vi "LabviewImageProcess - red_tweezers_interface_linegen - test_edited for seq order-10-10 - Copy.vi"() -> ()   [LabVIEW 2015]
doc: "This is the interface, the one VI which loads all the others. Run this one first.\n\n(the line below ensures settings are saved)\n[Red Tweezers Save Settings]"
uses:
  subvis/line_trapping.ctl
  subvis/spot.ctl
  <vilib>/userdefined/High Color/IMAQdx.ctl
  subvis/selection_element.ctl
  subvis/mouse_info.ctl
  <vilib>/Analysis/baseanly.llb/Real A x B.vi
  subvis/red_tweezers_globals_INTERNAL_VOLATILE.vi
  subvis/red_tweezers_globals.vi
  <vilib>/Analysis/NI_AALBase.lvlib
  <vilib>/vision/driver/NI_Vision_Acquisition_Software.lvlib
  <vilib>/vision/NI_Vision_Development_Module.lvlib
panel:
  out "Spot Storage":T1[](array[typedef]) {"Amplitude Correction" step=0.1; "Line Trapping"."Phase Gradient" step=0.05; "Line Trapping"."Vector"."x" step=1e-06 format="%#_6p"; "Line Trapping"."Vector"."y" step=1e-06 format="%#_6p"; "Line Trapping"."Vector"."z" step=1e-06 format="%#_6p"; "NA Position"."r" step=1e-06; "NA Position"."y" step=1e-06; "NA Position"."x" step=1e-06; "Position"."z" step=1e-06; "Position"."y" step=1e-06; "Position"."x" step=1e-06; "Phase" step=0.7753; "Intensity" step=0.1}
  out "# selected":i16
  out "Last Pattern":T1[](array[typedef]) {"Amplitude Correction" step=0.1; "Line Trapping"."Phase Gradient" step=0.05; "Line Trapping"."Vector"."x" step=1e-06 format="%#_6p"; "Line Trapping"."Vector"."y" step=1e-06 format="%#_6p"; "Line Trapping"."Vector"."z" step=1e-06 format="%#_6p"; "NA Position"."r" step=1e-06; "NA Position"."y" step=1e-06; "NA Position"."x" step=1e-06; "Position"."z" step=1e-06; "Position"."y" step=1e-06; "Position"."x" step=1e-06; "Phase" step=0.7753; "Intensity" step=0.1}
  out "Plugins":T3(array[cluster])=[{"Name"="ASI Stage", "Folder"=path "C:/Users/Richard Bowman/Dropbox/red_tweezers_1_4_rc4/plugins/ASI Stage.llb", "vi reference"=refnum, "Needs to be run"=TRUE, "Error"={"status"=FALSE, "code"=0, "source"=""}}, {"Name"="iTweezers", "Folder"=path "C:/Users/Richard Bowman/Dropbox/red_tweezers_1_4_rc4/plugins/iTweezers.llb", "vi reference"=refnum, "Needs to be run"=TRUE, "Error"={"status"=FALSE, "code"=0, "source"=""}}, {"Name"="MightexLED", "Folder"=path "C:/Users/Richard Bowman/Dropbox/red_tweezers_1_4_rc4/plugins/MightexLED.llb", "vi reference"=refnum, "Needs to be run"=TRUE, "Error"={"status"=FALSE, "code"=0, "source"=""}}]
  in  "Tab":T4(tab)
  out "Y":dbl
  out "X":dbl
  in  "O Button":bool
  in  "OK Button":bool
  in  "Bubble Size":dbl=50.0002
  out "Hit Indicator":bool
  in  "On":bool
  out "Induce check":bool
  out "Area+ Buffer":dbl
  in  "Area to check":dbl=0.00025
  out "Prev Current Spot":dbl
  out "spots selected 2":i32=4
  out "Spot # Check":dbl
  out "Orig Y SC":dbl
  out "Orig X SC":dbl
  out "ID num check":dbl
  out "Value Check":dbl
  out "ID":dbl[](array[numeric])
  out "Null array":dbl[](array[numeric])
  out "Potential Collisions":dbl
  out "What to Check":dbl[](array[numeric])
  out "String counter":dbl
  out "Counter for String":dbl
  out "Numeric 4":dbl
  out "LCounter":dbl
  out "Numeric 3":dbl
  out "Num":dbl
  out "Old Y":dbl
  out "Old X":dbl
  out "init":dbl
  out "Looper":bool
  in  "Output to SLM":bool
  out "Maximum":dbl
  out "Projected Distance":dbl
  out "Previous Distance":dbl
  out "Group ID #":dbl
  in  "Buffer Zone":dbl=7e-05
  out "# of Spots":dbl
  out "Distance":dbl
  out "Hit":bool
  out "Y Displacement":dbl
  out "X Displacement":dbl
  out "Current Spot #":dbl
  out "spots selected":i32=4
  in  "lock aspect ratio":bool=TRUE
  in  "Size":cluster{"x":dbl, "y":dbl, "z":dbl} {"z" step=1e-06 format="%#_4p"; "y" step=1e-06 format="%#_4p"; "x" step=1e-06 format="%#_4p"}
  in  "Position":cluster{"x":dbl, "y":dbl, "z":dbl}={"x"=1e-06, "y"=-6.3e-06, "z"=0.0} {"z" step=1e-06 format="%#_4p"; "y" step=1e-06 format="%#_4p"; "x" step=1e-06 format="%#_4p"}
  in  "phase":dbl step=0.7753
  in  "Vortex Charge":i8
  in  "Intensity":dbl=1.0 step=0.1
  in  "add to selection":bool
  in  "random position":bool
  in  "new spot":bool
  in  "delete":bool
  in  "rotate":bool
  in  "Rotation Axis":u16(ring)=2 items=["Z", "X", "Y", "Custom"]
  in  "Angle (degrees)":dbl=2.0
  in  "Custom Axis":cluster{dbl, dbl, dbl}
  in  "Spot Shape":enum32{"Normal", "Line", "NA", "Mixed"}(tab)=enum."Mixed"
  in  "Line Trapping":T2 {"Phase Gradient" step=0.05; "Vector"."x" step=1e-06 format="%#_4p"; "Vector"."y" step=1e-06 format="%#_4p"; "Vector"."z" step=1e-06 format="%#_4p"}
  in  "Scale back aperture":dbl=1.1 step=0.1
  in  "Scale BA":bool
  in  "Position on back aperture":cluster{"x":dbl, "y":dbl}={"x"=-5.84327907697451e-18, "y"=0.0} {"y" step=0.1 format="%#_4p"; "x" step=0.1 format="%#_4p"}
  in  "Radius on back aperture":dbl=1.1 step=0.1
  in  "Generate":bool
  in  "Pattern":T5(tab)
  in  "Spots across centre":i32=5
  in  "Reference Array?":bool
  in  "Fraction of SLM":dbl=1.0
  in  "Spots across centre":i32=5
  in  "N":cluster{i32, i32}
  in  "spacing/m":dbl=2.0
  in  "Iterations":i32=10
  out "non-uniformity":dbl(slide)=0.031119223416512406 scale=0.0..0.2
  out "efficiency":dbl(slide)=0.8985936267644501 scale=0.0..1.0
  in  "Optimise":bool
  in  "Reset Phase/Amplitude":bool
  in  "Fall-off/m":dbl=0.00025 min=0.0 step=1e-06 format="%#_4p"
  in  "Abort Plugin":bool
  in  "Plugin:":u16(ring)=1 items=["ASI Stage", "iTweezers", "MightexLED"]
  in  "Save Video":bool
  in  "Global ROI (requires restart)":i32[](array[numeric])=[0, 0, 1280, 512]
  in  "Zoom":bool
  in  "Draw ROI":bool
  in  "Zoom to Fit":bool
  out "Image Information":string="640x480 1.93X 8-bit image 255    (0,0)"
  in  "Camera":T6
  in  "Time per Frame (ms)":dbl
  in  "Edit Sequence Mode":bool
  in  "Manual Edit":bool
  in  "Bubble ID to Empty":dbl
  in  "Clearance Button":bool
  in  "Manual Sequence":bool
  in  "Play Sequence":bool
  in  "Reset":bool
  out "Sequence Instances":dbl
  out "Counter":dbl
  in  "Save State":bool
  out "Sequence On?":bool
  in  "Sequence Order":dbl
  out "Selection/Group":T7[](array[typedef])
  in  "Sequence Storer":T1[][](array[typedef]) {"Amplitude Correction" step=0.1; "Line Trapping"."Phase Gradient" step=0.05; "Line Trapping"."Vector"."x" step=1e-06 format="%#_6p"; "Line Trapping"."Vector"."y" step=1e-06 format="%#_6p"; "Line Trapping"."Vector"."z" step=1e-06 format="%#_6p"; "NA Position"."r" step=1e-06; "NA Position"."y" step=1e-06; "NA Position"."x" step=1e-06; "Position"."z" step=1e-06; "Position"."y" step=1e-06; "Position"."x" step=1e-06; "Phase" step=0.7753; "Intensity" step=0.1}
  in  "Rates":bool
  out "Rates":dbl
  out "LCS":dbl
  in  "Add Additional Frames":bool
  in  "Frame Location":dbl
  in  "Additional Frames Wanted":dbl
  in  "Initiate Creation":bool
  in  "Number of Planned Sequence Frames":dbl
  in  "Max Number of Bubbles":dbl
  in  "Tab Control":enum32{"Line", "Arc"}(tab)
  out "X Rate":dbl
  out "Y Rate":dbl
  out "Degree Rate":dbl
  out "Radians":dbl
  out "Center Y":dbl
  out "Center X":dbl
  in  "Radius X":dbl
  in  "Theta":dbl
  in  "Lock Current Spot":bool
  out "Locked Current Spot":dbl
  out "Numeric":dbl
  out "probe":dbl
  in  "Insert":bool
  in  "Start at Which Frame?":dbl
  out "Original Y":dbl
  out "Original X":dbl
  in  "Mark Original Position":bool
  in  "How Many Frames?":dbl
  out "New Y":dbl
  out "New X":dbl
  out "Spot Storage 2":T1[](array[typedef]) {"Amplitude Correction" step=0.1; "Line Trapping"."Phase Gradient" step=0.05; "Line Trapping"."Vector"."x" step=1e-06 format="%#_6p"; "Line Trapping"."Vector"."y" step=1e-06 format="%#_6p"; "Line Trapping"."Vector"."z" step=1e-06 format="%#_6p"; "NA Position"."r" step=1e-06; "NA Position"."y" step=1e-06; "NA Position"."x" step=1e-06; "Position"."z" step=1e-06; "Position"."y" step=1e-06; "Position"."x" step=1e-06; "Phase" step=0.7753; "Intensity" step=0.1}
  in  "Save":bool
  in  "Load":bool
  in  "Camera Capture":bool
  out "Bubble y":dbl
  out "Bubble x":dbl
  out "Number of Matches Returned":dbl
  out "bottomry":dbl
  out "toply":dbl
  out "bottomrx":dbl
  out "toplx":dbl
  in  "Send Data":bool
  out "Camera 2":T8(plugin-control)
  out "Circles":T9(array[cluster]) {"Position"."Y" format="%.2f"; "Position"."X" format="%.2f"}
  out "Video Frame Rate":dbl(knob)=50.00000000000003 scale=0.0..100.0 scale format="%.1f"
  out "Interface Frame Rate":dbl(knob)=97.23240312927678 scale=0.0..100.0 scale format="%.1f"
  in  "stop":bool=TRUE
  out "1 for original positon":dbl
  out "MOP pressed":bool
  out "MOP pressed After":bool
  out "X Pos every 10 sec":dbl
  out "Elapsed Time":dbl
  out "Sequence Frames To Check":string
  out "Position Indicator":string
  in  "Clear String":bool
  out "String 2":string
  out "Collision Detector":string
  out "Array":dbl[](array[numeric])
  out "Spot Checker":T1[](array[typedef]) {"Amplitude Correction" step=0.1; "Line Trapping"."Phase Gradient" step=0.05; "Line Trapping"."Vector"."x" step=1e-06 format="%#_6p"; "Line Trapping"."Vector"."y" step=1e-06 format="%#_6p"; "Line Trapping"."Vector"."z" step=1e-06 format="%#_6p"; "NA Position"."r" step=1e-06; "NA Position"."y" step=1e-06; "NA Position"."x" step=1e-06; "Position"."z" step=1e-06; "Position"."y" step=1e-06; "Position"."x" step=1e-06; "Phase" step=0.7753; "Intensity" step=0.1}
  out "Image":T8(plugin-control)
  # "Notes:\n\nIf you are doing non-sequence controls,\nthe delete function can be used as intended.\nHowever, do not use the delete function after\nrunning a sequence! Using it will prevent\nthe bubbles from appearing as the\nnumber of spots will change, which is\nessential for the sequence to work (it would\nbe displaying the maximum number of\nbubbles). \n\nIf you happen to delete a bubble, it can be \nrestored by inserting a new spot. Once enough\nspots have been restored, click on manual edit\nto correct the # of spots tracker. It should \nbe restored to where it originally was."
  # "The SLM can be used to shape spots; here you can restrict the NA of a spot (so it comes only from part of the back aperture), or create a line-trap"
  # "The traps do not have any spot-shaping applied (so they should just be diffraction-limited focal spots)."
  # "This shapes the amplitude (and phase) of the beam to create extended line traps.  The \"Phase Gradient\" control allows the Poynting vector to push things along the line.  Unfortunately, some work is needed on the scaling factors so the phase gradient control will need tweaking if the line trap has a nonzero z component."
  # "By default,each spot comes from the whole back aperture.  Here, you can limit a spot to come from a specific part of the back aperture."
  # "The control below allows you to scale the whole back aperture (i.e. the position and size of all the apertures).  It's a one-time operation, i.e. only changes things when you push \"ok\"."
  # "A Combination of line-trapping and NA restriction has been applied to these traps.  You can get at the line trap or NA parameters on the other tabs, switching to the NA tab does not delete the line-trap settings."
  # "This tab generates Shack-Hartmann type holograms, which are often useful when aligning the system, and arrays of spots."
  # "The controls above only work when using the \"IMAQdx with ROI Buttons\" case in the bottom loop.  You can save video regardless of camera code though."
  # "Manual Edit allows a user to\ngo to a specific sequence frame."
  # "To clear the sequence, you must\nclear the array. Right click on sequence\nstorer to do this."
  # "Use this to \"clear\" a \nspecific bubble. If\nworking on a sequence,\nuse this as your delete\nbutton! You can update\nthe view by using manual edit."
  # "Use the reset button\nto clear counter.\nIt becomes necessary\nwhen you clear the array,\nespecially in manual mode."
  # "Use the sequence creator tab to specify the\nnumber of bubbles you want along with\nthe number of frames.\n\nTo save at a specific interval, the sequence\norder can be used to place the state. If used\nto correct something, it will replace the\nentire sequence frame.\n\n\"Sequence On?\" is only used in auto mode."
  # "Frame Location must be\nwhere you want to add\nthe frames to (ie having \n4 as an input would have\nthe additional frames\nstart at array row 5."
  # "Multiple bubbles can  be done with the\nline function. One bubble at a time for the arc\nfunction."
  # "Using the Load/Save function:\n\nRed Tweezers itself is unable to save long \nsequences, but a separate program is able to\naccomplish this. To do this, follow these\nsteps:\n\n1. After creating your sequence, press the save\nbutton below.\n\n2. Then, go to the subvi folder and find\nSequenceSaver.vi.\n\n3. At the control \"Sequence Storer,\" right-click\nthe dimensions part of the array and go to\ndata operations.\n\n4. Press \"Make Current Values Default\" and save\nthe sequence.\n\n5. The next time you load the program, simply\npress load to re-acquire the sequence. You\nwill need to insert the bubbles again, but after\nthe first frame can be recovered by using\nSequenceControl.vi."
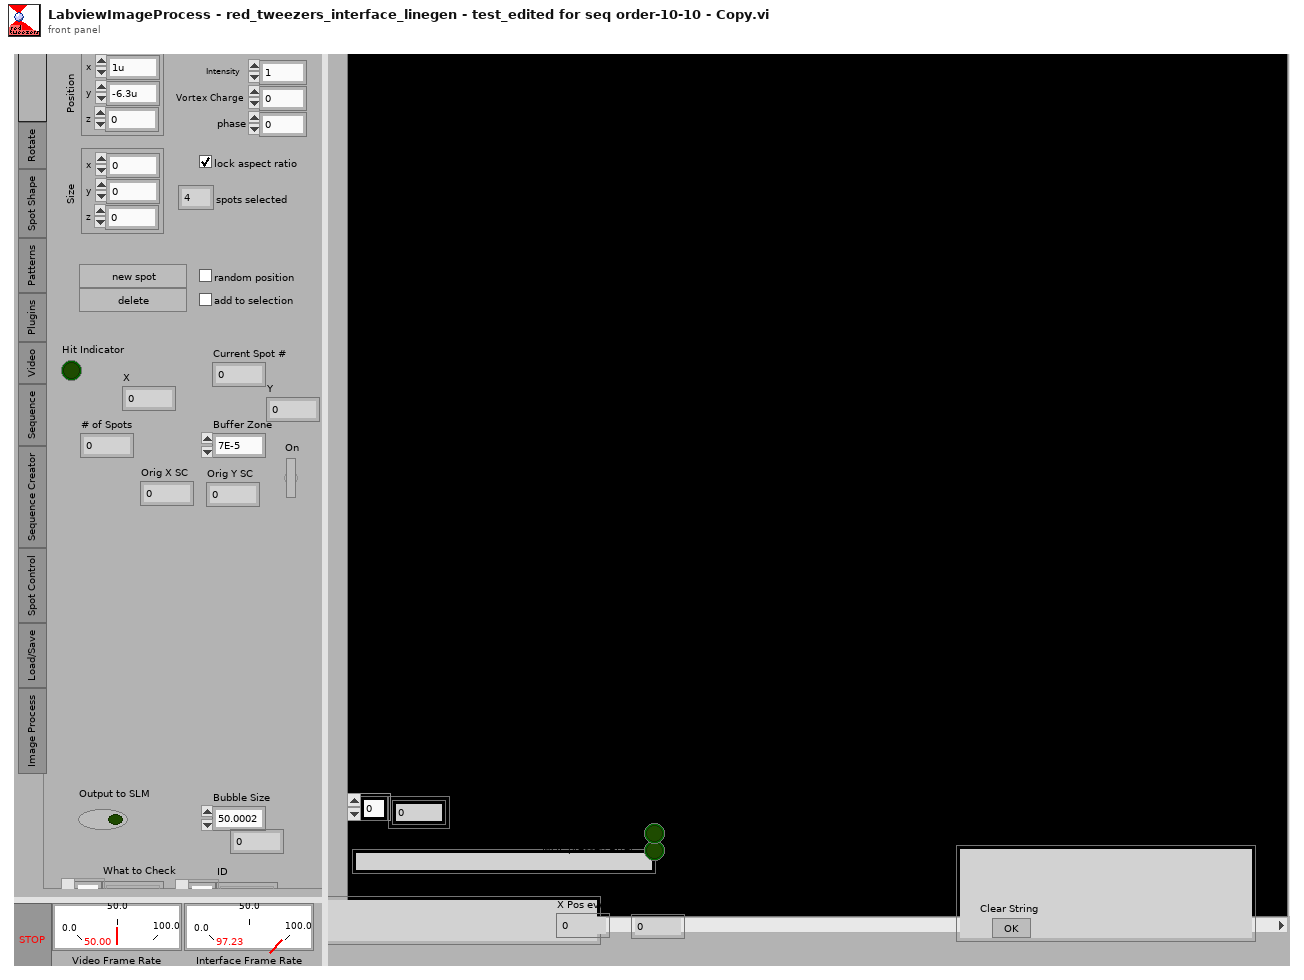
[diagram p1: front panel]
types:
  T1 = typedef "spot.ctl" = cluster{"Position":cluster{"x":dbl, "y":dbl, "z":dbl}, "Intensity":dbl, "Vortex Charge":i8, "Phase":dbl, "NA Position":cluster{"x":dbl, "y":dbl, "r":dbl}, "Line Trapping":T2, "Amplitude Correction":dbl}
  T2 = typedef "line_trapping.ctl" = cluster{"Vector":cluster{"x":dbl, "y":dbl, "z":dbl}, "Phase Gradient":dbl}
  T3 = cluster{"Name":string, "Folder":path, "vi reference":refnum<vi>, "Needs to be run":bool, "Error":errorcluster}[]
  T4 = enum32{"Current Spot", "Rotate", "Spot Shape", "Patterns", "Plugins", "Video", "Sequence", "Sequence Creator", "Spot Control", "Load/Save", "Image Process"}
  T5 = enum32{"HCP Shack-Hartmann", "Square Shack-Hartmann", "Rectangular Grid"}
  T6 = typedef "IMAQdx.ctl" = refnum<k21>
  T7 = typedef "selection_element.ctl" = cluster{"Group ID":i32, "Selected":bool}
  T8 = typedef "IMAQ Image.ctl" = refnum<image>
  T9 = cluster{"Position":cluster{"X":sgl, "Y":sgl}, "Radius":dbl, "Score":dbl}[]
  T10 = typedef "mouse_info.ctl" = cluster{"Button Down":bool, "Dragging":bool, "Position (Image Pixels)":cluster{"X":dbl, "Y":dbl}, "Previous Position (Image Pixels)":cluster{"X":dbl, "Y":dbl}, "Button":u16, "Mods":cluster{"Double Click":bool, "Menu Key":bool}, "PlatMods":cluster{"Shift":bool, "Ctrl":bool, "Alt":bool, "Cmd":bool, "Opt":bool}}
  T11 = cluster{"Position":cluster{"x":dbl, "y":dbl, "z":dbl}, "Intensity":dbl, "Vortex Charge":i8, "Phase":dbl, "NA Position":cluster{"x":dbl, "y":dbl, "r":dbl}, "Line Trapping":T2, "Amplitude Correction":dbl}
  T12 = enum16{"Set guide visibility", "Set grid visibility", "Show front panel", "Render on image"}
  T13 = enum32{"Current Spot", "Rotate", "Spot Shape", "Patterns", "Plugins", "Video"}
  T14 = enum16{"Left Button", "Center Button", "Right Button", "Window Close"}
  T15 = typedef "Image Type" = u32
  T16 = cluster{"number: 0 to 1":dbl, "number: 0 to 1":dbl}
  T17 = typedef "NI_Matrix.lvlib/RealMatrix.ctl" = dbl[][]
  T18 = typedef "overlay_element.ctl" = cluster{"Tool":enum16{"Lines", "Oval", "Rectangle", "Text"}, "Points":cluster{"X":dbl, "Y":dbl}[], "Drawing Mode":u32, "Color":u32, "String":string}
  T19 = enum32{"Current Spot", "Rotate", "Spot Shape", "Patterns", "Plugins", "Video", "Particle Tracking", "Clamping", "Blank"}[]
  T20 = typedef "LVMenuShortCut.ctl" = cluster{"include Shift key?":bool, "include Ctrl key?":bool, "shortcut key":string}
  T21 = typedef "LVPoint32TypeDef.ctl" = cluster{"Horizontal":i32, "Vertical":i32}
  T22 = cluster{"Shift":bool, "Ctrl":bool, "Alt":bool, "Cmd":bool, "Opt":bool}
  T23 = cluster{"Button Down":bool, "Dragging":bool, "Mouse Coords (image pixels)":cluster{dbl, dbl}, "Mouse Coords (image pixels)":cluster{dbl, dbl}, "Button":u16, "Mods":cluster{"Double Click":bool, "Menu Key":bool}, "PlatMods":cluster{"Shift":bool, "Ctrl":bool, "Alt":bool, "Cmd":bool, "Opt":bool}}
  T24 = cluster{"Position":cluster{"X":sgl, "Y":sgl}, "Radius":dbl, "Score":dbl}
  T25 = cluster{"[0]":dbl, "[1]":dbl, "[2]":dbl, "[3]":dbl}
  T26 = cluster{"Average Frame Time":dbl, "millisecond timer value":u32}
  T27 = cluster{"Position":cluster{"x":dbl, "y":dbl, "z":dbl}, "Intensity":dbl, "Vortex Charge":i8, "Phase":dbl, "NA Position":cluster{"x":dbl, "y":dbl, "r":dbl}, "Line Trapping":T2, "Amplitude Correction":dbl}[]
  T28 = enum32{"Bad", "Idle", "Run top level", "Running"}
  T29 = typedef "AviRefnum.ctl" = refnum<k1>
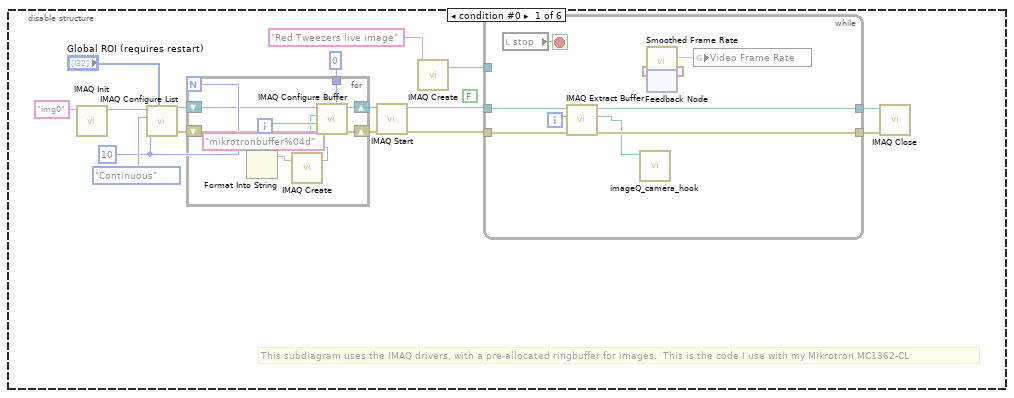
[diagram p3: hidden frame]
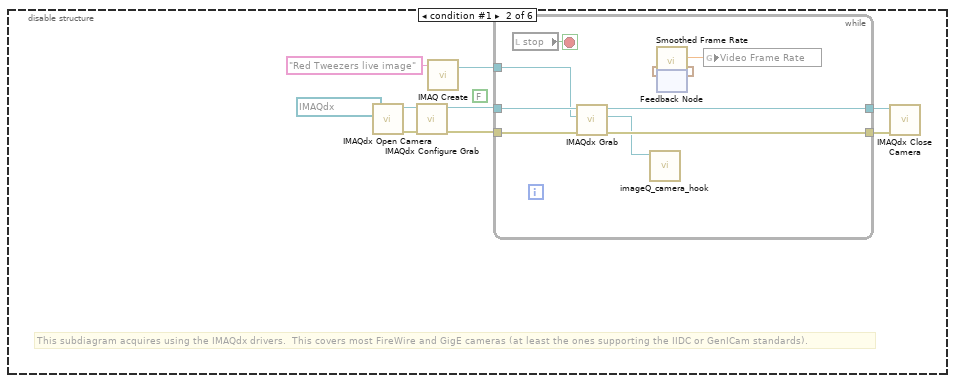
[diagram p4: hidden frame]
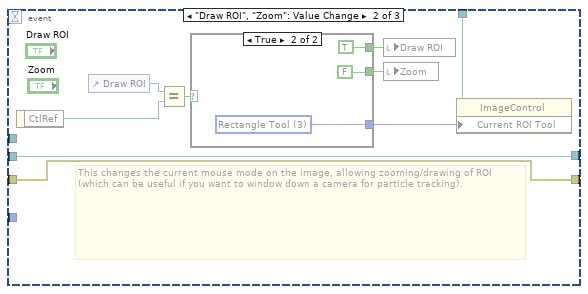
[diagram p5: hidden frame]
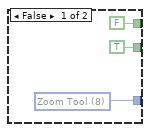
[diagram p6: hidden frame]
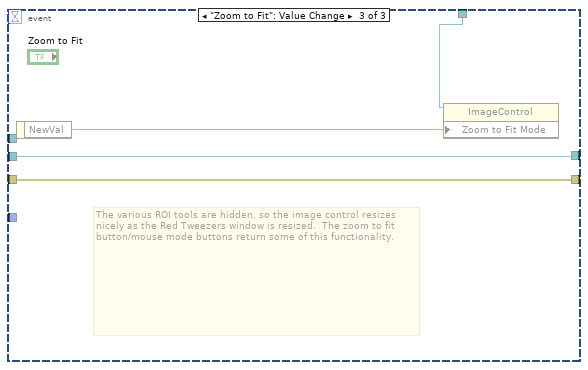
[diagram p7: hidden frame]
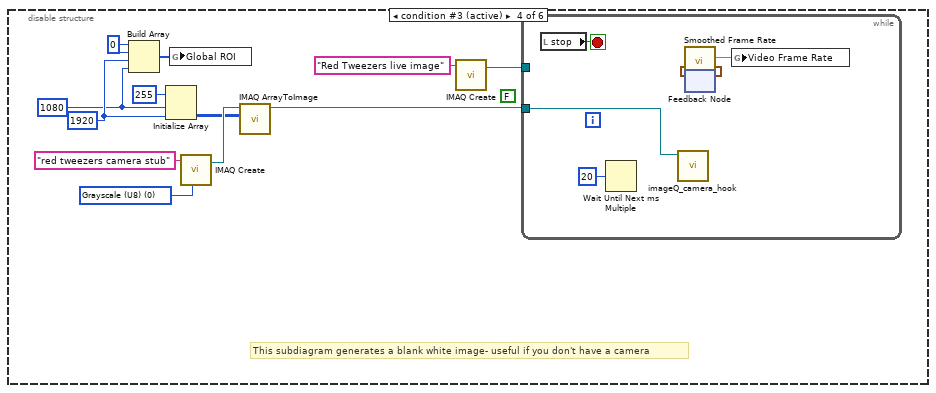
[diagram p8: hidden frame]
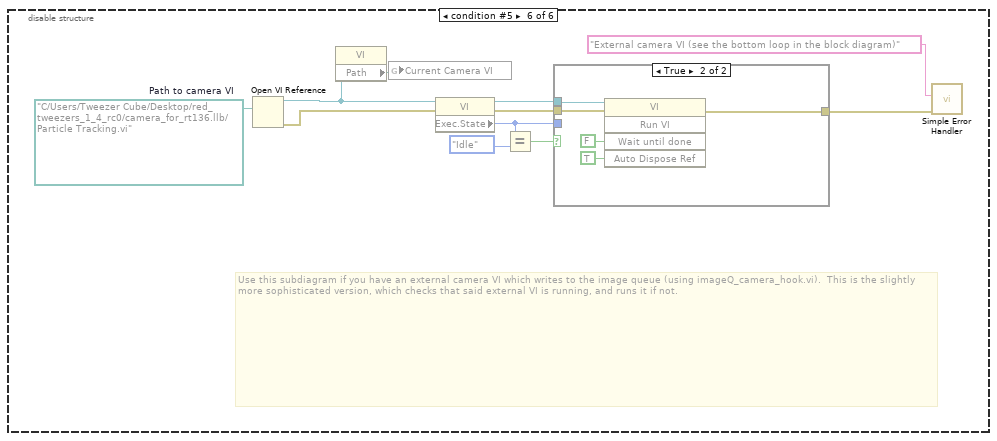
[diagram p10: hidden frame]
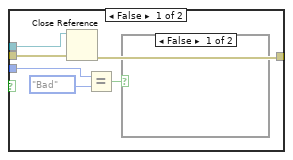
[diagram p11: hidden frame]
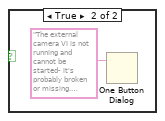
[diagram p12: hidden frame]
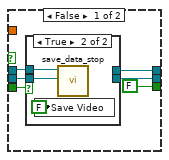
[diagram p13: hidden frame]
diagram:
  w11 = "red_tweezers_display_imageQ" ("Queue Name")
  w23 = T10 {"Button Down"=FALSE, "Dragging"=FALSE, "Position (Image Pixels)"={"X"=0.0, "Y"=0.0}, "Previous Position (Image Pixels)"={"X"=0.0, "Y"=0.0}, "Button"=0, "Mods"={"Double Click"=FALSE, "Menu Key"=FALSE}, "PlatMods"={"Shift"=FALSE, "Ctrl"=FALSE, "Alt"=FALSE, "Cmd"=FALSE, "Opt"=FALSE}}  # Mouse Information
  w24 = refnum<vi> refnum  # Image
  # "The funny looking feedback-node structure is deliberate (if odd).  We want to reload settings from the last used file (stored in the registry) only if this program has not been run since it was last loaded from file/recompiled.  That's why I use an uninitialised shift register: every time the program runs, it increments.  So, if it is zero, this is our first run (or we've been recently recompiled)."
  # "This loop handles the video that is displayed on-screen and saved to file."
  # "Initially, we only register to be told when the user clicks the image"
  # "This is the actual image control"
  # "This is a generic reference.\nIt is just a placeholder, so we can register for events later."
  # "This version of red tweezers uses two coordinate systems: \n1. Real Coordinates - corresponding to physical distances in 3D in microns\n2. Image Coordinates - position on the camera image, relative to the top left of the CURRENT ROI, measured in pixels. If the ROI changes, the relationship between \"real units\" and \"image pixels\" may change, so all values should be stored and presented to the user in REAL units unless there is a good reason to do otherwise."
  n1 = control-ref of="Plugin Pnl"() -> (w20:refnum<vi>)
  n2 = flat-sequence {
    tunnel: [w27] -> w6
    tunnel: w4 -> [_]
    frame #0 {
      n3 = vi-ref "red_tweezers_globals_INTERNAL.vi"() -> (w28:refnum<vi>)
      n4 = property class="VI"(reference=w28) -> ("Path"=w27:path)  [unwired: 1 in, 2 out]
      n5 = global write "red_tweezers_globals_INTERNAL_VOLATILE.vi" "Current Camera VI"(w27) -> ()
    }
  }
  n6 = control-ref of="Plugin:"() -> (w21:refnum<vi>)
  n7 = feedback #1() -> (w14:dbl)  [unwired: 1 in]
  n8 = Equal To 0?(x=w14) -> (x = 0?=w13:bool)
  n9 = Increment(x=w14) -> (x+1=w12:dbl)
  n10 = feedback-in #1(w12) -> ()
  n11 = call "plugins_load.vi"("Sub Panel"=w20, "Plugin Chooser"=w21) -> ("error out"=w15:errorcluster, "Plugins"=w17:T3)  [unwired: 2 in, 2 out]
  "Plugins" <- w17
  n12 = control-ref of="Image"() -> (w5:refnum<vi>)
  n13 = case shown="True" w13 {
    tunnel: w15 -> [_ w29]
    tunnel: [_ w29] -> w4
    frame False {
    }
    frame True {
      n14 = call "settings_load_default_file.vi"("error out"=w29) -> ()
    }
  }
  n15 = flat-sequence {
    tunnel: w4 -> [_]
    tunnel: w2 -> [w31]
    frame #0 {
      # "ensure we don't accidentally start saving video, and run UDP Sender to set up the hologram window."
      n16 = local write "Save Video"(FALSE ("background subtraction")) -> ()
      n17 = call "UDP Sender generic_2.vi"("Spots"=w31) -> ()  [unwired: 2 in, 1 out]
    }
  }
  n18 = global read "red_tweezers_globals.vi" "Selection/Group"() -> (w22:T7[])
  n19 = register-events(w5, w24, w24, w24) -> (reference out=w25:refnum<event-registration>)  [unwired: 2 in, 1 out]
  n20 = global read "red_tweezers_globals.vi" "Spots"() -> (w2:T1[])
  n21 = local write "stop"(FALSE ("STOP")) -> ()
  n22 = call "ensure_selection_matches_spots.vi"("Selection and Groups in"=w22, "Spots"=w2) -> ("Selection and Groups out"=w26:T7[], "Spots (duplicate)"=w1:T1[])  [unwired: 4 in]
  n23 = call "IMAQ Create"("Image Name"=w11) -> ("New Image"=w9:T8)  [unwired: 4 in, 1 out]
  n24 = call "imageQ_create_return_queue.vi"("Queue Name"=w11) -> ("queue out"=w10:refnum<queue>)
  n25 = while {
    shift-right: [w118] -> _
    shift-left: w1 -> [w138]
    shift-right: [w137] -> _
    shift-left: w26 -> [w136]
    shift-right: [w140] -> _
    shift-left: _ -> [w131]
    shift-right: [w139] -> _
    shift-left: _ -> [w130]
    tunnel: w5 -> [w135]
    shift-right: [w129] -> _
    shift-left: w23 -> [w128]
    shift-right: [w132] -> _
    shift-left: w25 -> [w133]
    border: errorcluster {"status"=FALSE, "code"=0, "source"=""} ("error out") -> [_]
    tunnel: [errorcluster {"status"=FALSE, "code"=0, "source"=""} ("error in (no error)")] -> w18
    border: w17 -> [_]
    tunnel: w1 -> [w119]
    stop <- w120 stop-if-true
    w34 = 1
    w42 = 7 items=["Red", "Green", "Blue", "Hue", "Saturation", "Luminance", "Value", "Intensity"] ("Color Plane")
    w46 = T15 0 items=["Grayscale (U8)", "Grayscale (I16)", "Grayscale (SGL)", "Complex (CSG)", "RGB (U32)", "HSL (U32)", "RGB (U64)", "Grayscale (U16)"] ("Image Type")
    # "Don't Need. For Matlab Part."
    # "The function inserts the newly generated sequence for the automatic sequence generator. It also contains the code\nthe code necessary to check whether the bubbles will intersect with each other in the sequence."
    # "This calculates the size of the area including the buffer zone length.\nThe bubble diameter will also be included in the near future."
    # "The statement to the right controls the area that are being chcecked and checks\nwhich bubbles need to be checked.  There are two instances where this activates\nin this case:\n\nWhen a new bubble is selected\nWhen a bubble is deselected, reverting to the last current spot #\n\nThe other case, when the bubble moves out of the area specified, is located\ninside the while loop controlling the bubble movement with a mouse."
    # "Timer function example"
    # "These functions help with the calculations for the sequence generator."
    # "This loads the sequence from the \"saver\" VI. The save function below \"saves\" the sequence into the saver VI."
    # "The VI above is SequenceSaver.vi which contains the\ncode necessary to create a sequence."
    # "This case structure is the Save State structure. This stores\nthe current state of the bubbles (ie position)."
    # "Reset sets the counter back to zero. This is particularly useful \nwhen using the manual sequence."
    # "This case structure helps to continue the sequence.\nThis takes the true case of the Sequence On? function\nor the true case for the Manual Sequence function\nin order to go to the next sequence frame."
    # "This case structure allows for the playing of the sequence.\nThe amount of time it takes to go through the sequence\ncan be edited on the current spot menu."
    # "We only write to the image overlay when we are in one of the tabs, to prevent it disappearing when we are (for example) using the mouse."
    # "These wires control saving undo info. See the VI below's tip strips for details."
    # "Setting these wires to false means:\n(1) dragging moves the selection\n(2) clicking spots changes selection\nset them to true to stop the default mouse behaviour, don't wire them straight through!"
    n26 = event shown="[6] <Image>: Mouse Move" {
      selector: w133 -> [w550 w1222 w1227 w1449 w1477 w1494 w1591 _]
      dyn-events: [w550 w1221 w1227 w1447 w1474 w1495 w1591 _] -> w132
      timeout: 0 -> [_ _ _ _ _ _ _ _]
      tunnel: [w558 _ w1229 w1444 w1479 w1486 w1578 _] -> w140
      tunnel: [w557 _ w1228 w1443 w1478 w1485 w1582 _] -> w139
      tunnel: [w556 _ _ _ _ _ _ _] -> w91
      tunnel: w138 -> [w555 w1217 w1234 w1439 w1472 w1491 w1586 w1909]
      tunnel: [w554 w1217 w1232 w1439 w1472 w1482 w1584 w1909] -> w126
      tunnel: [w553 w1216 w1231 w1428 w1471 w1492 w1574 w1908] -> w125
      tunnel: w136 -> [w552 w1216 w1233 w1428 w1471 w1490 w1585 w1908]
      tunnel: w135 -> [w551 w1218 w1224 w1438 w1475 w1493 w1587 _]
      tunnel: [w549 _ w1226 w1448 T10 {"Button Down"=FALSE, "Dragging"=FALSE, "Position (Image Pixels)"={"X"=0.0, "Y"=0.0}, "Previous Position (Image Pixels)"={"X"=0.0, "Y"=0.0}, "Button"=0, "Mods"={"Double Click"=FALSE, "Menu Key"=FALSE}, "PlatMods"={"Shift"=FALSE, "Ctrl"=FALSE, "Alt"=FALSE, "Cmd"=FALSE, "Opt"=FALSE}} T10 {"Button Down"=FALSE, "Dragging"=FALSE, "Position (Image Pixels)"={"X"=0.0, "Y"=0.0}, "Previous Position (Image Pixels)"={"X"=0.0, "Y"=0.0}, "Button"=0, "Mods"={"Double Click"=FALSE, "Menu Key"=FALSE}, "PlatMods"={"Shift"=FALSE, "Ctrl"=FALSE, "Alt"=FALSE, "Cmd"=FALSE, "Opt"=FALSE}} w1590 _] -> w129
      tunnel: w128 -> [w549 _ w1226 _ _ w1489 w1581 _]
      tunnel: w131 -> [_ _ w1229 w1444 w1479 w1486 w1578 _]
      tunnel: w130 -> [_ _ w1228 w1443 w1478 w1485 w1582 _]
      tunnel: [w548 _ _ _ _ _ _ _] -> w127
      tunnel: [_ _ w1225 _ _ _ TRUE _] -> w124
      tunnel: [_ _ _ TRUE TRUE TRUE FALSE _] -> w123
      tunnel: [TRUE _ _ _ _ _ _ _] -> w121
      tunnel: [_ _ _ _ _ _ _ "stop"] -> w120
      tunnel: w119 -> [_ _ _ _ _ _ w1575 _]
      event Timeout {
        n27 = event-data() -> ()  [unwired: 1 in, 1 out]
        n28 = case shown="\"Current Spot\", Default" "Tab" {
          tunnel: [w574 w842 w989 w1091 w1172 w1210] -> w554
          tunnel: w555 -> [w571 w844 w990 w1093 w1172 w1210]
          tunnel: w552 -> [w560 w843 w987 w1092 w1171 w1209]
          tunnel: [w573 w841 w988 w1090 w1171 w1209] -> w553
          tunnel: [w561 _ TRUE _ _ _] -> w558
          tunnel: [w561 _ _ _ _ _] -> w557
          tunnel: [_ _ _ FALSE _ _] -> w556
          tunnel: w551 -> [_ _ _ _ _ w1206]
          tunnel: w549 -> [_ _ w969 _ _ _]
          tunnel: [_ _ w971 _ _ _] -> w548
          frame "Current Spot", Default {
            w561 = FALSE
            # "The function below contains the code necessary to use the automatic sequence generator to create specific movements. It also helps translate cases where the point is entered in not dragged.\nThis prevents bubbles from intersecting if the bubble is told not to intersect."
            # "If it's out of date, update front panel"
            n29 = call "find_centroid.vi"("Selection and Groups"=w560, "Spots"=w571) -> ("Mean Values"=w569:T1, "size"=w563:cluster{"x":dbl, "y":dbl, "z":dbl}, "centroid"=w564:cluster{"x":dbl, "y":dbl, "z":dbl}, "# selected"=w562:i16)  [unwired: 2 in, 1 out]
            n30 = stacked-sequence {
              tunnel: w562 -> [_ w576]
              frame #0 {
                n31 = local read "spots selected"() -> (→"spots selected 2":i32)
              }
              frame #1 {
                "spots selected" <- w576
              }
            }
            n32 = feedback-in #2(w569) -> ()
            n33 = feedback #2() -> (w570:T1)  [unwired: 1 in]
            n34 = feedback #3() -> (w568:cluster{"x":dbl, "y":dbl, "z":dbl})  [unwired: 1 in]
            n35 = feedback-in #3(w563) -> ()
            n36 = Not Equal?(x=w570, y=w569) -> (x != y?=w567:bool)
            n37 = Not Equal?(x=w568, y=w563) -> (x != y?=w566:bool)
            n38 = Or(x=w567, y=w566) -> (x .or. y?=w565:bool)
            n39 = case shown="True" w565 {
              tunnel: w569 -> [_ w582]
              tunnel: w563 -> [_ w578]
              frame False {
              }
              frame True {
                n40 = Unbundle By Name(w582) -> ("Position"=w577:cluster{"x":dbl, "y":dbl, "z":dbl}, "Intensity"=w580:dbl, "Vortex Charge"=w579:i8, "Phase"=w581:dbl)
                n41 = local write "Size"(w578) -> ()
                n42 = local write "Vortex Charge"(w579) -> ()
                n43 = local write "Intensity"(w580) -> ()
                n44 = local write "Position"(w577) -> ()
                n45 = local write "phase"(w581) -> ()
                n46 = Unbundle By Name(w577) -> ()  [unwired: 2 out]
              }
            }
            n47 = local write "Selection/Group"(w560) -> ()
            n48 = event shown="[3] \"Position\": Value Change" {
              selector: _ -> [_ _ _ _ _ _ _ _]
              dyn-events: _ -> [_ _ _ _ _ _ _ _]
              timeout: 10 -> [_ _ _ _ _ _ _ _]
              tunnel: w571 -> [w584 w588 w602 w625 w729 w774 w800 w823]
              tunnel: w560 -> [w583 w587 w605 w632 w716 w771 w797 w821]
              tunnel: [w584 w586 w603 w624 w717 w772 w798 w822] -> w574
              tunnel: [w583 w585 w604 w632 w716 w771 w797 w821] -> w573
              tunnel: w564 -> [_ _ _ _ w728 _ _ _]
              event Timeout {
                n49 = event-data() -> ()  [unwired: 3 out]
              }
              event "delete": Value Change {
                n50 = event-data() -> ()  [unwired: 7 out]
                n51 = call "delete_selected_spots.vi"("Selection/Group 3"=w587, "Spots 3"=w588) -> ("Selection/Group 2"=w585:T7[], "Spots 2"=w586:T1[])  [unwired: 4 in]
              }
              event "new spot": Value Change {
                # "If we're not adding it to the selection, de-select all the other spots"
                n52 = event-data() -> ()  [unwired: 7 out]
                n53 = call "coords_ROI_currentimage.vi"() -> ("Mono ROI"=w589:i32[])
                n54 = case shown="False" "add to selection" {
                  tunnel: w605 -> [w618 w623]
                  tunnel: [w617 w623] -> w600
                  frame False {
                    n55 = for {
                      tunnel: w618 -> [w621] mode=indexing
                      tunnel: [w622] -> w617 mode=indexing
                      n56 = Unbundle(w621) -> ("Group ID"=w620:i32)  [unwired: 1 out]
                      n57 = Bundle(cluster=w621, "Group ID"=w620, "Selected"=FALSE ("Label.Visible")) -> (w622:T7)
                    }
                  }
                  frame True {
                  }
                }
                n58 = Index Array(array=w589) -> (element #1=w595:i32, element #2=w596:i32, element #3=w594:i32, element #4=w593:i32)  [unwired: 4 in]
                n59 = Bundle("Numeric"=w595, "Numeric"=w596) -> (w590:cluster{"Numeric":i32, "Numeric":i32})  [unwired: 1 in]
                n60 = Bundle("Numeric"=w594, "Numeric"=w593) -> (w592:cluster{"Numeric":i32, "Numeric":i32})  [unwired: 1 in]
                n61 = Subtract(x=w592, y=w590) -> (x-y=w591:cluster{"Numeric":i32, "Numeric":i32})
                n62 = case shown="True" "random position" {
                  tunnel: [w607 w613] -> w598
                  tunnel: w591 -> [_ w609]
                  tunnel: w590 -> [_ w608]
                  frame False {
                    n63 = call "replace_position.vi"("Position"=cluster{"x":dbl, "y":dbl, "z":dbl} {"x"=0.0, "y"=0.0, "z"=0.0}) -> ("Spot"=w607:T1)  [unwired: 1 in, 2 out]
                  }
                  frame True {
                    n64 = Random Number (0-1)() -> (number: 0 to 1=w615:dbl)
                    n65 = Random Number (0-1)() -> (number: 0 to 1=w616:dbl)
                    n66 = Bundle("number: 0 to 1"=w616, "number: 0 to 1"=w615) -> (w614:T16)  [unwired: 1 out]
                    n67 = Multiply(x=w614, y=w609) -> (x*y=w611:cluster{dbl, dbl})
                    n68 = Add(x=w611, y=w608) -> (x+y=w610:cluster{dbl, dbl})
                    n69 = call "coords_image_to_real_currentimage.vi"("Position (pixels on image)"=w610) -> ("Position (real coords)"=w612:cluster{dbl, dbl, "Z":dbl})  [unwired: 9 in]
                    n70 = call "replace_position.vi"("Position"=w612) -> ("Spot"=w613:T1)  [unwired: 1 in, 2 out]
                  }
                }
                n71 = Build Array (concatenate)(w602, w598) -> (w603:T1[])
                n72 = Build Array (concatenate)(w600, cluster{i32, "Label.Visible":bool} {0, "Label.Visible"=TRUE}) -> (w604:T7[])
              }
              event "Position": Value Change {
                # "If the position has changed, translate the spots"
                n73 = event-data() -> ("OldVal"=w630:cluster{"x":dbl, "y":dbl, "z":dbl}, "NewVal"=w631:cluster{"x":dbl, "y":dbl, "z":dbl})  [unwired: 5 out]
                n74 = flat-sequence {
                  tunnel: w632 -> [w636]
                  tunnel: w629 -> [w635]
                  tunnel: w625 -> [w634]
                  tunnel: [w633] -> w626
                  frame #0 {
                    n75 = for {
                      tunnel: w634 -> [w641] mode=indexing
                      tunnel: w636 -> [w638] mode=indexing
                      tunnel: [w640] -> w633 mode=indexing
                      tunnel: w635 -> [w639]
                      n76 = Unbundle(w638) -> ("Selected"=w637:bool)  [unwired: 1 out]
                      n77 = case shown="True" w637 {
                        tunnel: w641 -> [w642 w647]
                        tunnel: [w642 w646] -> w640
                        tunnel: w639 -> [_ w643]
                        frame False {
                        }
                        frame True {
                          n78 = call "extract_position.vi"("Spot"=w647) -> ("Position"=w644:cluster{"x":dbl, "y":dbl, "z":dbl})
                          n79 = Add(x=w644, y=w643) -> (x+y=w645:cluster{"x":dbl, "y":dbl, "z":dbl})
                          n80 = call "replace_position.vi"("Position"=w645, "Spot in"=w647) -> ("Spot"=w646:T1)  [unwired: 2 out]
                        }
                      }
                    }
                  }
                }
                n81 = Subtract(x=w631, y=w630) -> (x-y=w629:cluster{"x":dbl, "y":dbl, "z":dbl})
                n82 = local read "# of Spots"() -> (w628:dbl)
                n83 = stacked-sequence {
                  tunnel: w625 -> [_ w652 _]
                  tunnel: w626 -> [_ w651 _]
                  tunnel: w628 -> [_ w650 _]
                  tunnel: [_ _ w699] -> w627
                  tunnel: w626 -> [_ _ w698]
                  tunnel: w625 -> [_ _ w697]
                  tunnel: [_ _ w696] -> w624
                  frame #0 {
                    n84 = local write "Looper"(FALSE) -> ()
                    "init" <- 0
                  }
                  frame #1 {
                    n85 = for {
                      N: w650 -> [_]
                      tunnel: w652 -> [w657]
                      tunnel: w651 -> [w662]
                      stop <- w663 stop-if-true
                      n86 = local read "init"() -> (w656:dbl)
                      n87 = Index Array(array=w662, index=w656) -> (element=w661:T1)
                      n88 = Index Array(array=w657, index=w656) -> (element=w655:T1)
                      n89 = Unbundle By Name(w661) -> ("Position.x"=w660:dbl, "Position.y"=w659:dbl)
                      n90 = local read "# of Spots"() -> (w658:dbl)
                      n91 = Unbundle By Name(w655) -> ("Position.x"=→"Old X":dbl, "Position.y"=→"Old Y":dbl)
                      n92 = local write "New X"(w660) -> ()
                      n93 = local write "New Y"(w659) -> ()
                      n94 = stacked-sequence {
                        tunnel: w657 -> [w668 _]
                        tunnel: w660 -> [w667 _]
                        tunnel: w659 -> [w666 _]
                        tunnel: w658 -> [w665 _]
                        tunnel: w656 -> [w664 _]
                        frame #0 {
                          n95 = for {
                            N: w665 -> [_]
                            tunnel: w668 -> [w690]
                            tunnel: w667 -> [w689]
                            tunnel: w666 -> [w687]
                            tunnel: w664 -> [w672]
                            i -> [w674]
                            stop <- w673 stop-if-true
                            n96 = Index Array(array=w690, index=w674) -> (element=w691:T1)
                            n97 = Unbundle By Name(w691) -> ("Position.x"=w688:dbl, "Position.y"=w686:dbl)
                            n98 = Subtract(x=w689, y=w688) -> (x-y=w685:dbl)
                            n99 = Subtract(x=w687, y=w686) -> (x-y=w684:dbl)
                            n100 = Square(x=w685) -> (x^2=w683:dbl)
                            n101 = Square(x=w684) -> (x^2=w682:dbl)
                            n102 = local read "# of Spots"() -> (w676:dbl)
                            n103 = Add(x=w683, y=w682) -> (x+y=w681:dbl)
                            n104 = local read "Buffer Zone"() -> (w671:dbl)
                            n105 = Square Root(x=w681) -> (sqrt(x)=w680:dbl)
                            n106 = Multiply(x=2, y=w671) -> (x*y=w669:dbl)
                            n107 = Less?(x=w680, y=w669) -> (x < y?=w678:bool)
                            n108 = Not Equal?(x=w672, y=w674) -> (x != y?=w677:bool)
                            n109 = Equal?(x=w676, y=w674) -> (x = y?=w679:bool)
                            n110 = And(x=w677, y=w678) -> (x .and. y?=w675:bool)
                            "Looper" <- w675
                            n111 = Or(x=w675, y=w679) -> (x .or. y?=w673:bool)
                          }
                        }
                        frame #1 {
                          n112 = local read "Looper"() -> (w692:bool)
                          n113 = case shown="False" w692 {
                            frame False {
                              n114 = local read "init"() -> (w693:dbl)
                              n115 = Add(x=w693, y=1) -> (x+y=w695:dbl)
                              n116 = local write "init"(w695) -> ()
                            }
                            frame True {
                            }
                          }
                        }
                      }
                      n117 = local read "Looper"() -> (w663:bool)
                    }
                  }
                  frame #2 {
                    n118 = local read "Looper"() -> (w700:bool)
                    n119 = case shown="False" w700 {
                      tunnel: w698 -> [w704 _]
                      tunnel: w697 -> [_ w712]
                      tunnel: ["This is an acceptable entry." "ERROR: A bubble will intersect the buffer zone."] -> w699
                      tunnel: [w704 w712] -> w696
                      frame False {
                        n120 = local write "Looper"(FALSE) -> ()
                        n121 = local read "Current Spot #"() -> (w705:dbl)
                        n122 = Index Array(array=w704, index=w705) -> (element=w703:T1)
                        n123 = Unbundle By Name(w703) -> ("Position.x"=w702:dbl, "Position.y"=w701:dbl)
                        n124 = local write "New Y"(w701) -> ()
                        n125 = local write "New X"(w702) -> ()
                      }
                      frame True {
                        # "Restore original position"
                        n126 = local write "Looper"(FALSE) -> ()
                        n127 = local read "Old Y"() -> (w709:dbl)
                        n128 = local read "Old X"() -> (w710:dbl)
                        n129 = local read "Position"() -> (w708:cluster{"x":dbl, "y":dbl, "z":dbl})
                        n130 = Bundle By Name(cluster=w708, "x"=w710, "y"=w709) -> (w711:cluster{"x":dbl, "y":dbl, "z":dbl})
                        n131 = local write "Position"(w711) -> ()
                      }
                    }
                  }
                }
                "Position Indicator" <- w627
              }
              event "Size": Value Change {
                # "If we were constraining the aspect ratio, or preventing a divide by zero, the size control on the FP may be incorrect.  We refresh it in here to stop it displaying a wrong value."
                # "If the size has changed, scale the spots"
                n132 = event-data() -> ("OldVal"=w721:cluster{"x":dbl, "y":dbl, "z":dbl}, "NewVal"=w727:cluster{"x":dbl, "y":dbl, "z":dbl})  [unwired: 5 out]
                n133 = Not Equal?(x=w721, y=w727) -> (x != y?=w720:cluster{"x":bool, "y":bool, "z":bool})
                n134 = Divide(x=w727, y=w721) -> (x/y=w726:cluster{"x":dbl, "y":dbl, "z":dbl})
                n135 = Not Equal To 0?(x=w721) -> (x != 0?=w719:cluster{"x":bool, "y":bool, "z":bool})
                n136 = And(x=w720, y=w719) -> (x .and. y?=w718:cluster{"x":bool, "y":bool, "z":bool})
                n137 = Cluster To Array(cluster=w718) -> (array=w725:bool[])
                n138 = Cluster To Array(cluster=w726) -> (array=w724:dbl[])
                n139 = case shown="True" "lock aspect ratio" {
                  tunnel: w725 -> [w733 w750]
                  tunnel: w724 -> [w732 w748]
                  tunnel: [w730 w740] -> w723
                  frame False {
                    # "We are not constraining the aspect ratio here, so just check we're not introducing NAs"
                    n140 = for {
                      tunnel: w733 -> [w739] mode=indexing
                      tunnel: w732 -> [w735] mode=indexing
                      tunnel: [w737] -> w731 mode=indexing
                      n141 = Not A Number/Path/Refnum?(number/path/refnum=w735) -> (NaN/Path/Refnum?=w736:bool)
                      n142 = Compound Arithmetic op=AND(w739, invert w736) -> (w738:bool)
                      n143 = Select(t=w735, s=w738, f=1.0) -> (s? t:f=w737:dbl)
                    }
                    n144 = Array To Cluster(array=w731) -> (cluster=w730:cluster{"[0]":dbl, "[1]":dbl, "[2]":dbl})
                  }
                  frame True {
                    # "Pick the first element that changed and use it.  Also need to make sure (1) an element did change and (2) everything's valid (no divide by zeros)"
                    n145 = Search 1D Array(1D array=w750, element=TRUE) -> (index of element=w747:i32)  [unwired: 1 in]
                    n146 = Index Array(array=w748, index=w747) -> (element=w743:dbl)
                    n147 = Not A Number/Path/Refnum?(number/path/refnum=w743) -> (NaN/Path/Refnum?=w746:bool)
                    n148 = Less Than 0?(x=w747) -> (x < 0?=w745:bool)
                    n149 = Or(x=w746, y=w745) -> (x .or. y?=w744:bool)
                    n150 = Select(t=1.0, s=w744, f=w743) -> (s? t:f=w741:dbl)
                    n151 = Bundle("x"=w741, "x"=w741, "x"=w741) -> (w740:cluster{"x":dbl, "x":dbl, "x":dbl})  [unwired: 1 in]
                  }
                }
                n152 = for {
                  tunnel: w729 -> [w756] mode=indexing
                  tunnel: w716 -> [w753] mode=indexing
                  tunnel: [w755] -> w717 mode=indexing
                  tunnel: w723 -> [w754]
                  tunnel: w728 -> [w751]
                  n153 = Unbundle(w753) -> ("Selected"=w752:bool)  [unwired: 1 out]
                  n154 = case shown="True" w752 {
                    tunnel: w756 -> [w757 w765]
                    tunnel: [w757 w764] -> w755
                    tunnel: w754 -> [_ w763]
                    tunnel: w751 -> [_ w759]
                    frame False {
                    }
                    frame True {
                      n155 = call "extract_position.vi"("Spot"=w765) -> ("Position"=w761:cluster{"x":dbl, "y":dbl, "z":dbl})
                      n156 = Subtract(x=w761, y=w759) -> (x-y=w762:cluster{"x":dbl, "y":dbl, "z":dbl})
                      n157 = Multiply(x=w762, y=w763) -> (x*y=w760:cluster{"x":dbl, dbl, dbl})
                      n158 = Add(x=w759, y=w760) -> (x+y=w758:cluster{"x":dbl, dbl, dbl})
                      n159 = call "replace_position.vi"("Position"=w758, "Spot in"=w765) -> ("Spot"=w764:T1)  [unwired: 2 out]
                    }
                  }
                }
                n160 = call "find_centroid.vi"("Selection and Groups"=w716, "Spots"=w717) -> ("size"=w715:cluster{"x":dbl, "y":dbl, "z":dbl})  [unwired: 2 in, 4 out]
                n161 = local write "Size"(w715) -> ()
              }
              event "Intensity": Value Change {
                # "When  the user changes intensity, scale all the spots selected so the new mean is correct but keep the ratio between the selected spots.\n\nThe exception to this is when the mean intensity is zero, in which case multiplying makes no sense- in that case we just replace with the new value."
                n162 = event-data() -> ("NewVal"=w766:dbl, "OldVal"=w773:dbl)  [unwired: 5 out]
                n163 = Equal To 0?(x=w773) -> (x = 0?=w769:bool)
                n164 = Not A Number/Path/Refnum?(number/path/refnum=w773) -> (NaN/Path/Refnum?=w768:bool)
                n165 = Or(x=w769, y=w768) -> (x .or. y?=w767:bool)
                n166 = Divide(x=w766, y=w773) -> (x/y=w770:dbl)
                n167 = for {
                  tunnel: w774 -> [w779] mode=indexing
                  tunnel: w771 -> [w781] mode=indexing
                  tunnel: [w778] -> w772 mode=indexing
                  tunnel: w770 -> [w777]
                  tunnel: w767 -> [w776]
                  tunnel: w766 -> [w775]
                  n168 = Unbundle(w781) -> ("Selected"=w780:bool)  [unwired: 1 out]
                  n169 = case shown="True" w780 {
                    tunnel: w779 -> [w782 w789]
                    tunnel: [w782 w786] -> w778
                    tunnel: w777 -> [_ w785]
                    tunnel: w776 -> [_ w784]
                    tunnel: w775 -> [_ w783]
                    frame False {
                    }
                    frame True {
                      n170 = Unbundle By Name(w789) -> ("Intensity"=w787:dbl)
                      n171 = case shown="True" w784 {
                        tunnel: [w792 w793] -> w788
                        tunnel: w787 -> [w791 _]
                        tunnel: w785 -> [w790 _]
                        tunnel: w783 -> [_ w793]
                        frame False {
                          n172 = Multiply(x=w791, y=w790) -> (x*y=w792:dbl)
                        }
                        frame True {
                        }
                      }
                      n173 = Bundle By Name(cluster=w789, "Intensity"=w788) -> (w786:T1)
                    }
                  }
                }
              }
              event "phase": Value Change {
                # "When  the user changes phase, translate the phase of all spots selectedd"
                n174 = event-data() -> ("NewVal"=w795:dbl, "OldVal"=w799:dbl)  [unwired: 5 out]
                n175 = Not A Number/Path/Refnum?(number/path/refnum=w799) -> (NaN/Path/Refnum?=w794:bool)
                n176 = Subtract(x=w795, y=w799) -> (x-y=w796:dbl)
                n177 = for {
                  tunnel: w800 -> [w805] mode=indexing
                  tunnel: w797 -> [w807] mode=indexing
                  tunnel: [w804] -> w798 mode=indexing
                  tunnel: w796 -> [w803]
                  tunnel: w794 -> [w802]
                  tunnel: w795 -> [w801]
                  n178 = Unbundle(w807) -> ("Selected"=w806:bool)  [unwired: 1 out]
                  n179 = case shown="False" w806 {
                    tunnel: w805 -> [w808 w815]
                    tunnel: [w808 w812] -> w804
                    tunnel: w803 -> [_ w811]
                    tunnel: w802 -> [_ w810]
                    tunnel: w801 -> [_ w809]
                    frame False {
                    }
                    frame True {
                      n180 = Unbundle By Name(w815) -> ("Phase"=w813:dbl)
                      n181 = case shown="False" w810 {
                        tunnel: [w818 w819] -> w814
                        tunnel: w813 -> [w817 _]
                        tunnel: w811 -> [w816 _]
                        tunnel: w809 -> [_ w819]
                        frame False {
                          n182 = Add(x=w817, y=w816) -> (x+y=w818:dbl)
                        }
                        frame True {
                        }
                      }
                      n183 = Bundle By Name(cluster=w815, "Phase"=w814) -> (w812:T1)
                    }
                  }
                }
              }
              event "Vortex Charge": Value Change {
                # "When  the user changes l, just set all selected spots to have that value of l."
                n184 = event-data() -> ("NewVal"=w820:i8)  [unwired: 6 out]
                n185 = for {
                  tunnel: w823 -> [w826] mode=indexing
                  tunnel: w821 -> [w828] mode=indexing
                  tunnel: [w825] -> w822 mode=indexing
                  tunnel: w820 -> [w824]
                  n186 = Unbundle(w828) -> ("Selected"=w827:bool)  [unwired: 1 out]
                  n187 = case shown="True" w827 {
                    tunnel: w826 -> [w829 w832]
                    tunnel: [w829 w831] -> w825
                    tunnel: w824 -> [_ w830]
                    frame False {
                    }
                    frame True {
                      n188 = Bundle By Name(cluster=w832, "Vortex Charge"=w830) -> (w831:T1)
                    }
                  }
                }
              }
            }
          }
          frame "Spot Shape" {
            # "We update the spot shape tab only when spots have changed OUTSIDE this tab.  This avoids unnecessary jumping about of the tab control."
            n189 = call "find_centroid.vi"("Selection and Groups"=w843, "Spots"=w844) -> ("Mean Values"=w839:T1)  [unwired: 2 in, 4 out]
            n190 = Wait (ms)(milliseconds to wait=u32 10) -> ()  [unwired: 1 out]
            n191 = call "spots_shape.vi"("Selection and Groups"=w843, "Spots"=w844) -> ("Spot Shape"=w846:enum32{"Normal", "Line", "NA", "Mixed"})  [unwired: 7 in]
            n192 = feedback-in #4(w839) -> ()
            n193 = feedback #4() -> (w840:T1)  [unwired: 1 in]
            n194 = Not Equal?(x=w840, y=w839) -> (x != y?=w845:bool)
            n195 = feedback #5() -> (w835:enum32{"Normal", "Line", "NA", "Mixed"})  [unwired: 1 in]
            n196 = feedback #6() -> (w837:T1)  [unwired: 1 in]
            n197 = Not Equal?(x=w837, y=w839) -> (x != y?=w836:bool)
            n198 = case shown="False" w836 {
              tunnel: w846 -> [_ w965]
              tunnel: ["Spot Shape" w965] -> w834
              frame False {
              }
              frame True {
                n199 = local write "Spot Shape"(w965) -> ()
              }
            }
            n200 = feedback-in #5(w834) -> ()
            n201 = Not Equal?(x=w834, y=w835) -> (x != y?=w833:bool)
            n202 = case shown="\"Normal\", Default" w834 {
              tunnel: w844 -> [w850 w867 w893 w963]
              tunnel: w843 -> [w849 w866 w892 w962]
              tunnel: [w849 w865 w890 w962] -> w841
              tunnel: [w848 w864 w891 w963] -> w842
              tunnel: w839 -> [_ w863 w889 _]
              tunnel: w845 -> [_ w862 w888 _]
              tunnel: w833 -> [_ w860 w886 _]
              frame "Normal", Default {
                # "If \"normal\" is selected, don't allow any NA or line-trapping stuff"
                n203 = for {
                  tunnel: w850 -> [w853] mode=indexing
                  tunnel: w849 -> [w852] mode=indexing
                  tunnel: [w854] -> w848 mode=indexing
                  n204 = Unbundle(w852) -> ("Selected"=w851:bool)  [unwired: 1 out]
                  n205 = case shown="True" w851 {
                    tunnel: [w855 w859] -> w854
                    tunnel: w853 -> [w855 w858]
                    frame False {
                    }
                    frame True {
                      n206 = Bundle By Name(cluster=w858, "NA Position"=cluster{"x":dbl, "y":dbl, "r":dbl} {"x"=0.0, "y"=0.0, "r"=1.0} ("x"), "Line Trapping"=T2 {"Vector"={"x"=0.0, "y"=0.0, "z"=0.0}, "Phase Gradient"=0.0}) -> (w859:T1)
                    }
                  }
                }
              }
              frame "Line" {
                # "If it's out of date, update front panel"
                n207 = Or(x=w862, y=w860) -> (x .or. y?=w861:bool)
                n208 = case shown="True" w861 {
                  tunnel: w863 -> [_ w870]
                  frame False {
                  }
                  frame True {
                    n209 = Unbundle By Name(w870) -> ("Line Trapping"=w869:T2)
                    n210 = local write "Line Trapping"(w869) -> ()
                  }
                }
                n211 = event shown="[1] \"Line Trapping\": Value Change" {
                  selector: _ -> [_ _]
                  dyn-events: _ -> [_ _]
                  timeout: 10 -> [_ _]
                  tunnel: w867 -> [w872 w876]
                  tunnel: w866 -> [w871 w874]
                  tunnel: [w872 w875] -> w864
                  tunnel: [w871 w874] -> w865
                  event Timeout {
                    n212 = event-data() -> ()  [unwired: 3 out]
                  }
                  event Value Change {
                    # "If the line vector has changed, update it"
                    n213 = event-data() -> ("NewVal"=w873:T2)  [unwired: 6 out]
                    n214 = for {
                      tunnel: w876 -> [w881] mode=indexing
                      tunnel: w874 -> [w878] mode=indexing
                      tunnel: [w880] -> w875 mode=indexing
                      tunnel: w873 -> [w879]
                      n215 = Unbundle(w878) -> ("Selected"=w877:bool)  [unwired: 1 out]
                      n216 = case shown="True" w877 {
                        tunnel: w881 -> [w882 w884]
                        tunnel: [w882 w885] -> w880
                        tunnel: w879 -> [_ w883]
                        frame False {
                        }
                        frame True {
                          n217 = Bundle By Name(cluster=w884, "Line Trapping"=w883) -> (w885:T1)
                        }
                      }
                    }
                  }
                }
              }
              frame "NA" {
                n218 = Or(x=w886, y=w888) -> (x .or. y?=w887:bool)
                n219 = case shown="True" w887 {
                  tunnel: w889 -> [_ w898]
                  frame False {
                  }
                  frame True {
                    n220 = Unbundle By Name(w898) -> ("NA Position"=w897:cluster{"x":dbl, "y":dbl, "r":dbl})
                    n221 = call "xyz_to_xy.vi"("Position"=w897) -> ("Position (2D)"=w896:cluster{"x":dbl, "y":dbl}, "z"=w895:dbl)  [unwired: 6 out]
                    n222 = local write "Position on back aperture"(w896) -> ()
                    n223 = local write "Radius on back aperture"(w895) -> ()
                  }
                }
                n224 = event shown="[3] \"Scale BA\": Value Change" {
                  selector: _ -> [_ _ _ _]
                  dyn-events: _ -> [_ _ _ _]
                  timeout: 10 -> [_ _ _ _]
                  tunnel: w893 -> [w900 w906 w927 w949]
                  tunnel: w892 -> [w899 w904 w924 w950]
                  tunnel: [w900 w905 w925 w947] -> w891
                  tunnel: [w899 w904 w924 w950] -> w890
                  event Timeout {
                    n225 = event-data() -> ()  [unwired: 3 out]
                  }
                  event "Position on back aperture": Value Change {
                    # "If the position has changed, translate the spots"
                    n226 = event-data() -> ("OldVal"=w902:cluster{"x":dbl, "y":dbl}, "NewVal"=w903:cluster{"x":dbl, "y":dbl})  [unwired: 5 out]
                    n227 = Subtract(x=w903, y=w902) -> (x-y=w901:cluster{"x":dbl, "y":dbl})
                    n228 = for {
                      tunnel: w906 -> [w911] mode=indexing
                      tunnel: w904 -> [w908] mode=indexing
                      tunnel: [w910] -> w905 mode=indexing
                      tunnel: w901 -> [w909]
                      n229 = Unbundle(w908) -> ("Selected"=w907:bool)  [unwired: 1 out]
                      n230 = case shown="True" w907 {
                        tunnel: w911 -> [w912 w914]
                        tunnel: [w912 w915] -> w910
                        tunnel: w909 -> [_ w916]
                        frame False {
                        }
                        frame True {
                          n231 = Unbundle By Name(w914) -> ("NA Position"=w918:cluster{"x":dbl, "y":dbl, "r":dbl})
                          n232 = call "xy_to_xyz.vi"("Position (2D)"=w916) -> ("Position (3D)"=w917:cluster{dbl, dbl, dbl})  [unwired: 1 in, 2 out]
                          n233 = Add(x=w918, y=w917) -> (x+y=w913:cluster{dbl, dbl, dbl})
                          n234 = Bundle By Name(cluster=w914, "NA Position"=w913) -> (w915:T1)
                        }
                      }
                    }
                  }
                  event "Radius on back aperture": Value Change {
                    # "When  the user changes intensity, scale all the spots selected so the new mean is correct but keep the ratio between the selected spots.\n\nThe exception to this is when the mean intensity is zero, in which case multiplying makes no sense- in that case we just replace with the new value."
                    n235 = event-data() -> ("NewVal"=w919:dbl, "OldVal"=w926:dbl)  [unwired: 5 out]
                    n236 = Equal To 0?(x=w926) -> (x = 0?=w922:bool)
                    n237 = Not A Number/Path/Refnum?(number/path/refnum=w926) -> (NaN/Path/Refnum?=w921:bool)
                    n238 = Or(x=w922, y=w921) -> (x .or. y?=w920:bool)
                    n239 = Divide(x=w919, y=w926) -> (x/y=w923:dbl)
                    n240 = for {
                      tunnel: w927 -> [w932] mode=indexing
                      tunnel: w924 -> [w934] mode=indexing
                      tunnel: [w931] -> w925 mode=indexing
                      tunnel: w923 -> [w930]
                      tunnel: w920 -> [w929]
                      tunnel: w919 -> [w928]
                      n241 = Unbundle(w934) -> ("Selected"=w933:bool)  [unwired: 1 out]
                      n242 = case shown="True" w933 {
                        tunnel: w932 -> [w935 w942]
                        tunnel: [w935 w939] -> w931
                        tunnel: w930 -> [_ w938]
                        tunnel: w929 -> [_ w937]
                        tunnel: w928 -> [_ w936]
                        frame False {
                        }
                        frame True {
                          n243 = Unbundle By Name(w942) -> ("NA Position.r"=w940:dbl)
                          n244 = case shown="False" w937 {
                            tunnel: [w945 w946] -> w941
                            tunnel: w940 -> [w944 _]
                            tunnel: w938 -> [w943 _]
                            tunnel: w936 -> [_ w946]
                            frame False {
                              n245 = Multiply(x=w944, y=w943) -> (x*y=w945:dbl)
                            }
                            frame True {
                            }
                          }
                          n246 = Bundle By Name(cluster=w942, "NA Position.r"=w941) -> (w939:T1)
                        }
                      }
                    }
                  }
                  event "Scale BA": Value Change {
                    n247 = event-data() -> ()  [unwired: 7 out]
                    n248 = for {
                      tunnel: w950 -> [w955] mode=indexing
                      tunnel: w949 -> [w953] mode=indexing
                      tunnel: "Scale back aperture" -> [w952]
                      tunnel: [w951] -> w947 mode=indexing
                      n249 = Unbundle(w955) -> ("Selected"=w954:bool)  [unwired: 1 out]
                      n250 = case shown="True" w954 {
                        tunnel: w953 -> [w956 w957]
                        tunnel: w952 -> [_ w960]
                        tunnel: [w956 w958] -> w951
                        frame False {
                        }
                        frame True {
                          n251 = Unbundle By Name(w957) -> ("NA Position"=w961:cluster{"x":dbl, "y":dbl, "r":dbl})
                          n252 = Multiply(x=w960, y=w961) -> (x*y=w959:cluster{"x":dbl, "y":dbl, "r":dbl})
                          n253 = Bundle By Name(cluster=w957, "NA Position"=w959) -> (w958:T1)
                        }
                      }
                    }
                  }
                }
              }
              frame "Mixed" {
              }
            }
            n254 = call "find_centroid.vi"("Selection and Groups"=w841, "Spots"=w842) -> ("Mean Values"=w838:T1)  [unwired: 2 in, 4 out]
            n255 = feedback-in #6(w838) -> ()
          }
          frame "Rotate" {
            w976 = u32 0 items=["Frame", "Fill", "Highlight"] ("Drawing Mode")
            w975 = u32 0 ("Color")
            w972 = i16 100 ("radius")
            # "It's necessary to check this has changed to stop us unintentionally \"spinning\" the spots..."
            # "Draw the centroid as a spot, then a large circle+cross"
            # "It's important that this loop doesn't go too fast- it hogs the CPU.  However, each tab can have a different loop speed."
            n256 = Unbundle By Name(w969) -> ("Position (Image Pixels)"=w985:cluster{"X":dbl, "Y":dbl}, "Previous Position (Image Pixels)"=w984:cluster{"X":dbl, "Y":dbl}, "Dragging"=w986:bool)
            n257 = feedback-in #7(w969) -> ()
            n258 = feedback #7() -> (w970:T10)  [unwired: 1 in]
            n259 = call "find_centroid.vi"("Selection and Groups"=w987, "Spots"=w990) -> ("centroid"=w983:cluster{"x":dbl, "y":dbl, "z":dbl})  [unwired: 2 in, 4 out]
            n260 = Not Equal?(x=w969, y=w970) -> (x != y?=w967:bool)
            n261 = Wait (ms)(milliseconds to wait=u32 10) -> ()  [unwired: 1 out]
            n262 = And(x=w967, y=w986) -> (x .and. y?=w968:bool)
            n263 = call "coords_real_to_image_currentview.vi"("Position (real coords)"=w983) -> ("Position (pixels, relative to the top left of the image)"=w966:cluster{dbl, dbl})  [unwired: 7 in, 1 out]
            n264 = case shown="True" w968 {
              tunnel: w990 -> [w999 w1043]
              tunnel: [w1001 w1042] -> w989
              tunnel: w987 -> [w1000 w1044]
              tunnel: [w1000 w1044] -> w988
              tunnel: w983 -> [w998 w1035]
              tunnel: w985 -> [_ w1034]
              tunnel: w984 -> [_ w1033]
              tunnel: w966 -> [_ w1032]
              frame False {
                n265 = event shown="[1] Timeout" {
                  selector: _ -> [_ _]
                  dyn-events: _ -> [_ _]
                  timeout: 10 -> [_ _]
                  tunnel: [w1014 w1031] -> w1001
                  tunnel: w1000 -> [w1013 _]
                  tunnel: w999 -> [w1012 w1031]
                  tunnel: w998 -> [w1008 _]
                  event "rotate": Value Change {
                    n266 = event-data() -> ()  [unwired: 6 out]
                    n267 = case shown="3" "Rotation Axis" {
                      tunnel: [cluster{dbl, dbl, dbl} {0.0, 0.0, 1.0} ("Custom Axis") cluster{dbl, dbl, dbl} {1.0, 0.0, 0.0} ("Custom Axis") cluster{dbl, dbl, dbl} {0.0, 1.0, 0.0} ("Custom Axis") "Custom Axis"] -> w1009
                      frame 0, Default {
                        # "Z"
                      }
                      frame 1 {
                        # "X"
                      }
                      frame 2 {
                        # "Y"
                      }
                      frame 3 {
                      }
                    }
                    n268 = call "normalise_3d_vector.vi"("Vector"=w1009) -> ("Unit Vector"=w1011:cluster{dbl, dbl, dbl})  [unwired: 3 out]
                    n269 = Divide(x=6.283185307179586, y=360.0) -> (x/y=w1006:dbl)
                    n270 = Multiply(x="Angle (degrees)", y=w1006) -> (x*y=w1003:dbl)
                    n271 = call "arb_rotation_matrix.vi"("Unit Vector"=w1011, "theta"=w1003) -> ("Real Matrix"=w1015:T17)
                    n272 = for {
                      tunnel: w1013 -> [w1025] mode=indexing
                      tunnel: w1012 -> [w1020] mode=indexing
                      tunnel: [w1021] -> w1014 mode=indexing
                      tunnel: w1008 -> [w1023]
                      tunnel: w1015 -> [w1022]
                      n273 = Unbundle(w1025) -> ("Selected"=w1024:bool)  [unwired: 1 out]
                      n274 = case shown="True" w1024 {
                        tunnel: w1023 -> [_ w1030]
                        tunnel: [w1026 w1029] -> w1021
                        tunnel: w1020 -> [w1026 w1028]
                        tunnel: w1022 -> [_ w1027]
                        frame False {
                        }
                        frame True {
                          n275 = call "apply_matrix_transformation_to_spots.vi"("Transform centre (i.e. transform about this point)"=w1030, "Transformation Matrix (3x3)"=w1027, "Spot In"=w1028) -> ("Spot Out"=w1029:T1)  [unwired: 5 out]
                        }
                      }
                    }
                  }
                  event Timeout {
                    n276 = event-data() -> ()  [unwired: 4 out]
                  }
                }
              }
              frame True {
                # "if the mouse has not moved, stuff will be NaN, so let's make like a leopard and not change our spots"
                # "the magnitude of the change in our direction vector gives the rotation angle in radians"
                # "If it's within 100px of the centroid, pretend the mouse is on the surface of a sphere, and synthesize Z accordingly (z^2=100^2-x^2-y^2).  This allows rotation in 3d :)  The output should always be a unit vector."
                n277 = Build Array(w1034, w1033) -> (w1049:cluster{"X":dbl, "Y":dbl}[])
                n278 = for {
                  tunnel: w1032 -> [w1082]
                  tunnel: w1049 -> [w1078] mode=indexing
                  tunnel: [w1068] -> w1048 mode=indexing
                  n279 = Subtract(x=w1078, y=w1082) -> (x-y=w1073:cluster{dbl, dbl})
                  n280 = Divide(x=w1073, y=100.0 ("x")) -> (x/y=w1074:cluster{dbl, dbl})
                  n281 = Square(x=w1074) -> (x^2=w1081:cluster{dbl, dbl})
                  n282 = Unbundle(w1081) -> (w1079:dbl, w1080:dbl)
                  n283 = Add(x=w1079, y=w1080) -> (x+y=w1070:dbl)
                  n284 = Subtract(x=1.0, y=w1070) -> (x-y=w1076:dbl)
                  n285 = Square Root(x=w1070) -> (sqrt(x)=w1071:dbl)
                  n286 = Greater Than 0?(x=w1076) -> (x > 0?=w1077:bool)
                  n287 = case shown="False" w1077 {
                    tunnel: w1076 -> [_ w1089]
                    tunnel: [0.0 w1088] -> w1067
                    tunnel: w1074 -> [w1086 w1087]
                    tunnel: w1071 -> [w1085 _]
                    tunnel: [w1084 w1087] -> w1069
                    frame False {
                      n288 = Divide(x=w1086, y=w1085) -> (x/y=w1084:cluster{dbl, dbl})
                    }
                    frame True {
                      n289 = Square Root(x=w1089) -> (sqrt(x)=w1088:dbl)
                    }
                  }
                  n290 = call "xy_to_xyz.vi"("z"=w1067, "Position (2D)"=w1069) -> ("Position (3D)"=w1068:cluster{dbl, dbl, dbl})  [unwired: 2 out]
                }
                n291 = Index Array(array=w1048) -> (element #1=w1047:cluster{dbl, dbl, dbl}, element #2=w1038:cluster{dbl, dbl, dbl})  [unwired: 2 in]
                n292 = Add(x=w1047, y=w1038) -> (x+y=w1037:cluster{dbl, dbl, dbl})
                n293 = Subtract(x=w1047, y=w1038) -> (x-y=w1036:cluster{dbl, dbl, dbl})
                n294 = call "cross_product.vi"("b"=w1037, "a"=w1036) -> ("a cross b"=w1046:cluster{dbl, dbl, dbl})
                n295 = call "normalise_3d_vector.vi"("Vector"=w1046) -> ("Unit Vector"=w1045:cluster{dbl, dbl, dbl})  [unwired: 3 out]
                n296 = call "normalise_3d_vector.vi"("Vector"=w1036) -> ("magnitude"=w1040:dbl)  [unwired: 3 out]
                n297 = Not Equal To 0?(x=w1040) -> (x != 0?=w1039:bool)
                n298 = call "arb_rotation_matrix.vi"("Unit Vector"=w1045, "theta"=w1040) -> ("Real Matrix"=w1041:T17)
                n299 = case shown="True" w1039 {
                  tunnel: w1044 -> [_ w1055]
                  tunnel: w1043 -> [w1050 w1054]
                  tunnel: [w1050 w1053] -> w1042
                  tunnel: w1041 -> [_ w1052]
                  tunnel: w1035 -> [_ w1051]
                  frame False {
                  }
                  frame True {
                    n300 = for {
                      tunnel: w1055 -> [w1061] mode=indexing
                      tunnel: w1054 -> [w1058] mode=indexing
                      tunnel: [w1057] -> w1053 mode=indexing
                      tunnel: w1052 -> [w1059]
                      tunnel: w1051 -> [w1056]
                      n301 = Unbundle(w1061) -> ("Selected"=w1060:bool)  [unwired: 1 out]
                      n302 = case shown="True" w1060 {
                        tunnel: [w1062 w1065] -> w1057
                        tunnel: w1058 -> [w1062 w1066]
                        tunnel: w1059 -> [_ w1063]
                        tunnel: w1056 -> [_ w1064]
                        frame False {
                        }
                        frame True {
                          n303 = call "apply_matrix_transformation_to_spots.vi"("Transform centre (i.e. transform about this point)"=w1064, "Transformation Matrix (3x3)"=w1063, "Spot In"=w1066) -> ("Spot Out"=w1065:T1)  [unwired: 5 out]
                        }
                      }
                    }
                  }
                }
              }
            }
            n304 = call "coords_real_to_image_currentview.vi"("Position (real coords)"=w983) -> ("Position (pixels, relative to the top left of the image)"=w978:cluster{dbl, dbl}, "z (real coords)"=w982:dbl)  [unwired: 7 in]
            n305 = expression code="z*1e7+20"(w982) -> (w994:dbl)
            n306 = In Range and Coerce(upper limit=100.0, x=w994, lower limit=2.0) -> (coerced(x)=w981:dbl)  [unwired: 1 out]
            n307 = Bundle("upper limit"=w981, "upper limit"=w981) -> (w974:cluster{"upper limit":dbl, "upper limit":dbl})  [unwired: 1 in]
            n308 = call "myoverlay_oval.vi"("Color"=w975, "Drawing Mode"=w976, "Size"=w974, "Centre Position (pixels on image)"=w978) -> ("Overlay Elements Out"=w980:T18[])  [unwired: 5 in]
            n309 = Bundle("radius"=w972, "radius"=w972) -> (w973:cluster{"radius":i16, "radius":i16})  [unwired: 1 in]
            n310 = call "myoverlay_oval.vi"("Color"=w975, "Drawing Mode"=w976, "Size"=w973, "Centre Position (pixels on image)"=w978, "Overlay Elements In"=w980) -> ("Overlay Elements Out"=w979:T18[])  [unwired: 4 in]
            n311 = Multiply(x=w972, y=cluster{dbl, dbl}[] [{0.0, 0.0}, {1.0, 0.0}, {0.0, 0.0}, {0.0, 1.0}, {0.0, 0.0}, {-1.0, 0.0}, {0.0, 0.0}, {0.0, -1.0}, {0.0, 0.0}]) -> (x*y=w991:cluster{dbl, dbl}[])
            n312 = Add(x=w978, y=w991) -> (x+y=w977:cluster{dbl, dbl}[])
            n313 = call "myoverlay_lines.vi"("Color"=w975, "Drawing Mode"=w976, "Line Endpoints"=w977, "Overlay Elements In"=w979) -> ("Overlay Elements Out"=w971:T18[])  [unwired: 5 in]
          }
          frame "Patterns" {
            n314 = event shown="[3] \"Optimise\": Value Change" {
              selector: _ -> [_ _ _ _ _]
              dyn-events: _ -> [_ _ _ _ _]
              timeout: u32 10 ("milliseconds to wait") -> [_ _ _ _ _]
              tunnel: [w1108 w1138 w1142 w1145 w1156] -> w1091
              tunnel: [w1107 w1139 w1141 w1148 w1157] -> w1090
              tunnel: w1093 -> [w1106 w1138 w1142 w1146 w1155]
              tunnel: w1092 -> [w1105 w1139 w1141 w1148 w1157]
              event "Generate": Value Change {
                # "If there were previous spots, centre the pattern on the spots"
                n315 = event-data() -> ()  [unwired: 1 in, 1 out]
                n316 = call "find_centroid.vi"("Selection and Groups"=w1105, "Spots"=w1106) -> ("size"=w1101:cluster{"x":dbl, "y":dbl, "z":dbl}, "centroid"=w1097:cluster{"x":dbl, "y":dbl, "z":dbl}, "# selected"=w1103:i16)  [unwired: 2 in, 2 out]
                n317 = Greater?(x=w1103, y=i16 1) -> (0:w1098:bool)
                n318 = case shown="False" w1098 {
                  tunnel: w1101 -> [_ w1124]
                  tunnel: [cluster{"x":dbl, "y":dbl, "z":dbl} {"x"=2e-05, "y"=2e-05, "z"=2e-05} ("size") w1124] -> w1100
                  frame False {
                  }
                  frame True {
                  }
                }
                n319 = case shown="\"HCP Shack-Hartmann\"" "Pattern" {
                  tunnel: [w1126 w1129 w1135] -> w1099
                  tunnel: w1100 -> [_ w1128 _]
                  frame "Square Shack-Hartmann" {
                    n320 = call "patterns_square_shack_hartmann.vi"("N"="Spots across centre") -> ("Spots"=w1126:T1[])
                  }
                  frame "HCP Shack-Hartmann" {
                    n321 = Unbundle By Name(w1128) -> ("x"=w1127:dbl)
                    n322 = call "pattern_hcp_shack_hartmann.vi"("Width"=w1127, "Reference Array?"="Reference Array?", "Fraction of SLM"="Fraction of SLM", "N"="Spots across centre") -> ("Shack-Hartmann Spots"=w1129:T1[])  [unwired: 7 in]
                  }
                  frame "Rectangular Grid" {
                    n323 = call "patterns_rectangular_grid.vi"("spacing/m"="spacing/m", "N"="N") -> ("Spots"=w1135:T1[])
                  }
                }
                n324 = local write "Generate"(FALSE ("Generate")) -> ()
                n325 = case shown="True" w1098 {
                  tunnel: w1099 -> [w1111 w1115]
                  tunnel: w1097 -> [_ w1117]
                  tunnel: [w1111 w1113] -> w1109
                  frame False {
                  }
                  frame True {
                    n326 = call "find_centroid.vi"("Spots"=w1115) -> ("centroid"=w1116:cluster{"x":dbl, "y":dbl, "z":dbl}, "# selected"=→"# selected":i16)  [unwired: 3 in, 3 out]
                    n327 = Subtract(x=w1117, y=w1116) -> (x-y=w1114:cluster{"x":dbl, "y":dbl, "z":dbl})
                    n328 = for {
                      tunnel: w1115 -> [w1120] mode=indexing
                      tunnel: w1114 -> [w1119]
                      tunnel: [w1118] -> w1113 mode=indexing
                      n329 = call "extract_position.vi"("Spot"=w1120) -> ("Position"=w1121:cluster{"x":dbl, "y":dbl, "z":dbl})
                      n330 = Add(x=w1121, y=w1119) -> (x+y=w1122:cluster{"x":dbl, "y":dbl, "z":dbl})
                      n331 = call "replace_position.vi"("Position"=w1122, "Spot in"=w1120) -> ("Spot"=w1118:T1)  [unwired: 2 out]
                    }
                  }
                }
                "Last Pattern" <- w1109
                n332 = call "ensure_selection_matches_spots.vi"("Select All (default: no)"=TRUE ("Select All (default: true)"), "Spots"=w1109) -> ("Selection and Groups out"=w1107:T7[], "Spots (duplicate)"=w1108:T1[])  [unwired: 4 in]
              }
              event "Spots across centre", "Fraction of SLM", "Reference Array?", "N", "spacing/m", "Spots across centre": Value Change {
                n333 = event-data() -> ()  [unwired: 1 in, 1 out]
                n334 = local read "Last Pattern"() -> (w1137:T1[])
                n335 = Equal?(x=w1138, y=w1137) -> (x = y?=w1136:bool)
                n336 = case shown="True" w1136 {
                  selector: w1136 -> [_ w1140]
                  frame False {
                  }
                  frame True {
                    n337 = property on="Generate" class="Bool (strict)"("Val(Sgnl)"=w1140) -> ()  [unwired: 2 in, 2 out]
                  }
                }
              }
              event Timeout {
                n338 = event-data() -> ()  [unwired: 1 in, 1 out]
              }
              event "Optimise": Value Change {
                n339 = event-data() -> ()  [unwired: 1 in, 1 out]
                n340 = for {
                  N: "Iterations" -> [_]
                  tunnel: 203 ("Optimisation Resolution") -> [w1152]
                  shift-right: [w1153] -> w1145
                  shift-left: w1146 -> [w1154]
                  tunnel: "Fall-off/m" -> [w1149]
                  n341 = call "do_gsw_step.vi"("Optimisation Resolution"=w1152, "Sinc Zero"=w1149, "Spots In"=w1154) -> ("non-uniformity"=→"non-uniformity":dbl, "efficiency"=→"efficiency":dbl, "Spots Out"=w1153:T1[])  [unwired: 6 in]
                }
              }
              event "Reset Phase/Amplitude": Value Change {
                n342 = event-data() -> ()  [unwired: 1 in, 1 out]
                n343 = for {
                  tunnel: [w1160] -> w1156 mode=indexing
                  tunnel: w1155 -> [w1161] mode=indexing
                  n344 = Bundle By Name(cluster=w1161, "Phase"=0.0, "Amplitude Correction"=0.0) -> (w1160:T1)
                }
              }
            }
          }
          frame "Plugins" {
            # "The local variable ensures the references are  correct when they make it through to the \"close plugins\" block."
            # "This is the error from loading/unloading VIs on the front panel"
            n345 = control-ref of="Plugin Pnl"() -> (w1165:refnum<vi>)
            n346 = Wait (ms)(milliseconds to wait=u32 10) -> ()  [unwired: 1 out]
            n347 = feedback #8() -> (w1164:T3)
            n348 = feedback #9() -> (w1166:errorcluster)
            n349 = event shown="[1] \"Plugin:\": Value Change" {
              selector: _ -> [_ _ _]
              dyn-events: _ -> [_ _ _]
              timeout: 10 -> [_ _ _]
              tunnel: "Abort Plugin" -> [w1173 _ _]
              tunnel: "Plugin:" -> [w1178 _ w1194]
              tunnel: w1166 -> [w1177 w1192 w1196]
              tunnel: [w1176 w1187 w1195] -> w1167
              tunnel: [w1175 w1188 w1198] -> w1163
              tunnel: w1164 -> [w1179 w1189 w1197]
              tunnel: w1165 -> [_ w1190 _]
              event Timeout {
                n350 = event-data() -> ()  [unwired: 1 in, 2 out]
                n351 = Not(x=w1173) -> (.not. x?=w1174:bool)
                n352 = case shown="True" w1174 {
                  tunnel: w1179 -> [w1181 w1186]
                  tunnel: w1178 -> [_ w1185]
                  tunnel: w1177 -> [w1180 w1184]
                  tunnel: [w1180 w1183] -> w1176
                  tunnel: [w1181 w1182] -> w1175
                  frame False {
                  }
                  frame True {
                    n353 = call "plugins_run.vi"("Error In"=w1184, "Plugin Index"=w1185, "Plugins In"=w1186) -> ("Error Out"=w1183:errorcluster, "Plugins"=w1182:T3)  [unwired: 7 in]
                  }
                }
              }
              event "Plugin:": Value Change {
                n354 = event-data() -> ("NewVal"=w1191:u16)  [unwired: 1 in]
                n355 = call "plugins_switch.vi"("error in"=w1192, "Plugin Pnl"=w1190, "Plugin Index"=w1191, "Plugins In"=w1189) -> ("error out"=w1187:errorcluster, "Plugins Out"=w1188:T3)  [unwired: 4 in]
              }
              event "Abort Plugin": Value Change {
                n356 = event-data() -> ("NewVal"=w1193:bool)  [unwired: 1 in]
                n357 = case shown="True" w1193 {
                  tunnel: [w1200 w1205] -> w1198
                  tunnel: w1197 -> [w1200 w1204]
                  tunnel: w1196 -> [w1199 w1203]
                  tunnel: [w1199 w1202] -> w1195
                  tunnel: w1194 -> [_ w1201]
                  frame False {
                  }
                  frame True {
                    n358 = call "plugins_abort.vi"("Error In"=w1203, "Plugin Index"=w1201, "Plugins In"=w1204) -> ("Error Out"=w1202:errorcluster, "Plugins Out"=w1205:T3)  [unwired: 7 in]
                  }
                }
              }
            }
            n359 = feedback-in #8(w1163) -> ()
            n360 = feedback-in #9(w1167) -> ()
            n361 = local write "Plugins"(w1163) -> ()
          }
          frame "Video" {
            # "All the controls on this tab are in the bottom (camera) loop."
            n362 = Wait (ms)(milliseconds to wait=u32 10) -> ()  [unwired: 1 out]
            n363 = property on="Property Node" class="ImageControl"(reference=w1206) -> ("Image Information String"=→"Image Information":string)  [unwired: 1 in, 2 out]
          }
        }
        n364 = case shown="True" "Clear String" {
          frame False {
          }
          frame True {
            w559 = ""
            n365 = local write "Sequence Frames To Check"(w559) -> ()
            n366 = local write "String 2"(w559) -> ()
          }
        }
      }
      event "Tab": Value Change {
        w1214 = T19 [enum."Video", enum."Particle Tracking"] items=["Current Spot", "Rotate", "Spot Shape", "Patterns", "Plugins", "Video", "Particle Tracking", "Clamping", "Blank"]
        w1219 = refnum<vi> refnum  # Image
        # "This allows us to disable custom mouse-handling for certain tabs.  It can also be done from within the \"mouse down\" event case."
        n367 = event-data() -> ("NewVal"=w1215:T4)  [unwired: 1 in, 3 out]
        n368 = Equal?(x=w1214, y=w1215) -> (x = y?=w1213:bool[])
        n369 = Or Array Elements(Boolean array=w1213) -> (logical OR=w1212:bool)
        n370 = Not(x=w1212) -> (.not. x?=w1211:bool)
        n371 = Select(t=w1218, s=w1211, f=w1219) -> (s? t:f=w1220:refnum<vi>)
        n372 = register-events(reference=w1222, w1220, w1219, w1219, w1219) -> (reference out=w1221:refnum<event-registration>)  [unwired: 1 in, 1 out]
      }
      event Menu Selection (User) {
        n373 = event-data() -> ("ItemTag"=w1230:string, "MenuRef"=w1223:refnum<k9>)  [unwired: 1 in]
        n374 = case shown="\"ToggleSavingData\"" w1230 {
          tunnel: w1234 -> [w1238 w1248 w1257 w1271 w1290 w1294 w1297 w1304 w1311 w1313 w1316 w1345 w1371 w1392 w1403 w1414 w1417 w1419 w1424 w1427]
          tunnel: w1233 -> [w1237 w1247 w1256 w1280 w1289 w1293 w1295 w1302 w1310 w1312 w1315 w1344 w1370 w1391 w1402 w1413 w1416 w1420 w1425 w1426]
          tunnel: [w1238 w1248 w1257 w1271 w1288 w1291 w1297 w1304 w1311 w1313 w1316 w1345 w1371 w1392 w1403 w1414 w1417 w1419 w1424 w1427] -> w1232
          tunnel: [w1237 w1247 w1256 w1280 w1287 w1292 w1296 w1303 w1309 w1314 w1317 w1344 w1370 w1391 w1402 w1413 w1416 w1420 w1425 w1426] -> w1231
          tunnel: [_ _ _ _ TRUE _ _ _ _ _ _ _ _ _ _ _ _ _ _ _] -> w1225
          tunnel: w1224 -> [_ _ _ _ _ _ _ _ _ _ _ w1343 w1369 w1383 _ _ _ _ _ _]
          tunnel: w1223 -> [_ _ _ _ _ _ _ _ _ _ _ w1334 w1363 w1386 w1397 w1408 _ _ _ _]
          frame "ToggleSavingData" {
            # "Data is saved from the middle loop: look there for an explanation."
            n375 = local read "Save Video"() -> (w1236:bool)
            n376 = Not(x=w1236) -> (.not. x?=w1235:bool)
            n377 = local write "Save Video"(w1235) -> ()
          }
          frame "SaveStateToFile" {
            # "Save the current settings (i.e. the values of all the controls in VIs that have [Red Tweezers Save Settings] in their documentation string) to a file."
            n378 = call "File Dialog"("prompt"="Please select a location to save the settings", "button label"="Save", "default name"="red_tweezers_settings.xml", "pattern (all files)"="*.xml" ("pattern label"), "pattern label"="XML Settings Files") -> ("selected path"=w1246:path, "cancelled"=w1239:bool)  [unwired: 7 in, 2 out]
            n379 = Not(x=w1239) -> (.not. x?=w1240:bool)
            n380 = case shown="True" w1240 {
              tunnel: w1246 -> [_ w1250]
              frame False {
              }
              frame True {
                n381 = Path To String(path=w1250) -> (string=w1249:string)
                n382 = call "settings_save_to_file.vi"("XML File Path"=w1250) -> ()  [unwired: 11 in]
                n383 = call "settings_filename_to_registry.vi"("Last Used Settings File"=w1249) -> ()  [unwired: 11 in]
              }
            }
          }
          frame "SaveStateToCurrentFile" {
            # "As SaveStateToFile, but using the current file (i.e. Save not Save As...)."
            n384 = global read "red_tweezers_globals_INTERNAL_VOLATILE.vi" "Current Settings File"() -> (w1255:path)
            n385 = call <vilib>:"Check if File or Folder Exists.vi"("path"=w1255) -> ("file or folder exists?"=w1254:bool, "dup path"=w1253:path)  [unwired: 8 in, 1 out]
            n386 = case shown="True" w1254 {
              selector: w1254 -> [_ w1268]
              tunnel: w1253 -> [_ w1269]
              tunnel: [w1260 w1269] -> w1252
              tunnel: [w1261 w1268] -> w1251
              frame False {
                n387 = call "File Dialog3"("prompt"="Please select a location to save the settings", "button label"="Save", "default name"="red_tweezers_settings.xml", "pattern (all files)"="*.xml" ("pattern label"), "pattern label"="XML Settings Files") -> ("selected path"=w1260:path, "cancelled"=w1267:bool)  [unwired: 7 in, 2 out]
                n388 = Not(x=w1267) -> (.not. x?=w1261:bool)
              }
              frame True {
              }
            }
            n389 = case shown="True" w1251 {
              tunnel: w1252 -> [_ w1259]
              frame False {
              }
              frame True {
                n390 = Path To String(path=w1259) -> (string=w1258:string)
                n391 = call "settings_save_to_file.vi"("XML File Path"=w1259) -> ()  [unwired: 11 in]
                n392 = call "settings_filename_to_registry.vi"("Last Used Settings File"=w1258) -> ()  [unwired: 11 in]
              }
            }
          }
          frame "LoadStateFromFile" {
            # "Load a file, and use it to reset the values of all the front panel controls."
            # "We need to re-run the initialisation stuff in UDP sender after changing settings\n(for example, this synchronises the settings like camera pixel size with the\nrelevant global variable)"
            n393 = call "File Dialog2"("prompt"="Please select a settings file", "button label"="Open", "default name"="red_tweezers_settings.xml", "pattern (all files)"="*.xml" ("pattern label"), "pattern label"="XML Settings Files") -> ("selected path"=w1272:path, "cancelled"=w1279:bool)  [unwired: 7 in, 2 out]
            n394 = Not(x=w1279) -> (.not. x?=w1278:bool)
            n395 = case shown="False" w1278 {
              selector: w1278 -> [w1281 w1282]
              tunnel: w1272 -> [_ w1283]
              tunnel: [w1281 w1282] -> w1270
              frame False {
              }
              frame True {
                n396 = call "settings_load_from_file.vi"("XML File Path"=w1283) -> ()  [unwired: 9 in, 2 out]
                n397 = Path To String(path=w1283) -> (string=w1284:string)
                n398 = call "settings_filename_to_registry.vi"("Last Used Settings File"=w1284) -> ()  [unwired: 11 in]
              }
            }
            n399 = call "UDP Sender generic_2.vi"("re-initialise"=w1270, "Spots"=w1271) -> ()  [unwired: 1 in, 1 out]
          }
          frame "Undo" {
            # "This should get the last undo vector and replace the spots with it :)"
            n400 = call "red_tweezers_UNDO.vi"("Selection/Group"=w1289, "Undo/Store (store, False)"=TRUE, "Spots"=w1290) -> ("Selection/Group Out (Undo only)"=w1287:T7[], "Spots Out (Undo only)"=w1288:T1[])  [unwired: 7 in]
          }
          frame "Delete" {
            n401 = call "delete_selected_spots.vi"("Selection/Group 3"=w1293, "Spots 3"=w1294) -> ("Selection/Group 2"=w1292:T7[], "Spots 2"=w1291:T1[])  [unwired: 4 in]
          }
          frame "SelectAllSpots" {
            n402 = for {
              tunnel: w1295 -> [w1300] mode=indexing
              tunnel: [w1301] -> w1296 mode=indexing
              n403 = Unbundle(w1300) -> ("Group ID"=w1299:i32)  [unwired: 1 out]
              n404 = Bundle(cluster=w1300, "Group ID"=w1299, "Selected"=TRUE ("Label.Visible")) -> (w1301:T7)
            }
          }
          frame "SelectNoSpots" {
            n405 = for {
              tunnel: w1302 -> [w1307] mode=indexing
              tunnel: [w1308] -> w1303 mode=indexing
              n406 = Unbundle(w1307) -> ("Group ID"=w1306:i32)  [unwired: 1 out]
              n407 = Bundle(cluster=w1307, "Group ID"=w1306, "Selected"=FALSE ("Label.Visible")) -> (w1308:T7)
            }
          }
          frame "SelectSpecificSpots" {
            n408 = call "select_by_id.vi"("Selection/Group"=w1310, "Spots"=w1311) -> ("Selection/Group Out"=w1309:T7[])  [unwired: 9 in]
          }
          frame "Group" {
            # "Group the currently selected spots"
            n409 = call "group_selected_spots.vi"("Selection/Group 2"=w1312) -> ("Array"=w1314:T7[])
          }
          frame "Ungroup" {
            # "Ungroup the currently selected spots"
            n410 = for {
              tunnel: [w1321] -> w1317 mode=indexing
              tunnel: w1315 -> [w1320] mode=indexing
              tunnel: 0 -> [w1319]
              n411 = Unbundle(w1320) -> ("Selected"=w1322:bool)  [unwired: 1 out]
              n412 = case shown="False" w1322 {
                tunnel: [w1323 w1326] -> w1321
                tunnel: w1320 -> [w1323 w1325]
                tunnel: w1319 -> [_ w1324]
                frame False {
                }
                frame True {
                  n413 = Unbundle(w1325) -> ("Selected"=w1327:bool)  [unwired: 1 out]
                  n414 = Bundle(cluster=w1325, "Group ID"=w1324, "Selected"=w1327) -> (w1326:T7)
                }
              }
            }
          }
          frame "ZoomIn" {
            w1328 = "ZoomToFit" ("item tag")
            # "turn off \"zoom to fit\""
            n415 = property class="ImageControl"(reference=w1343) -> (reference out=w1337:refnum<vi>, "ZoomSingle"=w1342:cluster{"X":sgl, "Y":sgl}, "Image Center Position"=w1335:cluster{"X":u32, "Y":u32})  [unwired: 1 in, 1 out]
            n416 = Unbundle(w1342) -> ("X"=w1340:sgl)  [unwired: 1 out]
            n417 = Round To Nearest(number=w1340) -> (nearest integer value=w1336:sgl)
            n418 = Greater Than 0?(x=w1336) -> (x > 0?=w1341:bool)
            n419 = case shown="True" w1341 {
              tunnel: w1340 -> [w1350 w1353]
              tunnel: [w1349 w1351] -> w1339
              frame False {
                n420 = Reciprocal(x=w1350) -> (1/x=w1347:sgl)
                n421 = Round Toward +Infinity(x=w1347) -> (ceil(x): smallest int >= x=w1348:sgl)
                n422 = Decrement(x=w1348) -> (x-1=w1346:sgl)
                n423 = Reciprocal(x=w1346) -> (1/x=w1349:sgl)
              }
              frame True {
                n424 = Round Toward -Infinity(1:w1353) -> (0:w1352:sgl)
                n425 = Increment(x=w1352) -> (x+1=w1351:sgl)
              }
            }
            n426 = Bundle(w1339, w1339) -> (w1338:cluster{sgl, sgl})  [unwired: 1 in]
            n427 = property class="ImageControl"(reference=w1337, "ZoomSingle"=w1338, "Image Center Position"=w1335) -> ()  [unwired: 1 in, 2 out]
            n428 = Get Menu Item Info(7:w1328, 11:w1334) -> (1:w1331:bool, 2:w1332:string, 3:w1333:refnum<k9>, 6:w1330:T20)  [unwired: 1 in, 3 out]
            n429 = Set Menu Item Info(4:w1330, 6:FALSE ("checked"), 7:w1328, 9:w1331, 10:w1332, 11:w1333) -> ()  [unwired: 1 in, 2 out]
          }
          frame "ZoomOut" {
            w1357 = "ZoomToFit" ("item tag")
            # "turn off \"zoom to fit\""
            n430 = property class="ImageControl"(reference=w1369) -> (reference out=w1365:refnum<vi>, "ZoomSingle"=w1368:cluster{"X":sgl, "Y":sgl}, "Image Center Position"=w1364:cluster{"X":u32, "Y":u32})  [unwired: 1 in, 1 out]
            n431 = Unbundle(w1368) -> ("X"=w1354:sgl)  [unwired: 1 out]
            n432 = Greater?(x=w1354, y=1.0) -> (0:w1356:bool)
            n433 = case shown="False" w1356 {
              tunnel: w1354 -> [w1378 w1381]
              tunnel: [w1377 w1379] -> w1367
              frame False {
                n434 = Reciprocal(x=w1378) -> (1/x=w1375:sgl)
                n435 = Add(x=w1375, y=sgl 0.01 ("x")) -> (x+y=w1373:sgl)
                n436 = Round Toward -Infinity(1:w1373) -> (0:w1376:sgl)
                n437 = Increment(x=w1376) -> (x+1=w1374:sgl)
                n438 = Reciprocal(x=w1374) -> (1/x=w1377:sgl)
              }
              frame True {
                n439 = Round Toward +Infinity(x=w1381) -> (ceil(x): smallest int >= x=w1380:sgl)
                n440 = Decrement(x=w1380) -> (x-1=w1379:sgl)
              }
            }
            n441 = Bundle(w1367, w1367) -> (w1366:cluster{sgl, sgl})  [unwired: 1 in]
            n442 = property class="ImageControl"(reference=w1365, "ZoomSingle"=w1366, "Image Center Position"=w1364) -> ()  [unwired: 1 in, 2 out]
            n443 = Get Menu Item Info(7:w1357, 11:w1363) -> (1:w1360:bool, 2:w1361:string, 3:w1362:refnum<k9>, 6:w1359:T20)  [unwired: 1 in, 3 out]
            n444 = Set Menu Item Info(4:w1359, 6:FALSE ("checked"), 7:w1357, 9:w1360, 10:w1361, 11:w1362) -> ()  [unwired: 1 in, 2 out]
          }
          frame "ZoomToFit" {
            w1387 = "ZoomToFit" ("item tag")
            # "and make sure the image obeys the result"
            # "Toggle menu checkmark"
            n445 = Get Menu Item Info(7:w1387, 11:w1386) -> (1:w1385:bool, 2:w1389:string, 3:w1390:refnum<k9>, 4:w1384:bool, 6:w1388:T20)  [unwired: 1 in, 2 out]
            n446 = Not(x=w1384) -> (.not. x?=w1382:bool)
            n447 = Set Menu Item Info(4:w1388, 6:w1382, 7:w1387, 9:w1385, 10:w1389, 11:w1390) -> ()  [unwired: 1 in, 2 out]
            n448 = property class="ImageControl"(reference=w1383, "Zoom to Fit Mode"=w1382) -> ()  [unwired: 1 in, 2 out]
          }
          frame "ShowGrid" {
            w1398 = "ShowGrid" ("item tag")
            # "Toggle menu checkmark"
            n449 = Get Menu Item Info(7:w1398, 11:w1397) -> (1:w1396:bool, 2:w1400:string, 3:w1401:refnum<k9>, 4:w1395:bool, 6:w1399:T20)  [unwired: 1 in, 2 out]
            n450 = Not(x=w1395) -> (.not. x?=w1394:bool)
            n451 = Set Menu Item Info(4:w1399, 6:w1394, 7:w1398, 9:w1396, 10:w1400, 11:w1401) -> ()  [unwired: 1 in, 2 out]
            n452 = call "grid_and_guides.vi"("Boolean"=w1394, "Operation"=T12."Set grid visibility") -> ()  [unwired: 9 in, 1 out]
          }
          frame "ShowGuides" {
            w1409 = "ShowGuides" ("item tag")
            # "Toggle menu checkmark"
            n453 = Get Menu Item Info(7:w1409, 11:w1408) -> (1:w1407:bool, 2:w1411:string, 3:w1412:refnum<k9>, 4:w1406:bool, 6:w1410:T20)  [unwired: 1 in, 2 out]
            n454 = Not(x=w1406) -> (.not. x?=w1405:bool)
            n455 = Set Menu Item Info(4:w1410, 6:w1405, 7:w1409, 9:w1407, 10:w1411, 11:w1412) -> ()  [unwired: 1 in, 2 out]
            n456 = call "grid_and_guides.vi"("Boolean"=w1405, "Operation"=T12."Set guide visibility") -> ()  [unwired: 9 in, 1 out]
          }
          frame "ConfigureGridAndGuides" {
            n457 = call "grid_and_guides.vi"("Operation"=T12."Show front panel") -> ()  [unwired: 10 in, 1 out]
          }
          frame "ShowSettings" {
            n458 = call "UDP Sender generic_2.vi"("Show panel"=TRUE, "Spots"=w1419) -> ()  [unwired: 1 in, 1 out]
          }
          frame "CameraSettings" {
            n459 = global read "red_tweezers_globals_INTERNAL_VOLATILE.vi" "Current Camera VI"() -> (w1422:path)
            n460 = Open VI Reference(vi path=w1422) -> (vi reference=w1421:refnum<vi>)  [unwired: 5 in, 1 out]
            n461 = property class="VI"(reference=w1421, "Front Panel.Open"=TRUE ("Front Panel Window:Open")) -> ()  [unwired: 1 in, 2 out]
          }
          frame Default {
          }
        }
      }
      event Mouse Down? {
        # "We don't process clicks when the user is on the video tab, so that we can set ROIs."
        # "When the mouse button goes down over the image, we save where it went down, etc. and wait to see what happens next.  We also register to be told when the mouse leaves the control, goes up, or moves.  \"click\" or \"drag\" are only detected once the mouse moves or goes up."
        n462 = event-data() -> ("Coords"=w1442:T21, "Button"=w1437:u16, "Mods"=w1446:cluster{"Double Click":bool, "Menu Key":bool}, "PlatMods"=w1445:T22)  [unwired: 1 in]
        n463 = call "mouse_to_image_coords.vi"("Mouse Coords (screen/pane units)"=w1442, "Image Control"=w1438) -> ("Cursor is on Display Area"=w1436:bool, "Mouse Coords (image pixels)"=w1441:cluster{dbl, dbl})  [unwired: 4 in]
        n464 = disable-structure shown="Enabled" {
          disable-tunnel: w1437 -> [w1454 _]
          disable-tunnel: w1436 -> [w1452 w1455]
          disable-tunnel: [w1451 w1455] -> w1432
          frame Enabled {
            n465 = Equal?(x=u16 1, y=w1454) -> (x = y?=w1453:bool)
            n466 = And(x=w1452, y=w1453) -> (x .and. y?=w1451:bool)
          }
          frame Disabled {
            # "use other pane to allow right-clicking on image"
          }
        }
        n467 = local read "Tab"() -> (w1433:T4)
        n468 = Not Equal?(x=w1433, y=T13."Video" ("Tab")) -> (x != y?=w1431:bool)
        n469 = And(x=w1432, y=w1431) -> (x .and. y?=w1430:bool)
        n470 = case shown="False" w1430 {
          tunnel: w1449 -> [w1458 w1469]
          tunnel: [T10 {"Button Down"=FALSE, "Dragging"=FALSE, "Position (Image Pixels)"={"X"=0.0, "Y"=0.0}, "Previous Position (Image Pixels)"={"X"=0.0, "Y"=0.0}, "Button"=0, "Mods"={"Double Click"=FALSE, "Menu Key"=FALSE}, "PlatMods"={"Shift"=FALSE, "Ctrl"=FALSE, "Alt"=FALSE, "Cmd"=FALSE, "Opt"=FALSE}} w1468] -> w1448
          tunnel: [w1458 w1465] -> w1447
          tunnel: w1437 -> [_ w1464]
          tunnel: w1446 -> [_ w1463]
          tunnel: w1445 -> [_ w1462]
          tunnel: w1441 -> [_ w1461]
          tunnel: [FALSE TRUE] -> w1440
          tunnel: w1438 -> [_ w1459]
          frame False {
            # "If the user clicked on a scrollbar, ignore it and let LabVIEW handle it. (this keeps the scrollbars working)"
          }
          frame True {
            w1467 = FALSE  # Dragging
            w1466 = TRUE  # Button Down
            n471 = register-events(reference=w1469, w1459, w1459, w1459, w1459) -> (reference out=w1465:refnum<event-registration>)  [unwired: 1 in, 1 out]
            n472 = Bundle("Button Down"=w1466, "Dragging"=w1467, "Mouse Coords (image pixels)"=w1461, "Mouse Coords (image pixels)"=w1461, "Button"=w1464, "Mods"=w1463, "PlatMods"=w1462) -> (w1468:T23)  [unwired: 1 in]
          }
        }
        n473 = Array Size(array=w1428) -> (size(s)=w1429:i32)
        n474 = local write "# of Spots"(w1429) -> ()
        n475 = local write "Selection/Group"(w1428) -> ()
        n476 = event-data("Discard?"=w1440) -> ()  [unwired: 4 in, 1 out]
      }
      event Mouse Leave {
        w1476 = refnum<vi> refnum  # Dummy
        # "When the mouse leaves, we reset things."
        n477 = event-data() -> ()  [unwired: 1 in, 2 out]
        n478 = register-events(reference=w1477, w1475, w1476, w1476, w1476) -> (reference out=w1474:refnum<event-registration>)  [unwired: 1 in, 1 out]
      }
      event Mouse Up {
        w1496 = refnum<vi> refnum  # Dummy
        # "Double clicking adds a spot at the mouse position."
        # "deregister"
        # "If we get here the mouse has gone down and up again.  If we've not moved in between, we have a Click.\nEither way we're no longer interested in mouse leave/move/up events."
        n479 = event-data() -> ("Mods"=w1483:cluster{"Double Click":bool, "Menu Key":bool})  [unwired: 1 in, 5 out]
        n480 = Unbundle By Name(w1489) -> ("Dragging"=w1498:bool)
        n481 = Unbundle By Name(w1483) -> ("Double Click"=w1480:bool)
        n482 = Not(x=w1498) -> (.not. x?=w1497:bool)
        n483 = Not(x=w1485) -> (.not. x?=w1487:bool)
        n484 = And(x=w1497, y=w1487) -> (x .and. y?=w1481:bool)
        n485 = case shown="True" w1481 {
          tunnel: w1489 -> [_ w1504]
          tunnel: w1491 -> [w1499 w1503]
          tunnel: w1490 -> [w1500 w1506]
          tunnel: [w1500 w1505] -> w1492
          tunnel: w1480 -> [_ w1501]
          tunnel: [w1499 w1502] -> w1482
          frame False {
          }
          frame True {
            n486 = case shown="False" w1501 {
              tunnel: w1506 -> [w1513 w1563]
              tunnel: [w1511 w1569] -> w1505
              tunnel: w1503 -> [w1507 w1570]
              tunnel: w1504 -> [w1510 w1565]
              tunnel: [w1507 w1561] -> w1502
              frame False {
                w1517 = 400.0  # 20^2 px
                # "If the user clicked, determine which spots should be selected: if we've clicked a spot/group then select it.  Shift-clicking toggles selection for that spot, and leaves the rest of the selection unchanged."
                # "check we're close enough"
                # "find closest"
                n487 = Unbundle By Name(w1510) -> ("Position (Image Pixels)"=w1509:cluster{"X":dbl, "Y":dbl}, "PlatMods.Shift"=w1508:bool)
                n488 = for {
                  tunnel: [w1553] -> w1515 mode=indexing
                  tunnel: w1509 -> [w1552]
                  tunnel: w1507 -> [w1551] mode=indexing
                  # "calculate distances between mouse position and spot positions"
                  n489 = call "extract_position.vi"("Spot"=w1551) -> ("Position"=w1550:cluster{"x":dbl, "y":dbl, "z":dbl})
                  n490 = call "coords_real_to_image_currentview.vi"("Position (real coords)"=w1550) -> ("Position (pixels, relative to the top left of the image)"=w1549:cluster{dbl, dbl})  [unwired: 7 in, 1 out]
                  n491 = Subtract(x=w1549, y=w1552) -> (x-y=w1556:cluster{dbl, dbl})
                  n492 = Multiply(x=w1556, y=w1556) -> (x*y=w1555:cluster{dbl, dbl})
                  n493 = Cluster To Array(cluster=w1555) -> (array=w1554:dbl[])
                  n494 = Add Array Elements(numeric array=w1554) -> (sum=w1553:dbl)
                }
                n495 = Array Max & Min(array=w1515) -> (min value=w1516:dbl, min index (indices)=w1512:i32)  [unwired: 2 out]
                n496 = Less Or Equal?(x=w1516, y=w1517) -> (x <= y?=w1514:bool)
                n497 = case shown="True" w1514 {
                  tunnel: w1513 -> [w1518 w1525]
                  tunnel: w1512 -> [_ w1519]
                  tunnel: w1508 -> [_ w1521]
                  tunnel: [w1518 w1520] -> w1511
                  frame False {
                    # "If we didn't click a spot, do nothing."
                  }
                  frame True {
                    # "If the spot is in a group, act on all spots in that group, not just the spot we clicked."
                    # "This case statement toggles the selection of the spot/group we clicked, and leaves other spots unchanged if we're holding shift.  Otherwise, we select the spot/group that was clicked and deselect everything else."
                    n498 = stacked-sequence {
                      tunnel: w1519 -> [_ w1527]
                      frame #0 {
                        n499 = local read "Current Spot #"() -> (→"Prev Current Spot":dbl)
                      }
                      frame #1 {
                        "Current Spot #" <- w1527
                      }
                    }
                    n500 = Index Array(array=w1525, index=w1519) -> (element=w1524:T7)
                    n501 = Unbundle(w1524) -> ("Group ID"=w1522:i32)  [unwired: 1 out]
                    n502 = Greater Than 0?(x=w1522) -> (x > 0?=w1523:bool)
                    n503 = for {
                      tunnel: w1525 -> [w1538] mode=indexing
                      tunnel: w1523 -> [w1535]
                      tunnel: w1522 -> [w1534]
                      tunnel: w1519 -> [w1533]
                      tunnel: w1521 -> [w1531]
                      tunnel: [w1529] -> w1520 mode=indexing
                      i -> [w1532]
                      n504 = Unbundle(w1538) -> ("Group ID"=w1528:i32, "Selected"=w1536:bool)
                      n505 = case shown="True" w1535 {
                        tunnel: w1528 -> [_ w1542]
                        tunnel: [w1540 w1544] -> w1530
                        tunnel: w1534 -> [_ w1543]
                        tunnel: w1533 -> [w1541 _]
                        tunnel: w1532 -> [w1539 _]
                        frame False {
                          n506 = Equal?(x=w1539, y=w1541) -> (x = y?=w1540:bool)
                        }
                        frame True {
                          n507 = Equal?(x=w1542, y=w1543) -> (x = y?=w1544:bool)
                        }
                      }
                      n508 = case shown="True" w1531 {
                        tunnel: [w1545 w1546] -> w1537
                        tunnel: w1536 -> [_ w1547]
                        tunnel: w1530 -> [w1545 w1548]
                        frame False {
                        }
                        frame True {
                          n509 = Exclusive Or(1:w1548, 2:w1547) -> (0:w1546:bool)
                        }
                      }
                      n510 = Bundle("Group ID"=w1528, w1537) -> (w1529:cluster{"Group ID":i32, bool})  [unwired: 1 out]
                    }
                  }
                }
              }
              frame True {
                # "convert mouse position to real coords, and add a spot there."
                # "Double-click detected"
                n511 = Unbundle By Name(w1565) -> ("Position (Image Pixels)"=w1564:cluster{"X":dbl, "Y":dbl})
                n512 = for {
                  tunnel: w1563 -> [w1573] mode=indexing
                  tunnel: [w1572] -> w1562 mode=indexing
                  n513 = Bundle(cluster=w1573, "Selected"=FALSE) -> (w1572:T7)  [unwired: 1 in]
                }
                n514 = call "coords_image_to_real_currentimage.vi"("Position (pixels on image)"=w1564) -> ("Position (real coords)"=w1566:cluster{dbl, dbl, "Z":dbl})  [unwired: 9 in]
                n515 = call "replace_position.vi"("Position"=w1566) -> ("Spot"=w1568:T1)  [unwired: 3 in]
                n516 = Build Array (concatenate)(w1570, w1568) -> (w1561:T1[])
                n517 = Build Array (concatenate)(w1562, T7 {"Group ID"=0, "Selected"=TRUE} ("selection_element")) -> (w1569:T7[])
                n518 = Array Size(array=w1561) -> (size(s)=w1560:i32)
                n519 = local write "Induce check"(TRUE) -> ()
                n520 = Subtract(x=w1560, y=1) -> (x-y=w1559:i32)
                n521 = local write "Current Spot #"(w1559) -> ()
              }
            }
          }
        }
        n522 = register-events(reference=w1494, w1493, w1496, w1496, w1496) -> (reference out=w1495:refnum<event-registration>)  [unwired: 1 in, 1 out]
      }
      event Mouse Move {
        n523 = event-data() -> ("Coords"=w1588:T21)  [unwired: 1 in, 2 out]
        n524 = call "mouse_to_image_coords.vi"("Mouse Coords (screen/pane units)"=w1588, "Image Control"=w1587) -> ("Mouse Coords (image pixels)"=w1579:cluster{dbl, dbl})  [unwired: 4 in, 1 out]
        n525 = Not(x=w1578) -> (.not. x?=w1583:bool)
        n526 = case shown="True" w1583 {
          tunnel: w1581 -> [_ w1601]
          tunnel: w1586 -> [w1593 w1603]
          tunnel: w1585 -> [w1592 w1602]
          tunnel: [w1592 w1602] -> w1574
          tunnel: [w1593 w1604] -> w1584
          tunnel: w1579 -> [_ w1595]
          tunnel: w1575 -> [_ w1594]
          frame False {
          }
          frame True {
            # "this is the displacement of the mouse, since the last iteration, in \"real\" coordinates (NB the conversions go before subtracting, as it may involve adding a constant as well as multiplying, which would confuse things as we're only interested in displacements here."
            # "The \"position\" local variable is there just in case we're on the \"current spot\" tab, so that the position updates nicely"
            # "If the user is dragging, translate the spots.\nHolding down shift causes the mouse's motion to be transformed into scaling about the centroid of the spots and rotation about the same point"
            n527 = Unbundle By Name(w1601) -> ("Position (Image Pixels)"=w1596:cluster{"X":dbl, "Y":dbl})
            n528 = call "find_centroid.vi"("Selection and Groups"=w1602, "Spots"=w1603) -> ("centroid"=w1597:cluster{"x":dbl, "y":dbl, "z":dbl})  [unwired: 2 in, 4 out]
            n529 = Unbundle By Name(w1601) -> ("PlatMods.Shift"=w1600:bool)
            n530 = disable-structure shown="Disabled" {
              disable-tunnel: w1597 -> [w1605 _]
              frame Disabled {
                n531 = local write "Position"(w1605) -> ()
              }
              frame Enabled {
              }
            }
            n532 = call "coords_image_to_real_currentimage.vi"("Position (pixels on image)"=w1595) -> ("Position (real coords)"=w1598:cluster{dbl, dbl, "Z":dbl})  [unwired: 9 in]
            n533 = call "coords_image_to_real_currentimage.vi"("Position (pixels on image)"=w1596) -> ("Position (real coords)"=w1599:cluster{dbl, dbl, "Z":dbl})  [unwired: 9 in]
            n534 = case shown="False" w1600 {
              tunnel: [w1610 w1884] -> w1604
              tunnel: w1603 -> [w1616 w1885]
              tunnel: w1602 -> [w1615 w1883]
              tunnel: w1599 -> [w1614 w1870]
              tunnel: w1597 -> [_ w1880]
              tunnel: w1598 -> [w1611 w1871]
              tunnel: w1594 -> [_ _]
              frame False {
                # "Spot Checker passes on information for the bubble collision,system so proper calculations can be made."
                n535 = while {
                  tunnel: w1614 -> [w1655]
                  tunnel: [w1645] -> w1612
                  tunnel: w1611 -> [w1644]
                  i -> [w1638]
                  stop <- w1640 stop-if-true
                  w1630 = 0
                  # "This while loop statement makes sure\nthat every spot gets checked before \nallowing any spot to move."
                  # "Buffer zone controls the amount of space between the\ncenter of a spot compared to the center of another spot.\nThis is used to prevent bubbles from colliding with each other."
                  # "Projected distance calculates the distance between two spots- this is used for when a \"hit\" occurs. If the projected distance becomes larger than the previous distance, the program will assume that the spot is being pulled from the buffer zone and as a result will allow the bubble to exit."
                  # "This subVI leads to the distance function, which outputs the distance between a spot being checked compared to the current spot number."
                  n536 = control-ref of="Value Check"() -> (w1635:refnum<vi>)
                  n537 = control-ref of="ID num check"() -> (w1634:refnum<vi>)
                  n538 = control-ref of="Spot Checker"() -> (w1651:refnum<vi>)
                  n539 = Subtract(x=w1644, y=w1655) -> (x-y=w1645:cluster{dbl, dbl, "Z":dbl})
                  n540 = call "DistanceFunction.vi"("Condition Driver"=FALSE, "Position (real coords)"=w1655, "Current Spot Number"=w1634, "Spot Checker"=w1651, "Spot Number Being Checked"=w1635) -> ("Distance"=w1619:dbl)  [unwired: 6 in]
                  n541 = stacked-sequence {
                    tunnel: w1619 -> [_ w1660]
                    frame #0 {
                      n542 = local read "Distance"() -> (→"Previous Distance":dbl)
                    }
                    frame #1 {
                      "Distance" <- w1660
                    }
                  }
                  n543 = Unbundle(w1645) -> (→"X Displacement":dbl, →"Y Displacement":dbl)  [unwired: 1 out]
                  n544 = control-ref of="ID num check"() -> (w1636:refnum<vi>)
                  n545 = control-ref of="Spot Checker"() -> (w1649:refnum<vi>)
                  n546 = control-ref of="Y Displacement"() -> (w1647:refnum<vi>)
                  n547 = control-ref of="Value Check"() -> (w1637:refnum<vi>)
                  n548 = control-ref of="X Displacement"() -> (w1648:refnum<vi>)
                  n549 = call "ProjectedDistance.vi"("X Displacement"=w1648, "Spot Number Check"=w1637, "Current Spot #"=w1636, "Spot Checker"=w1649, "Y Displacement"=w1647) -> ("Numeric"=→"Projected Distance":dbl)  [unwired: 6 in]
                  n550 = Multiply(x="Buffer Zone", y=2) -> (x*y=w1654:dbl)
                  n551 = local read "ID num check"() -> (w1631:dbl)
                  n552 = local read "Value Check"() -> (w1632:dbl)
                  n553 = local read "Projected Distance"() -> (w1623:dbl)
                  n554 = Equal?(x=w1619, y=0) -> (x = y?=w1620:bool)
                  n555 = case shown="False" w1620 {
                    frame False {
                      n556 = local read "Hit"() -> (w1657:bool)
                      n557 = local write "Hit Indicator"(w1657) -> ()
                    }
                    frame True {
                      "Hit Indicator" <- FALSE
                    }
                  }
                  n558 = Not Equal?(x=w1623, y=0) -> (x != y?=w1621:bool)
                  n559 = Less Or Equal?(x=w1619, y=w1654) -> (x <= y?=w1624:bool)
                  n560 = Equal?(x=w1631, y=w1630) -> (x = y?=w1629:bool)
                  n561 = And(x=w1624, y=w1621) -> (x .and. y?=w1617:bool)
                  "Hit" <- w1617
                  n562 = Equal?(x=w1630, y=w1632) -> (x = y?=w1628:bool)
                  n563 = Not(x=w1617) -> ()  [unwired: 1 out]
                  n564 = And(x=w1629, y=w1628) -> (x .and. y?=w1627:bool)
                  n565 = Or(x=w1617, y=w1627) -> (x .or. y?=w1633:bool)
                  n566 = case shown="True" w1633 {
                    frame False {
                      n567 = stacked-sequence {
                        frame #0 {
                          n568 = local read "Potential Collisions"() -> (w1663:dbl)
                          n569 = local read "Spot # Check"() -> (w1665:dbl)
                          n570 = Subtract(x=w1663, y=1) -> (x-y=w1661:dbl)
                          n571 = Less Or Equal?(x=w1665, y=w1661) -> (x <= y?=w1664:bool)
                          n572 = case shown="True" w1664 {
                            frame False {
                              # "Spot # Check resets if the the number of potential collisons is more than Spot # Check."
                              n573 = local write "Spot # Check"(0) -> ()
                            }
                            frame True {
                              n574 = stacked-sequence {
                                frame #0 {
                                # "Spot # Check increments by 1 every time it is greater than the # of potential collisions."
                                n575 = local read "Spot # Check"() -> (w1669:dbl)
                                n576 = Add(x=w1669, y=1) -> (x+y=→"Spot # Check":dbl)
                                }
                                frame #1 {
                                # "Spot # Check resets if the Spot # Check is eqaul to the # of potential collisions."
                                n577 = local read "Potential Collisions"() -> (w1670:dbl)
                                n578 = local read "Spot # Check"() -> (w1671:dbl)
                                n579 = Equal?(x=w1671, y=w1670) -> (x = y?=w1672:bool)
                                n580 = case shown="True" w1672 {
                                frame False {
                                }
                                frame True {
                                n581 = local write "Spot # Check"(0) -> ()
                                }
                                }
                                }
                                frame #2 {
                                n582 = local read "Spot Checker"() -> (w1687:T1[])
                                n583 = local read "Current Spot #"() -> (w1688:dbl)
                                n584 = local read "Area to check"() -> (w1674:dbl)
                                n585 = Index Array(array=w1687, index=w1688) -> (element=w1686:T1)
                                n586 = local read "Orig Y SC"() -> (w1683:dbl)
                                n587 = Unbundle By Name(w1686) -> ("Position.x"=w1684:dbl, "Position.y"=w1682:dbl)
                                n588 = local read "Orig X SC"() -> (w1685:dbl)
                                n589 = Subtract(x=w1682, y=w1683) -> (x-y=w1675:dbl)
                                n590 = Absolute Value(x=w1675) -> (abs(x)=w1676:dbl)
                                n591 = Subtract(x=w1684, y=w1685) -> (x-y=w1678:dbl)
                                n592 = Greater?(x=w1676, y=w1674) -> (0:w1680:bool)
                                n593 = Absolute Value(x=w1678) -> (abs(x)=w1677:dbl)
                                n594 = Greater?(x=w1677, y=w1674) -> (0:w1679:bool)
                                n595 = Or(x=w1679, y=w1680) -> (x .or. y?=w1681:bool)
                                n596 = case shown="True" w1681 {
                                frame False {
                                }
                                frame True {
                                n597 = stacked-sequence {
                                frame #0 {
                                n598 = local read "Null array"() -> (w1693:dbl[])
                                n599 = local write "What to Check"(w1693) -> ()
                                n600 = local write "ID"(w1693) -> ()
                                n601 = local read "Current Spot #"() -> (w1695:dbl)
                                n602 = local write "Potential Collisions"(0) -> ()
                                n603 = local read "Spot Checker"() -> (w1694:T1[])
                                n604 = Index Array(array=w1694, index=w1695) -> (element=w1696:T1)
                                n605 = Wait (ms)(milliseconds to wait=100) -> ()  [unwired: 1 out]
                                n606 = Unbundle By Name(w1696) -> ("Position.x"=w1690:dbl, "Position.y"=w1691:dbl)
                                n607 = local write "Orig Y SC"(w1691) -> ()
                                n608 = local write "Orig X SC"(w1690) -> ()
                                }
                                frame #1 {
                                # "All this is a  statement checking whether the microrobot is within the area being checked using absolute value statements. The number of potential collisions gets added by 1 every time a bubble is detected within the area."
                                n609 = local read "# of Spots"() -> (w1697:dbl)
                                n610 = for {
                                N: w1697 -> [_]
                                tunnel: w1697 -> [w1702]
                                i -> [w1698]
                                n611 = local read "Selection/Group"() -> (w1701:T7[])
                                n612 = Index Array(array=w1701, index=w1698) -> (element=w1700:T7)
                                n613 = Unbundle By Name(w1700) -> ("Selected"=w1699:bool)
                                n614 = case shown="True" w1699 {
                                tunnel: w1702 -> [_ w1704]
                                tunnel: w1698 -> [_ w1703]
                                frame False {
                                }
                                frame True {
                                n615 = for {
                                N: w1704 -> [_]
                                tunnel: w1703 -> [w1705]
                                i -> [w1706]
                                n616 = local read "Selection/Group"() -> (w1710:T7[])
                                n617 = Index Array(array=w1710, index=w1706) -> (element=w1709:T7)
                                n618 = Unbundle By Name(w1709) -> ("Selected"=w1707:bool)
                                n619 = Not(x=w1707) -> (.not. x?=w1708:bool)
                                n620 = case shown="True" w1708 {
                                tunnel: w1706 -> [_ w1714]
                                tunnel: w1705 -> [_ w1713]
                                tunnel: w1705 -> [_ w1712]
                                frame False {
                                }
                                frame True {
                                n621 = local read "Spot Checker"() -> (w1731:T1[])
                                n622 = Index Array(array=w1731, index=w1714) -> (element=w1732:T1)
                                n623 = Index Array(array=w1731, index=w1713) -> (element=w1730:T1)
                                n624 = Unbundle By Name(w1730) -> ("Position.x"=w1727:dbl, "Position.y"=w1723:dbl)
                                n625 = Unbundle By Name(w1732) -> ("Position.x"=w1724:dbl, "Position.y"=w1720:dbl)
                                n626 = local read "Area+ Buffer"() -> (w1711:dbl)
                                n627 = Subtract(x=w1727, y=w1711) -> (x-y=w1728:dbl)
                                n628 = Greater Or Equal?(x=w1724, y=w1728) -> (x >= y?=w1729:bool)
                                n629 = Add(x=w1723, y=w1711) -> (x+y=w1722:dbl)
                                n630 = Subtract(x=w1723, y=w1711) -> (x-y=w1721:dbl)
                                n631 = Add(x=w1727, y=w1711) -> (x+y=w1725:dbl)
                                n632 = Less Or Equal?(x=w1720, y=w1722) -> (x <= y?=w1719:bool)
                                n633 = Greater Or Equal?(x=w1720, y=w1721) -> (x >= y?=w1718:bool)
                                n634 = Less Or Equal?(x=w1724, y=w1725) -> (x <= y?=w1726:bool)
                                n635 = And(x=w1729, y=w1726) -> (x .and. y?=w1716:bool)
                                n636 = And(x=w1719, y=w1718) -> (x .and. y?=w1717:bool)
                                n637 = And(x=w1716, y=w1717) -> (x .and. y?=w1715:bool)
                                n638 = case shown="True" w1715 {
                                tunnel: w1714 -> [_ _]
                                tunnel: w1714 -> [_ w1734]
                                tunnel: w1712 -> [_ w1733]
                                frame False {
                                }
                                frame True {
                                n639 = stacked-sequence {
                                tunnel: w1734 -> [w1735 _]
                                tunnel: w1733 -> [w1736 _]
                                frame #0 {
                                n640 = local read "Potential Collisions"() -> (w1739:dbl)
                                n641 = local read "What to Check"() -> (w1740:dbl[])
                                n642 = Insert Into Array(array=w1740, index=w1739, new element=w1735) -> (w1741:dbl[])
                                n643 = local read "ID"() -> (w1738:dbl[])
                                n644 = local write "What to Check"(w1741) -> ()
                                n645 = Insert Into Array(array=w1738, index=w1739, new element=w1736) -> (w1737:dbl[])
                                n646 = local write "ID"(w1737) -> ()
                                }
                                frame #1 {
                                n647 = local read "Potential Collisions"() -> (w1744:dbl)
                                n648 = Add(x=w1744, y=1) -> (x+y=w1742:dbl)
                                n649 = local write "Potential Collisions"(w1742) -> ()
                                }
                                }
                                }
                                }
                                }
                                }
                                }
                                }
                                }
                                }
                                }
                                frame #2 {
                                n650 = local read "Current Spot #"() -> (w1745:dbl)
                                n651 = local write "Prev Current Spot"(w1745) -> ()
                                }
                                }
                                }
                                }
                                }
                              }
                            }
                          }
                        }
                        frame #1 {
                          # "This updates the ID and Value being checked at the beginning of IDs and values being checked."
                          n652 = local read "Spot # Check"() -> (w1748:dbl)
                          n653 = local read "What to Check"() -> (w1749:dbl[])
                          n654 = local read "ID"() -> (w1750:dbl[])
                          n655 = Index Array(array=w1750, index=w1748) -> (element=w1747:dbl)
                          n656 = Index Array(array=w1749, index=w1748) -> (element=w1746:dbl)
                          n657 = local write "Value Check"(w1746) -> ()
                          n658 = local write "ID num check"(w1747) -> ()
                        }
                      }
                    }
                    frame True {
                      n659 = stacked-sequence {
                        frame #0 {
                          # "This section activate a case statement which allows us to change the area being checked. Orig X/Y SC holds the position of the area to check and changes after the bubble exits the area beig checked."
                          # "This statement controls the areas selected and finds which bubbles needs to be checked. This activates when the bubble\nmoves out of the area specified."
                          n660 = local read "# of Spots"() -> (w1770:dbl)
                          n661 = local read "Current Spot #"() -> (w1769:dbl)
                          n662 = Subtract(x=w1770, y=1) -> (x-y=w1771:dbl)
                          n663 = Equal?(x=w1769, y=w1771) -> (x = y?=w1767:bool)
                          n664 = case shown="True" w1767 {
                            tunnel: [w1830 w1833] -> w1768
                            frame True {
                              n665 = local read "# of Spots"() -> (w1831:dbl)
                              n666 = Subtract(x=w1831, y=2) -> (x-y=w1830:dbl)
                            }
                            frame False {
                              n667 = local read "# of Spots"() -> (w1832:dbl)
                              n668 = Subtract(x=w1832, y=1) -> (x-y=w1833:dbl)
                            }
                          }
                          "Maximum" <- w1768
                          n669 = local read "Spot Checker"() -> (w1766:T1[])
                          n670 = local read "Current Spot #"() -> (w1765:dbl)
                          n671 = Index Array(array=w1766, index=w1765) -> (element=w1764:T1)
                          n672 = Unbundle By Name(w1764) -> ("Position.x"=w1763:dbl, "Position.y"=w1762:dbl)
                          n673 = local read "Orig Y SC"() -> (w1760:dbl)
                          n674 = local read "Orig X SC"() -> (w1761:dbl)
                          n675 = Subtract(x=w1762, y=w1760) -> (x-y=w1757:dbl)
                          n676 = Subtract(x=w1763, y=w1761) -> (x-y=w1759:dbl)
                          n677 = Absolute Value(x=w1757) -> (abs(x)=w1756:dbl)
                          n678 = Absolute Value(x=w1759) -> (abs(x)=w1758:dbl)
                          n679 = local read "Area to check"() -> (w1752:dbl)
                          n680 = local read "Area to check"() -> (w1751:dbl)
                          n681 = Greater?(x=w1758, y=w1752) -> (0:w1755:bool)
                          n682 = Greater?(x=w1756, y=w1751) -> (0:w1754:bool)
                          n683 = Or(x=w1755, y=w1754) -> (x .or. y?=w1753:bool)
                          n684 = case shown="True" w1753 {
                            frame False {
                            }
                            frame True {
                              n685 = stacked-sequence {
                                frame #0 {
                                # "A small time delay of 100 ms is provided to allow the data to pass throguh properly."
                                n686 = Wait (ms)(milliseconds to wait=100) -> ()  [unwired: 1 out]
                                n687 = local read "Null array"() -> (→"What to Check" →"ID":dbl[])
                                n688 = local read "Spot Checker"() -> (w1778:T1[])
                                n689 = local read "Current Spot #"() -> (w1777:dbl)
                                n690 = Index Array(array=w1778, index=w1777) -> (element=w1776:T1)
                                n691 = Unbundle By Name(w1776) -> ("Position.x"=→"Orig X SC":dbl, "Position.y"=→"Orig Y SC":dbl)
                                "Potential Collisions" <- 0
                                }
                                frame #1 {
                                n692 = local read "# of Spots"() -> (w1781:dbl)
                                n693 = for {
                                N: w1781 -> [_]
                                tunnel: w1781 -> [w1786]
                                i -> [w1782]
                                n694 = local read "Selection/Group"() -> (w1785:T7[])
                                n695 = Index Array(array=w1785, index=w1782) -> (element=w1784:T7)
                                n696 = Unbundle By Name(w1784) -> ("Selected"=w1783:bool)
                                n697 = case shown="True" w1783 {
                                tunnel: w1786 -> [_ w1788]
                                tunnel: w1782 -> [_ w1787]
                                frame False {
                                }
                                frame True {
                                n698 = for {
                                N: w1788 -> [_]
                                tunnel: w1787 -> [w1789]
                                i -> [w1790]
                                n699 = local read "Selection/Group"() -> (w1794:T7[])
                                n700 = Index Array(array=w1794, index=w1790) -> (element=w1793:T7)
                                n701 = Unbundle By Name(w1793) -> ("Selected"=w1791:bool)
                                n702 = Not(x=w1791) -> (.not. x?=w1792:bool)
                                n703 = case shown="True" w1792 {
                                tunnel: w1790 -> [_ w1798]
                                tunnel: w1789 -> [_ w1797]
                                tunnel: w1789 -> [_ w1796]
                                frame False {
                                }
                                frame True {
                                n704 = local read "Spot Checker"() -> (w1815:T1[])
                                n705 = Index Array(array=w1815, index=w1798) -> (element=w1816:T1)
                                n706 = Index Array(array=w1815, index=w1797) -> (element=w1814:T1)
                                n707 = Unbundle By Name(w1814) -> ("Position.x"=w1811:dbl, "Position.y"=w1807:dbl)
                                n708 = Unbundle By Name(w1816) -> ("Position.x"=w1808:dbl, "Position.y"=w1804:dbl)
                                n709 = local read "Area+ Buffer"() -> (w1795:dbl)
                                n710 = Subtract(x=w1811, y=w1795) -> (x-y=w1812:dbl)
                                n711 = Greater Or Equal?(x=w1808, y=w1812) -> (x >= y?=w1813:bool)
                                n712 = Add(x=w1807, y=w1795) -> (x+y=w1806:dbl)
                                n713 = Subtract(x=w1807, y=w1795) -> (x-y=w1805:dbl)
                                n714 = Add(x=w1811, y=w1795) -> (x+y=w1809:dbl)
                                n715 = Less Or Equal?(x=w1804, y=w1806) -> (x <= y?=w1803:bool)
                                n716 = Greater Or Equal?(x=w1804, y=w1805) -> (x >= y?=w1802:bool)
                                n717 = Less Or Equal?(x=w1808, y=w1809) -> (x <= y?=w1810:bool)
                                n718 = And(x=w1813, y=w1810) -> (x .and. y?=w1800:bool)
                                n719 = And(x=w1803, y=w1802) -> (x .and. y?=w1801:bool)
                                n720 = And(x=w1800, y=w1801) -> (x .and. y?=w1799:bool)
                                n721 = case shown="True" w1799 {
                                tunnel: w1798 -> [_ _]
                                tunnel: w1798 -> [_ w1818]
                                tunnel: w1796 -> [_ w1817]
                                frame False {
                                }
                                frame True {
                                n722 = stacked-sequence {
                                tunnel: w1818 -> [w1819 _]
                                tunnel: w1817 -> [w1820 _]
                                frame #0 {
                                n723 = local read "Potential Collisions"() -> (w1823:dbl)
                                n724 = local read "What to Check"() -> (w1824:dbl[])
                                n725 = Insert Into Array(array=w1824, index=w1823, new element=w1819) -> (w1825:dbl[])
                                n726 = local read "ID"() -> (w1822:dbl[])
                                n727 = Insert Into Array(array=w1822, index=w1823, new element=w1820) -> (w1821:dbl[])
                                n728 = local write "What to Check"(w1825) -> ()
                                n729 = local write "ID"(w1821) -> ()
                                }
                                frame #1 {
                                n730 = local read "Potential Collisions"() -> (w1828:dbl)
                                n731 = Add(x=w1828, y=1) -> (x+y=w1826:dbl)
                                n732 = local write "Potential Collisions"(w1826) -> ()
                                }
                                }
                                }
                                }
                                }
                                }
                                }
                                }
                                }
                                }
                                }
                              }
                            }
                          }
                        }
                        frame #1 {
                          n733 = local read "# of Spots"() -> (w1837:dbl)
                          n734 = Not Equal?(x=w1837, y=1) -> (x != y?=w1835:bool)
                          n735 = case shown="True" w1835 {
                            frame False {
                            }
                            frame True {
                              n736 = stacked-sequence {
                                frame #0 {
                                n737 = local read "Potential Collisions"() -> (w1840:dbl)
                                n738 = local read "Spot # Check"() -> (w1842:dbl)
                                n739 = Subtract(x=w1840, y=1) -> (x-y=w1838:dbl)
                                n740 = Less Or Equal?(x=w1842, y=w1838) -> (x <= y?=w1841:bool)
                                n741 = case shown="False" w1841 {
                                frame False {
                                n742 = local write "Spot # Check"(0) -> ()
                                }
                                frame True {
                                }
                                }
                                }
                                frame #1 {
                                n743 = local read "What to Check"() -> (w1848:dbl[])
                                n744 = local read "ID"() -> (w1846:dbl[])
                                n745 = local read "Spot # Check"() -> (w1844:dbl)
                                n746 = Index Array(array=w1848, index=w1844) -> (element=→"Value Check":dbl)
                                n747 = Index Array(array=w1846, index=w1844) -> (element=→"ID num check":dbl)
                                }
                              }
                            }
                          }
                        }
                      }
                    }
                  }
                  n748 = local read "Potential Collisions"() -> (w1625:dbl)
                  n749 = Subtract(x=w1625, y=1) -> (x-y=w1626:dbl)
                  n750 = local read "Hit"() -> (w1643:bool)
                  n751 = Equal?(x=w1638, y=w1626) -> (x = y?=w1642:bool)
                  n752 = Or(x=w1643, y=w1642) -> (x .or. y?=w1640:bool)
                }
                n753 = for {
                  tunnel: w1615 -> [w1862] mode=indexing
                  tunnel: w1616 -> [w1859] mode=indexing
                  tunnel: [w1861] -> w1610 mode=indexing
                  tunnel: w1612 -> [w1860]
                  # "If the projected distance is greater than the\nprevious distance, then the selected spots will move. \nThis situation only occurs if the bubble is about to/crossing \nthe buffer zone of another bubble. \n\nThe selected spots will also move if none of the bubbles\nare near/crossing the buffer zone of another bubble."
                  n754 = local read "Hit"() -> (w1852:bool)
                  n755 = Unbundle By Name(w1859) -> ()  [unwired: 1 out]
                  n756 = local read "Projected Distance"() -> (w1851:dbl)
                  n757 = Unbundle(w1862) -> ("Group ID"=→"Group ID #":i32, "Selected"=w1856:bool)
                  n758 = local read "Previous Distance"() -> (w1854:dbl)
                  n759 = Not(x=w1852) -> (.not. x?=w1850:bool)
                  n760 = Greater?(x=w1851, y=w1854) -> (0:w1853:bool)
                  n761 = And(x=w1852, y=w1853) -> (x .and. y?=w1849:bool)
                  n762 = Or(x=w1850, y=w1849) -> (x .or. y?=w1855:bool)
                  n763 = And(x=w1856, y=w1855) -> (x .and. y?=w1857:bool)
                  n764 = case shown="True" w1857 {
                    tunnel: w1859 -> [w1863 w1867]
                    tunnel: [w1863 w1866] -> w1861
                    tunnel: w1860 -> [_ w1868]
                    frame False {
                      # "otherwise, leave it alone!"
                    }
                    frame True {
                      # "If the spot is selected, move it by the same amount as the mouse"
                      n765 = call "extract_position.vi"("Spot"=w1867) -> ("Position"=w1865:cluster{"x":dbl, "y":dbl, "z":dbl})
                      n766 = Add(x=w1865, y=w1868) -> (x+y=w1864:cluster{dbl, dbl, dbl})
                      n767 = call "replace_position.vi"("Position"=w1864, "Spot in"=w1867) -> ("Spot"=w1866:T1)  [unwired: 2 out]
                    }
                  }
                }
                "Spot Checker" <- w1610
                n768 = local read "Locked Current Spot"() -> (w1606:dbl)
                n769 = Index Array(array=w1610, index=w1606) -> (element=w1609:T1)
                n770 = Unbundle By Name(w1609) -> ("Position.x"=→"New X":dbl, "Position.y"=→"New Y":dbl)  [unwired: 1 out]
                n771 = Array Size(array=w1610) -> (size(s)=→"# of Spots":i32)
              }
              frame True {
                # "coordinate conversion to find the rotation and scaling done by the mouse, about the centroid of the spots"
                n772 = Subtract(x=w1870, y=w1880) -> (x-y=w1889:cluster{dbl, dbl, dbl})
                n773 = Subtract(x=w1871, y=w1880) -> (x-y=w1888:cluster{dbl, dbl, dbl})
                n774 = Unbundle(w1888) -> (w1874:dbl, w1875:dbl)  [unwired: 1 out]
                n775 = Unbundle(w1889) -> (w1879:dbl, w1878:dbl)  [unwired: 1 out]
                n776 = Re/Im To Polar(2:w1875, 3:w1874) -> (0:w1872:dbl, 1:w1873:dbl)
                n777 = Re/Im To Polar(2:w1878, 3:w1879) -> (0:w1876:dbl, 1:w1877:dbl)
                n778 = Divide(x=w1873, y=w1877) -> (x/y=w1869:dbl)
                n779 = Subtract(x=w1872, y=w1876) -> (x-y=w1881:dbl)
                n780 = Bundle(w1869, w1869, w1869) -> (w1891:cluster{dbl, dbl, dbl})  [unwired: 1 out]
                n781 = call "scale_matrix.vi"("Scale Factors"=w1891) -> ("Scale Matrix"=w1887:T17)
                n782 = call "arb_rotation_matrix.vi"("Unit Vector"=cluster{dbl, dbl, dbl} {0.0, 0.0, 1.0}, "theta"=w1881) -> ("Real Matrix"=w1886:T17)
                n783 = call-poly <vilib>:"A x B.vi"("B"=w1886, "A"=w1887) -> ("A x B"=w1882:T17)  [unwired: 1 out]
                n784 = for {
                  tunnel: w1885 -> [w1897] mode=indexing
                  tunnel: [w1896] -> w1884 mode=indexing
                  tunnel: w1883 -> [w1895] mode=indexing
                  tunnel: w1880 -> [w1893]
                  tunnel: w1882 -> [w1892]
                  n785 = Unbundle(w1895) -> ("Selected"=w1894:bool)  [unwired: 1 out]
                  n786 = case shown="True" w1894 {
                    tunnel: w1897 -> [w1898 w1902]
                    tunnel: [w1898 w1901] -> w1896
                    tunnel: w1893 -> [_ w1900]
                    tunnel: w1892 -> [_ w1899]
                    frame False {
                    }
                    frame True {
                      n787 = call "apply_matrix_transformation_to_spots.vi"("Transform centre (i.e. transform about this point)"=w1900, "Transformation Matrix (3x3)"=w1899, "Spot In"=w1902) -> ("Spot Out"=w1901:T1)  [unwired: 5 out]
                    }
                  }
                }
              }
            }
          }
        }
        "Selection/Group" <- w1574
        n788 = Unbundle By Name(w1581) -> ("Position (Image Pixels)"=w1580:cluster{"X":dbl, "Y":dbl})
        n789 = Bundle By Name(cluster=w1581, "Dragging"=TRUE, "Previous Position (Image Pixels)"=w1580, "Position (Image Pixels)"=w1579) -> (w1590:T10)
      }
      event "stop": Value Change {
        n790 = event-data() -> ()  [unwired: 1 in, 4 out]
        n791 = global read "red_tweezers_globals_INTERNAL_VOLATILE.vi" "Current Settings File"() -> (w1906:path)
        n792 = call <vilib>:"Check if File or Folder Exists.vi"("path"=w1906) -> ("file or folder exists?"=w1905:bool)  [unwired: 8 in, 2 out]
        n793 = case shown="False" w1905 {
          tunnel: [w1913 w1917] -> w1907
          frame False {
            n794 = Two Button Dialog(message="Save current settings?", 1:"Don't Save" ("F button name (\"Cancel\")"), 2:"Save As..." ("T button name (\"OK\")")) -> (T button?=w1910:bool)
            n795 = Select(t=T14."Center Button" ("Which Button?"), s=w1910, f=T14."Right Button" ("Which Button?")) -> (s? t:f=w1913:T14)
          }
          frame True {
            n796 = call <vilib>:"Three Button Dialog.vi"("Allow user to close window? (TRUE)"=TRUE, "Window Title (\"\")"="Save Settings?" ("Window Title (\"\")"), "Right Button Text (\"Cancel\")"="No" ("Right Button Text (\"Cancel\")"), "Center Button Text (\"No\")"="Save As..." ("Center Button Text (\"No\")"), "Left Button Text (\"Yes\")"="Save" ("Left Button Text (\"Yes\")"), "message"="Would you like to save the current settings? You can choose to use the current settings file or save to a new location.") -> ("Which Button?"=w1917:T14)  [unwired: 5 in]
          }
        }
        n797 = case shown="\"Center Button\"" w1907 {
          tunnel: [TRUE TRUE FALSE FALSE] -> w1904
          frame "Left Button", Default {
          }
          frame "Center Button" {
            n798 = call "File Dialog5"("prompt"="Please select a location to save the settings", "button label"="Save", "default name"="red_tweezers_settings.xml", "pattern (all files)"="*.xml" ("pattern label"), "pattern label"="XML Settings Files") -> ("selected path"=w1925:path)  [unwired: 7 in, 3 out]
            n799 = global write "red_tweezers_globals_INTERNAL_VOLATILE.vi" "Current Settings File"(w1925) -> ()
          }
          frame "Right Button" {
          }
          frame "Window Close" {
          }
        }
        n800 = global write "red_tweezers_globals_INTERNAL_VOLATILE.vi" "Save Settings On Exit"(w1904) -> ()
      }
    }
    n801 = call "IMAQ Create"("Image Name"="untitled", "Image Type"=w46) -> ("New Image"=w45:T8)  [unwired: 3 in, 1 out]
    n802 = call "Vision Acquisition"() -> ("Image Out"=w43:T8)  [unwired: 25 in, 2 out]
    n803 = local read "Number of Matches Returned"() -> (w37:dbl)
    n804 = case shown="True" "Camera Capture" {
      frame False {
      }
      frame True {
        n805 = local read "Circles"() -> (w148:T9)
        n806 = Index Array(array=w148) -> (element=w147:T24)  [unwired: 1 in]
        n807 = Unbundle(w147) -> ("Position"=w146:cluster{"X":sgl, "Y":sgl})  [unwired: 2 out]
        n808 = Unbundle(w146) -> ("X"=→"Bubble x":sgl, "Y"=→"Bubble y":sgl)
      }
    }
    n809 = Add(x=w37, y=1.0 ("x+y")) -> (x+y=w39:dbl)
    n810 = call "IMAQ ExtractSingleColorPlane"("Color Plane"=w42, "Image Dst"=w45, "Image Src"=w43) -> ("Image Dst Out"=w40:T8)  [unwired: 7 in, 1 out]
    n811 = for {
      N: w39 -> [_]
      tunnel: w40 -> [w157]
      i -> [w153]
      n812 = local read "Circles"() -> (w169:T9)
      n813 = Number To Decimal String(number=w153) -> (decimal integer string=w152:string)  [unwired: 1 in]
      n814 = Index Array(array=w169) -> (element=w168:T24)  [unwired: 1 in]
      n815 = Unbundle(w168) -> ("Position"=w151:cluster{"X":sgl, "Y":sgl}, "Radius"=w167:dbl)  [unwired: 1 out]
      n816 = Unbundle(w151) -> ("X"=w155:sgl, "Y"=w154:sgl)
      n817 = Subtract(x=w155, y=w167) -> (x-y=→"toplx":dbl)
      n818 = Add(x=w155, y=w167) -> (x+y=→"bottomrx":dbl)
      n819 = Add(x=w154, y=w167) -> (x+y=→"bottomry":dbl)
      n820 = Subtract(x=w154, y=w167) -> (x-y=→"toply":dbl)
      n821 = local read "bottomry"() -> (w159:dbl)
      n822 = local read "bottomrx"() -> (w160:dbl)
      n823 = local read "toply"() -> (w161:dbl)
      n824 = local read "toplx"() -> (w162:dbl)
      n825 = Build Array(w162, w161, w160, w159) -> (w156:dbl[])
      n826 = Array To Cluster(array=w156) -> (cluster=w158:T25)
      n827 = call "IMAQ Overlay Oval"("Bounding Rectangle"=w158, "Image"=w157) -> ("Image Out"=w150:T8)  [unwired: 8 in, 1 out]
      n828 = call "IMAQ Overlay Text"("String"=w152, "Origin"=w151, "Image"=w150) -> ("Image Out"=→"Camera 2":T8)  [unwired: 7 in, 1 out]
    }
    n829 = case shown="True" "Lock Current Spot" {
      frame False {
      }
      frame True {
        n830 = global read "red_tweezers_globals.vi" "Spots"() -> (w473:T1[])
        n831 = local read "Current Spot #"() -> (w474:dbl)
        "Locked Current Spot" <- w474
        n832 = Index Array(array=w473, index=w474) -> (element=w475:T1)
        n833 = local write "LCS"(0) -> ()
        n834 = Unbundle By Name(w475) -> ("Position.x"=w471:dbl, "Position.y"=w470:dbl)
        n835 = local write "Original Y"(w470) -> ()
        n836 = local write "Original X"(w471) -> ()
      }
    }
    n837 = call-poly "IMAQ Detect Shapes"("Image"=w40) -> ("Number of Matches Returned"=→"Number of Matches Returned":i32, "Circles"=→"Circles":T9)  [unwired: 8 in, 1 out]
    n838 = case shown="True" "Mark Original Position" {
      frame False {
      }
      frame True {
        w476 = TRUE
        n839 = local read "1 for original positon"() -> (w478:dbl)
        n840 = local write "Mark Original Position"(FALSE) -> ()
        n841 = Add(x=w478, y=1) -> (x+y=w477:dbl)
        n842 = local write "1 for original positon"(w477) -> ()
        n843 = local read "New X"() -> (→"Original X":dbl)
        n844 = local read "New Y"() -> (→"Original Y":dbl)
        "MOP pressed After" <- w476
        "MOP pressed" <- w476
      }
    }
    n845 = case shown="True" "Rates" {
      frame False {
      }
      frame True {
        n846 = stacked-sequence {
          frame #0 {
            n847 = local read "Tab Control"() -> (w365:enum32{"Line", "Arc"})
            n848 = case shown="\"Line\"" w365 {
              tunnel: "Number of Planned Sequence Frames" -> [w366 w384]
              frame "Arc" {
                n849 = stacked-sequence {
                  tunnel: w366 -> [_ w379 _]
                  frame #0 {
                    n850 = expression code="(x/180.0)*pi" "degrees to radians"("Theta") -> (→"Radians":dbl)
                    n851 = local read "Radians"() -> (w378:dbl)
                    n852 = local read "Original Y"() -> (w372:dbl)
                    n853 = local read "Original X"() -> (w370:dbl)
                    n854 = Cosine(x=w378) -> (cos(x)=w367:dbl)
                    n855 = Sine(x=w378) -> (sin(x)=w369:dbl)
                    n856 = Multiply(x=w367, y="Radius X") -> (x*y=w371:dbl)
                    n857 = Multiply(x="Radius X", y=w369) -> (x*y=w373:dbl)
                    n858 = Subtract(x=w370, y=w371) -> (x-y=→"Center X":dbl)
                    n859 = Subtract(x=w372, y=w373) -> (x-y=→"Center Y":dbl)
                  }
                  frame #1 {
                    n860 = local read "Radians"() -> (w383:dbl)
                    n861 = Subtract(x=w379, y=1) -> (x-y=w381:dbl)
                    n862 = Divide(x=w383, y=w381) -> (x/y=→"Degree Rate":dbl)
                  }
                  frame #2 {
                  }
                }
              }
              frame "Line" {
                n863 = local read "Original X"() -> (w394:dbl)
                n864 = local read "Original Y"() -> (w392:dbl)
                n865 = Subtract(x=w384, y=1) -> (x-y=w386:dbl)
                n866 = local read "New Y"() -> (w391:dbl)
                n867 = local read "New X"() -> (w393:dbl)
                n868 = Subtract(x=w392, y=w391) -> (x-y=w389:dbl)
                n869 = Subtract(x=w394, y=w393) -> (x-y=w390:dbl)
                n870 = Divide(x=w389, y=w386) -> (x/y=→"Y Rate":dbl)
                n871 = Divide(x=w390, y=w386) -> (x/y=→"X Rate":dbl)
              }
            }
          }
          frame #1 {
            n872 = local write "Rates"(0) -> ()
          }
        }
      }
    }
    n873 = case shown="True" "Send Data" {
      frame False {
      }
      frame True {
        # "Pass data from Image Assistant to \nRed Tweezer New X & Y position"
        n874 = local read "Bubble y"() -> (w170:dbl)
        n875 = local read "Bubble x"() -> (w171:dbl)
        n876 = local write "New Y"(w170) -> ()
        n877 = local write "New X"(w171) -> ()
      }
    }
    n878 = local read "Sequence Instances"() -> (w102:dbl)
    n879 = case shown="True" w121 {
      tunnel: w127 -> [_ w544]
      frame False {
      }
      frame True {
        n880 = global write "red_tweezers_globals_INTERNAL.vi" "Image Overlay (extras from control loop)"(w544) -> ()
      }
    }
    n881 = local read "Counter"() -> (w101:dbl)
    n882 = call "red_tweezers_UNDO.vi"("Force Save"=w123, "This change is inconsequential (don't save it)"=w124, "Selection/Group"=w125, "Spots"=w126) -> ()  [unwired: 6 in, 2 out]
    n883 = call "sync_with_globals.vi"("Selection/Group"=w125, "Spots"=w126) -> ("Selection/Group 2"=w137:T7[], "Spots 2"=w88:T1[])  [unwired: 4 in]
    n884 = local read "Sequence Storer"() -> (w97:T1[][])
    n885 = local read "Sequence On?"() -> (w100:bool)
    n886 = local read "Sequence On?"() -> (w115:bool)
    n887 = call "SequenceControl.vi"("Sequence On? 2"=w100, "Counter 2"=w101, "Sequence Instances 2"=w102, "Sequence Storer"=w97) -> ("Time per Frame (ms) 2"=w95:dbl, "Sequence Order 2"=w98:dbl, "Reset 2"=w99:bool, "Sequence Storer 2"=w110:T1[][], "Clearance Button 2"=w109:bool, "Manual Edit 2"=w108:bool, "Save State 2"=w107:bool, "Play Sequence 2"=w104:bool, "Bubble ID to Empty 2"=w103:dbl, "Manual Sequence 2"=w105:bool, "Edit Sequence Mode 2"=w106:bool)  [unwired: 1 in]
    n888 = local write "Play Sequence"(w104) -> ()
    n889 = local write "Bubble ID to Empty"(w103) -> ()
    n890 = local write "Manual Sequence"(w105) -> ()
    n891 = local write "Reset"(w99) -> ()
    n892 = local write "Edit Sequence Mode"(w106) -> ()
    n893 = local write "Clearance Button"(w109) -> ()
    n894 = local write "Sequence Storer"(w110) -> ()
    n895 = local write "Save State"(w107) -> ()
    n896 = local write "Manual Edit"(w108) -> ()
    n897 = Or(x=w115, y="Manual Sequence") -> (x .or. y?=w114:bool)
    n898 = local write "Time per Frame (ms)"(w95) -> ()
    n899 = case shown="False" w114 {
      tunnel: [w514 w519] -> w118
      tunnel: w88 -> [w513 _]
      frame False {
        n900 = Or(x="Manual Edit", y="Edit Sequence Mode") -> (x .or. y?=w512:bool)
        n901 = case shown="False" w512 {
          tunnel: w513 -> [w515 _]
          tunnel: [w515 w516] -> w514
          frame False {
          }
          frame True {
            n902 = local read "Sequence Order"() -> (w517:dbl)
            n903 = local read "Sequence Storer"() -> (w518:T1[][])
            n904 = Index Array(array=w518, index (row)=w517) -> (element=w516:T1[])  [unwired: 1 in]
          }
        }
      }
      frame True {
        n905 = stacked-sequence {
          tunnel: [w521 _] -> w519
          frame #0 {
            n906 = local read "Counter"() -> (w522:dbl)
            n907 = local read "Sequence Storer"() -> (w523:T1[][])
            n908 = Index Array(array=w523, index (row)=w522) -> (element=w521:T1[])  [unwired: 1 in]
            n909 = Wait (ms)(milliseconds to wait="Time per Frame (ms)") -> ()  [unwired: 1 out]
          }
          frame #1 {
            n910 = local read "Sequence Instances"() -> (w525:dbl)
            n911 = local read "Counter"() -> (w528:dbl)
            n912 = Subtract(x=w525, y=1) -> (x-y=w526:dbl)
            n913 = Equal?(x=w528, y=w526) -> (x = y?=w527:bool)
            n914 = case shown="True" w527 {
              frame False {
                n915 = local read "Counter"() -> (w531:dbl)
                n916 = Add(x=w531, y=1) -> (x+y=→"Counter":dbl)
              }
              frame True {
                w532 = FALSE
                n917 = local write "Counter"(0) -> ()
                n918 = local write "Play Sequence"(w532) -> ()
                n919 = local write "Sequence On?"(w532) -> ()
              }
            }
          }
        }
      }
    }
    n920 = case shown="True" "Save State" {
      tunnel: w88 -> [_ w535]
      frame False {
      }
      frame True {
        n921 = local write "Save State"(FALSE) -> ()
        n922 = stacked-sequence {
          tunnel: w535 -> [w536 _]
          frame #0 {
            "Spot Storage" <- w536
          }
          frame #1 {
            n923 = local read "Spot Storage"() -> (w542:T1[])
            n924 = Replace Array Subset(array="Sequence Storer", new element=w542, index (row)="Sequence Order") -> (w540:T1[][])  [unwired: 1 in]
            n925 = Array Size(array=w540) -> (size(s)=w539:i32[])
            n926 = local write "Sequence Storer"(w540) -> ()
            n927 = Index Array(array=w539, index=0) -> (element=→"Sequence Instances":i32)
          }
        }
      }
    }
    n928 = feedback #10() -> (w142:T26)  [unwired: 1 out]
    n929 = call "Smoothed Frame Rate.vi"("Feedback In"=w142) -> ("Feedback Out"=w141:T26, "Frame Rate"=→"Interface Frame Rate":dbl)  [unwired: 1 in, 4 out]
    n930 = feedback-in #10(w141) -> ()
    n931 = local write "Sequence Order"(w98) -> ()
    n932 = case shown="True" "Clearance Button" {
      frame False {
      }
      frame True {
        # "This is the Bubble ID to Empty tool- this \"deletes\" the bubble in a sequence."
        n933 = local read "Sequence Order"() -> (w505:dbl)
        n934 = local read "Sequence Storer"() -> (w506:T1[][])
        n935 = Replace Array Subset(array=w506, new element=T11 {"Position"={"x"=nan, "y"=nan, "z"=nan}, "Intensity"=1.0, "Vortex Charge"=1, "Phase"=1.0, "NA Position"={"x"=0.0, "y"=0.0, "r"=1.0}, "Line Trapping"={"Vector"={"x"=0.0, "y"=0.0, "z"=0.0}, "Phase Gradient"=0.0}, "Amplitude Correction"=0.0} ("Cluster"), index (row)=w505, index (col)="Bubble ID to Empty") -> (w502:T1[][])
        n936 = local write "Sequence Storer"(w502) -> ()
      }
    }
    n937 = Not(x=w91) -> (.not. x?=w92:bool)
    n938 = Not(x="Output to SLM") -> (.not. x?=w93:bool)
    n939 = case shown="True" "Save" {
      frame False {
      }
      frame True {
        n940 = local read "Sequence Storer"() -> (w469:T1[][])
        n941 = call "SequenceSaver.vi"("Sequence Storer"=w469) -> ()  [unwired: 10 in, 1 out]
      }
    }
    n942 = And(x=w93, y=w92) -> (x .and. y?=w96:bool)
    n943 = case shown="True" "Load" {
      frame False {
      }
      frame True {
        n944 = call "SequenceSaver.vi"() -> ("Sequence Storer 2"=w468:T1[][])  [unwired: 11 in]
        n945 = local write "Sequence Storer"(w468) -> ()
      }
    }
    n946 = case shown="True" w96 {
      tunnel: w88 -> [w1934 _]
      frame False {
        n947 = call "UDP Sender generic_2.vi"("Spots"=w1934) -> ()  [unwired: 2 in, 1 out]
      }
      frame True {
      }
    }
    n948 = case shown="True" "Reset" {
      frame False {
      }
      frame True {
        n949 = local write "Counter"(0) -> ()
      }
    }
    n950 = case shown="True" "Add Additional Frames" {
      frame False {
      }
      frame True {
        # "This adds additional frames to the sequence."
        n951 = for {
          N: "Additional Frames Wanted" -> [_]
          i -> [w485]
          n952 = local read "Max Number of Bubbles"() -> (w489:dbl)
          n953 = Add(x=1, y=w485) -> (x+y=w486:i32)
          n954 = Add(x="Frame Location", y=w486) -> (x+y=w487:dbl)
          n955 = Initialize Array(T11 {"Position"={"x"=nan, "y"=nan, "z"=nan}, "Intensity"=1.0, "Vortex Charge"=1, "Phase"=1.0, "NA Position"={"x"=0.0, "y"=0.0, "r"=1.0}, "Line Trapping"={"Vector"={"x"=0.0, "y"=0.0, "z"=0.0}, "Phase Gradient"=0.0}, "Amplitude Correction"=0.0} ("Cluster"), w489) -> (w490:T27)
          n956 = local read "Sequence Storer"() -> (w491:T1[][])
          n957 = Insert Into Array(array=w491, index (row)=w487, new element=w490) -> (w492:T1[][])  [unwired: 1 in]
          n958 = local write "Sequence Storer"(w492) -> ()
        }
      }
    }
    n959 = case shown="True" "Initiate Creation" {
      frame False {
      }
      frame True {
        # "This create the array needed for a sequential\narray."
        n960 = local read "Number of Planned Sequence Frames"() -> (w495:dbl)
        n961 = for {
          N: w495 -> [_]
          tunnel: "Max Number of Bubbles" -> [w496]
          i -> [w499]
          n962 = Initialize Array(T11 {"Position"={"x"=nan, "y"=nan, "z"=nan}, "Intensity"=1.0, "Vortex Charge"=1, "Phase"=1.0, "NA Position"={"x"=0.0, "y"=0.0, "r"=1.0}, "Line Trapping"={"Vector"={"x"=0.0, "y"=0.0, "z"=0.0}, "Phase Gradient"=0.0}, "Amplitude Correction"=0.0} ("Cluster"), w496) -> (w497:T27)
          n963 = local read "Sequence Storer"() -> (w500:T1[][])
          n964 = Insert Into Array(array=w500, index (row)=w499, new element=w497) -> (w501:T1[][])  [unwired: 1 in]
          n965 = local write "Sequence Storer"(w501) -> ()
        }
      }
    }
    n966 = case shown="False" "Play Sequence" {
      frame False {
        n967 = local write "Sequence On?"(FALSE) -> ()
      }
      frame True {
        "Sequence On?" <- TRUE
      }
    }
    n968 = local read "Current Spot #"() -> (w71:dbl)
    n969 = local read "Selection/Group"() -> (w72:T7[])
    n970 = local read "# of Spots"() -> (w87:dbl)
    n971 = Not Equal?(x=w71, y=-1) -> (x != y?=w73:bool)
    n972 = local read "spots selected 2"() -> (w61:i32)
    n973 = Index Array(array=w72, index=w71) -> (element=w70:T7)
    n974 = Unbundle By Name(w70) -> ("Selected"=w69:bool)
    n975 = local read "spots selected"() -> (w62:i32)
    n976 = Not(x=w69) -> (.not. x?=w68:bool)
    n977 = And(x=w68, y=w73) -> (x .and. y?=w63:bool)
    n978 = Less?(x=w62, y=w61) -> (x < y?=w59:bool)
    n979 = case shown="True" "Insert" {
      tunnel: w88 -> [_ w173]
      tunnel: w87 -> [_ w172]
      frame False {
      }
      frame True {
        n980 = for {
          N: w172 -> [_]
          tunnel: w173 -> [w175]
          i -> [w174]
          n981 = stacked-sequence {
            tunnel: w175 -> [w177 w182 _]
            tunnel: w174 -> [_ w178 _]
            frame #0 {
              n982 = local read "Start at Which Frame?"() -> (→"Num":dbl)
              "Spot Storage 2" <- w177
            }
            frame #1 {
              n983 = local read "Selection/Group"() -> (w181:T7[])
              n984 = Index Array(array=w181, index=w178) -> (element=w180:T7)
              n985 = Unbundle By Name(w180) -> ("Selected"=w179:bool)
              n986 = case shown="True" w179 {
                tunnel: w182 -> [_ _]
                frame False {
                }
                frame True {
                  n987 = stacked-sequence {
                    frame #0 {
                      n988 = case shown="\"Line\"" "Tab Control" {
                        frame "Arc" {
                          n989 = local read "How Many Frames?"() -> (w186:dbl)
                          n990 = Subtract(x=w186, y=1) -> (x-y=w184:dbl)
                          n991 = for {
                            N: w186 -> [_]
                            tunnel: w184 -> [w187]
                            i -> [w189]
                            # "What is this ^\n\nFor # of sequence\nframes, don't worry\nabout it"
                            # "How to make position x and y?\nIt's called a cluster, inser the new position to Position.x and Position.y"
                            n992 = Equal?(x=w187, y=w189) -> (x = y?=w188:bool)
                            n993 = case shown="False" w188 {
                              tunnel: [w212 w221] -> w191
                              tunnel: [w211 w220] -> w190
                              tunnel: w189 -> [w208 _]
                              frame False {
                                # "calculating new position"
                                n994 = local read "Degree Rate"() -> (w210:dbl)
                                n995 = Multiply(x=w210, y=w208) -> (x*y=w209:dbl)
                                n996 = Cosine(x=w209) -> (cos(x)=w218:dbl)
                                n997 = Sine(x=w209) -> (sin(x)=w219:dbl)
                                n998 = local read "Radius X"() -> (w217:dbl)
                                n999 = Multiply(x=w217, y=w219) -> (x*y=w216:dbl)
                                n1000 = Multiply(x=w218, y=w217) -> (x*y=w215:dbl)
                                n1001 = local read "Center X"() -> (w214:dbl)
                                n1002 = local read "Center Y"() -> (w213:dbl)
                                n1003 = Add(x=w214, y=w215) -> (x+y=w212:dbl)
                                n1004 = Add(x=w213, y=w216) -> (x+y=w211:dbl)
                              }
                              frame True {
                                n1005 = global read "red_tweezers_globals.vi" "Spots"() -> (w224:T1[])
                                n1006 = local read "Numeric"() -> (w223:dbl)
                                n1007 = Index Array(array=w224, index=w223) -> (element=w222:T1)
                                n1008 = Unbundle By Name(w222) -> ("Position.x"=w221:dbl, "Position.y"=w220:dbl)
                              }
                            }
                            n1009 = local read "Spot Storage 2"() -> (w207:T1[])
                            n1010 = local read "Numeric"() -> (w206:dbl)
                            n1011 = Index Array(array=w207, index=w206) -> (element=w193:T1)
                            n1012 = local read "Start at Which Frame?"() -> (w195:dbl)
                            n1013 = Bundle By Name(cluster=w193, "Position.x"=w191, "Position.y"=w190) -> (w192:T1)
                            n1014 = local read "How Many Frames?"() -> (w194:dbl)
                            n1015 = Subtract(x=w195, y=w189) -> (x-y=w204:dbl)
                            n1016 = local read "Sequence Storer"() -> (w205:T1[][])
                            n1017 = local read "Numeric"() -> (w200:dbl)
                            n1018 = Add(x=w204, y=w194) -> (x+y=w203:dbl)
                            n1019 = Subtract(x=w203, y=1) -> (x-y=w201:dbl)
                            n1020 = Replace Array Subset(array=w205, new element=w192, index (row)=w201, index (col)=w200) -> (w199:T1[][])
                            n1021 = Array Size(array=w199) -> (size(s)=w198:i32[])
                            n1022 = local write "Sequence Storer"(w199) -> ()
                            n1023 = Index Array(array=w198, index=0) -> (element=w196:i32)
                            n1024 = local write "Sequence Instances"(w196) -> ()
                          }
                        }
                        frame "Line" {
                          n1025 = local read "Rates"() -> (w225:dbl)
                          n1026 = case shown="0" w225 {
                            frame 1, Default {
                              # "This is the automatic sequence generator which allows for the creation of the sequence. This calculates the LAST coordinates of each bubble first\nbefore going for the first few coordinates of the sequence."
                              n1027 = local read "How Many Frames?"() -> (w226:dbl)
                              n1028 = for {
                                N: w226 -> [_]
                                i -> [w238]
                                # "For why do we multiply?"
                                n1029 = local read "Spot Storage 2"() -> (w239:T1[])
                                n1030 = local read "Numeric"() -> (w229:dbl)
                                n1031 = local read "X Rate"() -> (w245:dbl)
                                n1032 = local read "Y Rate"() -> (w244:dbl)
                                n1033 = Index Array(array=w239, index=w229) -> (element=w236:T1)
                                n1034 = Unbundle By Name(w236) -> ("Position.x"=w246:dbl, "Position.y"=w242:dbl)
                                n1035 = Multiply(x=w245, y=w238) -> (x*y=w243:dbl)
                                n1036 = Multiply(x=w244, y=w238) -> (x*y=w237:dbl)
                                n1037 = local read "Start at Which Frame?"() -> (w228:dbl)
                                n1038 = Subtract(x=w246, y=w243) -> (x-y=w241:dbl)
                                n1039 = Subtract(x=w242, y=w237) -> (x-y=w240:dbl)
                                n1040 = Bundle By Name(cluster=w236, "Position.x"=w241, "Position.y"=w240) -> (w231:T1)
                                n1041 = Add(x=w228, y=w238) -> (x+y=w227:dbl)
                                n1042 = local read "Sequence Storer"() -> (w247:T1[][])
                                n1043 = local read "Numeric"() -> (w230:dbl)
                                n1044 = Replace Array Subset(array=w247, new element=w231, index (row)=w227, index (col)=w230) -> (w235:T1[][])
                                n1045 = Array Size(array=w235) -> (size(s)=w234:i32[])
                                n1046 = local write "Sequence Storer"(w235) -> ()
                                n1047 = Index Array(array=w234, index=0) -> (element=w232:i32)
                                n1048 = local write "Sequence Instances"(w232) -> ()
                              }
                            }
                            frame 0 {
                              # "This is the automatic sequence generator which allows for the creation of the sequence. This calculates the LAST coordinates of each bubble first\nbefore going for the first few coordinates of the sequence."
                              n1049 = local read "How Many Frames?"() -> (w248:dbl)
                              n1050 = for {
                                N: w248 -> [_]
                                i -> [w263]
                                # "For why do we multiply?"
                                n1051 = local read "Spot Storage 2"() -> (w265:T1[])
                                n1052 = local read "Numeric"() -> (w249:dbl)
                                n1053 = local read "X Rate"() -> (w271:dbl)
                                n1054 = local read "Y Rate"() -> (w270:dbl)
                                n1055 = Index Array(array=w265, index=w249) -> (element=w256:T1)
                                n1056 = Unbundle By Name(w256) -> ("Position.x"=w272:dbl, "Position.y"=w268:dbl)
                                n1057 = Multiply(x=w271, y=w263) -> (x*y=w269:dbl)
                                n1058 = Multiply(x=w270, y=w263) -> (x*y=w257:dbl)
                                "probe" <- w257
                                n1059 = Subtract(x=w272, y=w269) -> (x-y=w267:dbl)
                                n1060 = Subtract(x=w268, y=w257) -> (x-y=w266:dbl)
                                n1061 = Bundle By Name(cluster=w256, "Position.x"=w267, "Position.y"=w266) -> (w251:T1)
                                n1062 = Subtract(x="Start at Which Frame?", y=w263) -> (x-y=w262:dbl)
                                n1063 = local read "Sequence Storer"() -> (w273:T1[][])
                                n1064 = local read "Numeric"() -> (w250:dbl)
                                n1065 = local read "How Many Frames?"() -> (w261:dbl)
                                n1066 = Add(x=w262, y=w261) -> (x+y=w260:dbl)
                                n1067 = Subtract(x=w260, y=1) -> (x-y=w258:dbl)
                                n1068 = Replace Array Subset(array=w273, new element=w251, index (row)=w258, index (col)=w250) -> (w255:T1[][])
                                n1069 = Array Size(array=w255) -> (size(s)=w254:i32[])
                                n1070 = local write "Sequence Storer"(w255) -> ()
                                n1071 = Index Array(array=w254, index=0) -> (element=w252:i32)
                                n1072 = local write "Sequence Instances"(w252) -> ()
                              }
                            }
                          }
                        }
                      }
                    }
                    frame #1 {
                      n1073 = local read "How Many Frames?"() -> (w274:dbl)
                      n1074 = for {
                        N: w274 -> [_]
                        n1075 = stacked-sequence {
                          frame #0 {
                            n1076 = local read "Sequence Storer"() -> (w277:T1[][])
                            n1077 = local read "Num"() -> (w276:dbl)
                            n1078 = local read "# of Spots"() -> (w280:dbl)
                            n1079 = Index Array(array=w277, index (row)=w276) -> (element=w275:T1[])  [unwired: 1 in]
                            n1080 = Add(x=1, y=w276) -> (x+y=w278:dbl)
                            n1081 = for {
                              N: w280 -> [_]
                              tunnel: w280 -> [w284]
                              tunnel: w278 -> [w283]
                              tunnel: w275 -> [w282]
                              i -> [w281]
                              n1082 = stacked-sequence {
                                tunnel: w284 -> [w286 _]
                                tunnel: w283 -> [w290 _]
                                tunnel: w282 -> [w289 _]
                                tunnel: w281 -> [w288 _]
                                frame #0 {
                                n1083 = local read "LCounter"() -> (w285:dbl)
                                n1084 = Subtract(x=w286, y=w285) -> (x-y=w287:dbl)
                                n1085 = for {
                                N: w287 -> [_]
                                tunnel: w289 -> [w313]
                                tunnel: w288 -> [w294]
                                tunnel: w289 -> [w312]
                                tunnel: w290 -> [w299]
                                i -> [w293]
                                # "This checks whether a bubble intersects with another\nor not."
                                n1086 = local read "LCounter"() -> (w291:dbl)
                                n1087 = Add(x=w291, y=w293) -> (x+y=w292:dbl)
                                "Numeric 4" <- w292
                                n1088 = Index Array(array=w313, index=w292) -> (element=w314:T1)
                                n1089 = Index Array(array=w312, index=w294) -> (element=w315:T1)
                                n1090 = Unbundle By Name(w314) -> ("Position.x"=w310:dbl, "Position.y"=w308:dbl)
                                n1091 = Unbundle By Name(w315) -> ("Position.x"=w311:dbl, "Position.y"=w309:dbl)
                                n1092 = Subtract(x=w309, y=w308) -> (x-y=w306:dbl)
                                n1093 = Subtract(x=w311, y=w310) -> (x-y=w307:dbl)
                                n1094 = Square(x=w306) -> (x^2=w304:dbl)
                                n1095 = Square(x=w307) -> (x^2=w305:dbl)
                                n1096 = local write "Num"(w299) -> ()
                                n1097 = local read "Buffer Zone"() -> (w302:dbl)
                                n1098 = Add(x=w305, y=w304) -> (x+y=w303:dbl)
                                n1099 = Square Root(x=w303) -> (sqrt(x)=w296:dbl)
                                n1100 = Multiply(x=2, y=w302) -> (x*y=w300:dbl)
                                n1101 = Less Or Equal?(x=w296, y=w300) -> (x <= y?=w298:bool)
                                n1102 = Not Equal?(x=w294, y=w292) -> (x != y?=w295:bool)
                                n1103 = And(x=w295, y=w298) -> (x .and. y?=w297:bool)
                                n1104 = case shown="True" w297 {
                                tunnel: w299 -> [_ w316]
                                frame False {
                                }
                                frame True {
                                n1105 = stacked-sequence {
                                tunnel: w316 -> [w327 _]
                                frame #0 {
                                # "This prints the string which displays the information whether there are potential collisions\nor not."
                                n1106 = Subtract(x=w327, y=1) -> (x-y=w326:dbl)
                                n1107 = local read "Array"() -> (w324:dbl[])
                                n1108 = Insert Into Array(array=w324, index=0, new element=w326) -> (w317:dbl[])
                                "Array" <- w317
                                n1109 = Array Size(array=w317) -> (size(s)=w318:i32)
                                n1110 = Number To Decimal String(number=w318) -> (decimal integer string=w323:string)  [unwired: 1 in]
                                n1111 = Concatenate Strings("There are ", w323) -> (w321:string)
                                n1112 = Concatenate Strings(w321, " potential collisions in the sequence. Please examine the array to obtain the sequence numbers that need to be edited.") -> (→"Collision Detector":string)
                                }
                                frame #1 {
                                n1113 = stacked-sequence {
                                frame #0 {
                                n1114 = local read "Array"() -> (w330:dbl[])
                                n1115 = Array Size(array=w330) -> (size(s)=w329:i32)
                                n1116 = for {
                                N: w329 -> [_]
                                tunnel: w329 -> [w332]
                                tunnel: w329 -> [w331]
                                n1117 = stacked-sequence {
                                tunnel: [w350 _] -> _
                                tunnel: w332 -> [w345 _]
                                tunnel: w331 -> [_ _]
                                frame #0 {
                                n1118 = local read "Counter for String"() -> (w349:dbl)
                                n1119 = local read "Array"() -> (w350:dbl[])
                                n1120 = Multiply(x=w345, y=3) -> (x*y=w342:i32)
                                n1121 = Index Array(array=w350, index=w349) -> (element=w340:dbl)
                                n1122 = Subtract(x=w342, y=2) -> (x-y=w335:i32)
                                n1123 = Number To Decimal String(number=w340) -> (decimal integer string=w341:string)  [unwired: 1 in]
                                n1124 = local read "String counter"() -> (w333:dbl)
                                n1125 = local read "String 2"() -> (w347:string)
                                n1126 = Concatenate Strings(w341, ", ") -> (w348:string)
                                n1127 = Greater?(x=w340, y=9) -> (0:w337:bool)
                                n1128 = Add(x=w333, y=w335) -> (x+y=w336:dbl)
                                n1129 = Concatenate Strings(w348, w347) -> (w334:string)
                                "String 2" <- w334
                                n1130 = case shown="True" w337 {
                                frame False {
                                }
                                frame True {
                                n1131 = local read "String counter"() -> (w351:dbl)
                                n1132 = Add(x=w351, y=1) -> (x+y=→"String counter":dbl)
                                }
                                }
                                n1133 = Replace Substring(2:w336, 5:w334) -> (0:w339:string)  [unwired: 2 in, 1 out]
                                n1134 = local write "Sequence Frames To Check"(w339) -> ()
                                }
                                frame #1 {
                                n1135 = local read "Counter for String"() -> (w354:dbl)
                                n1136 = Add(x=w354, y=1) -> (x+y=w356:dbl)
                                n1137 = local write "Counter for String"(w356) -> ()
                                }
                                }
                                }
                                }
                                frame #1 {
                                w357 = 0
                                n1138 = local write "String counter"(w357) -> ()
                                "Counter for String" <- w357
                                }
                                }
                                }
                                }
                                }
                                }
                                "Numeric 3" <- w299
                                }
                                }
                                frame #1 {
                                n1139 = local read "LCounter"() -> (w358:dbl)
                                n1140 = Add(x=w358, y=1) -> (x+y=→"LCounter":dbl)
                                }
                              }
                            }
                          }
                          frame #1 {
                            n1141 = local write "LCounter"(0) -> ()
                          }
                        }
                      }
                    }
                    frame #2 {
                      n1142 = local write "LCounter"(0) -> ()
                    }
                  }
                }
              }
              "Numeric" <- w178
            }
            frame #2 {
              n1143 = local write "Insert"(FALSE) -> ()
            }
          }
        }
      }
    }
    n1144 = And(x=w59, y=w63) -> (x .and. y?=w64:bool)
    n1145 = case shown="True" w64 {
      frame False {
      }
      frame True {
        n1146 = local read "# of Spots"() -> (w403:dbl)
        n1147 = for {
          N: w403 -> [_]
          i -> [w405]
          stop <- w404 stop-if-true
          n1148 = local read "Selection/Group"() -> (w407:T7[])
          n1149 = Index Array(array=w407, index=w405) -> (element=w406:T7)
          n1150 = Unbundle By Name(w406) -> ("Selected"=w404:bool)
          n1151 = case shown="True" w404 {
            tunnel: w405 -> [_ w409]
            frame False {
            }
            frame True {
              n1152 = local write "Current Spot #"(w409) -> ()
              "Induce check" <- TRUE
            }
          }
        }
      }
    }
    n1153 = local read "spots selected"() -> (w74:i32)
    n1154 = local read "spots selected 2"() -> (w75:i32)
    n1155 = local read "Prev Current Spot"() -> (w83:dbl)
    n1156 = local read "Current Spot #"() -> (w84:dbl)
    n1157 = Not Equal?(x=w84, y=w83) -> (x != y?=w82:bool)
    n1158 = Greater?(x=w75, y=w74) -> (0:w76:bool)
    n1159 = local read "Induce check"() -> (w65:bool)
    n1160 = Or(x=w82, y=w76) -> (x .or. y?=w67:bool)
    n1161 = Or(x=w67, y=w65) -> (x .or. y?=w66:bool)
    n1162 = case shown="True" w66 {
      frame False {
      }
      frame True {
        n1163 = stacked-sequence {
          frame #0 {
            # "A small 100 ms delay is given to provide enough time for the data to be processed properly."
            n1164 = local read "Null array"() -> (w415:dbl[])
            n1165 = local write "What to Check"(w415) -> ()
            n1166 = local write "ID"(w415) -> ()
            n1167 = local read "Current Spot #"() -> (w417:dbl)
            n1168 = local write "Potential Collisions"(0) -> ()
            n1169 = local read "Spot Checker"() -> (w416:T1[])
            n1170 = Index Array(array=w416, index=w417) -> (element=w418:T1)
            n1171 = Wait (ms)(milliseconds to wait=10) -> ()  [unwired: 1 out]
            n1172 = Unbundle By Name(w418) -> ("Position.x"=w412:dbl, "Position.y"=w413:dbl)
            n1173 = local write "Orig Y SC"(w413) -> ()
            n1174 = local write "Orig X SC"(w412) -> ()
            n1175 = local write "Induce check"(FALSE) -> ()
          }
          frame #1 {
            n1176 = local read "# of Spots"() -> (w419:dbl)
            n1177 = for {
              N: w419 -> [_]
              tunnel: w419 -> [w424]
              i -> [w420]
              n1178 = local read "Selection/Group"() -> (w423:T7[])
              n1179 = Index Array(array=w423, index=w420) -> (element=w422:T7)
              n1180 = Unbundle By Name(w422) -> ("Selected"=w421:bool)
              n1181 = case shown="True" w421 {
                tunnel: w424 -> [_ w426]
                tunnel: w420 -> [_ w425]
                frame False {
                }
                frame True {
                  n1182 = for {
                    N: w426 -> [_]
                    tunnel: w425 -> [w427]
                    i -> [w428]
                    # "If the bubble is not selected, find difference of bubble to bubble\nbeing checked"
                    n1183 = local read "Selection/Group"() -> (w432:T7[])
                    n1184 = Index Array(array=w432, index=w428) -> (element=w431:T7)
                    n1185 = Unbundle By Name(w431) -> ("Selected"=w429:bool)
                    n1186 = Not(x=w429) -> (.not. x?=w430:bool)
                    n1187 = case shown="True" w430 {
                      tunnel: w428 -> [_ w436]
                      tunnel: w427 -> [_ w435]
                      tunnel: w427 -> [_ w434]
                      frame False {
                      }
                      frame True {
                        n1188 = local read "Spot Checker"() -> (w453:T1[])
                        n1189 = Index Array(array=w453, index=w436) -> (element=w454:T1)
                        n1190 = Index Array(array=w453, index=w435) -> (element=w452:T1)
                        n1191 = Unbundle By Name(w452) -> ("Position.x"=w449:dbl, "Position.y"=w445:dbl)
                        n1192 = Unbundle By Name(w454) -> ("Position.x"=w446:dbl, "Position.y"=w442:dbl)
                        n1193 = local read "Area+ Buffer"() -> (w433:dbl)
                        n1194 = Subtract(x=w449, y=w433) -> (x-y=w450:dbl)
                        n1195 = Greater Or Equal?(x=w446, y=w450) -> (x >= y?=w451:bool)
                        n1196 = Add(x=w445, y=w433) -> (x+y=w444:dbl)
                        n1197 = Subtract(x=w445, y=w433) -> (x-y=w443:dbl)
                        n1198 = Add(x=w449, y=w433) -> (x+y=w447:dbl)
                        n1199 = Less Or Equal?(x=w442, y=w444) -> (x <= y?=w441:bool)
                        n1200 = Greater Or Equal?(x=w442, y=w443) -> (x >= y?=w440:bool)
                        n1201 = Less Or Equal?(x=w446, y=w447) -> (x <= y?=w448:bool)
                        n1202 = And(x=w451, y=w448) -> (x .and. y?=w438:bool)
                        n1203 = And(x=w441, y=w440) -> (x .and. y?=w439:bool)
                        n1204 = And(x=w438, y=w439) -> (x .and. y?=w437:bool)
                        n1205 = case shown="True" w437 {
                          tunnel: w436 -> [_ _]
                          tunnel: w436 -> [_ w456]
                          tunnel: w434 -> [_ w455]
                          frame False {
                          }
                          frame True {
                            n1206 = stacked-sequence {
                              tunnel: w456 -> [w457 _]
                              tunnel: w455 -> [w458 _]
                              frame #0 {
                                n1207 = local read "Potential Collisions"() -> (w461:dbl)
                                n1208 = local read "What to Check"() -> (w462:dbl[])
                                n1209 = Insert Into Array(array=w462, index=w461, new element=w457) -> (w463:dbl[])
                                n1210 = local read "ID"() -> (w460:dbl[])
                                n1211 = local write "What to Check"(w463) -> ()
                                n1212 = Insert Into Array(array=w460, index=w461, new element=w458) -> (w459:dbl[])
                                n1213 = local write "ID"(w459) -> ()
                              }
                              frame #1 {
                                n1214 = local read "Potential Collisions"() -> (w466:dbl)
                                n1215 = Add(x=w466, y=1) -> (x+y=w464:dbl)
                                n1216 = local write "Potential Collisions"(w464) -> ()
                              }
                            }
                          }
                        }
                      }
                    }
                  }
                }
              }
            }
          }
          frame #2 {
            n1217 = local read "Current Spot #"() -> (w467:dbl)
            n1218 = local write "Prev Current Spot"(w467) -> ()
          }
        }
      }
    }
    n1219 = local read "Buffer Zone"() -> (w80:dbl)
    n1220 = Multiply(x=w80, y=2) -> (x*y=w81:dbl)
    n1221 = Add(x="Area to check", y=w81) -> (x+y=→"Area+ Buffer":dbl)
    n1222 = feedback #11() -> (w53:dbl)  [unwired: 1 in]
    n1223 = Equal?(x=w53, y=10000) -> (x = y?=w54:bool)
    n1224 = call "Elapsed Time"("Reset"=w54) -> ("Elapsed Time (s)"=w52:dbl, "Time has Elapsed"=w57:bool)  [unwired: 11 in, 6 out]
    "Elapsed Time" <- w52
    n1225 = feedback-in #11(w52) -> ()
    n1226 = And(x="On", y=w57) -> (x .and. y?=w58:bool)
    n1227 = case shown="True" w58 {
      frame False {
      }
      frame True {
        n1228 = local read "Position"() -> (w402:cluster{"x":dbl, "y":dbl, "z":dbl})
        n1229 = Unbundle By Name(w402) -> ("x"=→"X Pos every 10 sec":dbl)
      }
    }
    n1230 = case shown="True" "OK Button" {
      frame False {
      }
      frame True {
        n1231 = script code="clear all;\nclc;\n\ng = gigecam('169.254.154.83');\n\ng.PixelFormat= 'BayerGR8'\n\nimg = snapshot(g);\n\nimshow(img);"() -> ()  [unwired: 1 in, 1 out]
      }
    }
    n1232 = case shown="True" "O Button" {
      frame False {
      }
      frame True {
        n1233 = script code="%\n    rslt = Hough1_data(img);\n\n    % Frame translation\n    %- omit this as of now \n    \n    % Control method\n    increment = 10; %assuming the diamiter of the agent around 20 pic \n    \n    %- NewLoc = [x,y] whose unit is px\n    %- update new location based on current location obtained by the camera\n    NewLoc(1)= rslt(1);\n    NewLoc(2)= rslt(2);\n    \n    \n    % Update microrobot location with NewLoc\n    % the single robot would move to oblique downword\n    \n    % wait seconds"() -> ("NewLoc"=w398:dbl[])  [unwired: 1 in, 1 out]
        n1234 = Index Array(array=w398, index=1) -> (element=→"Y":dbl)
        n1235 = Index Array(array=w398, index=0) -> (element=→"X":dbl)
      }
    }
    "Rates" <- w34
    "LCS" <- w34
  }
  n1236 = flat-sequence {
    tunnel: w6 -> [w1937]
    tunnel: w5 -> [w1936]
    tunnel: [w1935] -> w3
    frame #0 {
      n1237 = disable-structure shown="\"IMAQdx with ROI tool buttons (default)\"" {
        disable-tunnel: w1937 -> [_ _ _ _ _ _]
        disable-tunnel: w1936 -> [_ _ w1995 _ _ _]
        disable-tunnel: [_ _ w1994 _ _ _] -> w1935
        frame condition #0 {
          w1939 = u32 10 ("Number of buffers")
          (unwired) FALSE ("background subtraction")
          # "This subdiagram uses the IMAQ drivers, with a pre-allocated ringbuffer for images.  This is the code I use with my Mikrotron MC1362-CL"
          n1238 = call <vilib>:"IMAQ Init.vi"("Interface Name"="img0") -> ("IMAQ Session Out"=w1946:refnum<k11>)  [unwired: 9 in, 1 out]
          n1239 = call <vilib>:"IMAQ Configure List.vi"("Region of interest"="Global ROI (requires restart)", "Number of buffers"=w1939, "Continuous?"=enum16{"One-Shot", "Continuous"}."Continuous", "IMAQ Session In"=w1946) -> ("error out"=w1940:errorcluster, "IMAQ Session Out"=w1942:refnum<k11>)  [unwired: 6 in]
          n1240 = for {
            N: w1939 -> [_]
            tunnel: 0 ("Channel") -> [w1959]
            shift-right: [w1962] -> w1944
            shift-left: w1940 -> [w1958]
            shift-right: [w1961] -> w1943
            shift-left: w1942 -> [w1960]
            i -> [w1957]
            n1241 = Format Into String(format string="mikrotronbuffer%04d", w1957) -> (resulting string=w1955:string)  [unwired: 2 in, 1 out]
            n1242 = call "IMAQ Create"("Image Name"=w1955) -> ("New Image"=w1954:T8)  [unwired: 4 in, 1 out]
            n1243 = call <vilib>:"IMAQ Configure Buffer.vi"("Channel"=w1959, "error in (no error)"=w1958, "Buffer Number"=w1957, "Image In"=w1954, "IMAQ Session In"=w1960) -> ("error out"=w1962:errorcluster, "IMAQ Session Out"=w1961:refnum<k11>)  [unwired: 5 in]
          }
          n1244 = call <vilib>:"IMAQ Start.vi"("error in (no error)"=w1944, "IMAQ Session In"=w1943) -> ("error out"=w1950:errorcluster, "IMAQ Session Out"=w1951:refnum<k11>)  [unwired: 8 in]
          n1245 = call "IMAQ Create"("Image Name"="Red Tweezers live image") -> ("New Image"=w1952:T8)  [unwired: 3 in, 2 out]
          n1246 = while {
            tunnel: w1951 -> [w1970]
            tunnel: w1950 -> [w1969]
            tunnel: w1952 -> [_]
            tunnel: [w1971] -> w1948
            tunnel: [w1964] -> w1949
            i -> [w1966]
            stop <- w1972 stop-if-true
            n1247 = local read "stop"() -> (w1972:bool)
            n1248 = call <vilib>:"IMAQ Extract Buffer.vi"("error in (no error)"=w1969, "Buffer to extract"=w1966, "IMAQ Session In"=w1970) -> ("error out"=w1964:errorcluster, "Image Out"=w1963:T8, "IMAQ Session Out"=w1971:refnum<k11>)  [unwired: 3 in, 3 out]
            n1249 = call "imageQ_camera_hook.vi"("Image"=w1963) -> ()  [unwired: 11 in]
            n1250 = feedback #12() -> (w1967:T26)  [unwired: 1 in]
            n1251 = call "Smoothed Frame Rate.vi"("Feedback In"=w1967) -> ("Feedback Out"=w1968:T26, "Frame Rate"=w1965:dbl)  [unwired: 1 in, 4 out]
            n1252 = feedback-in #12(w1968) -> ()
            n1253 = global write "red_tweezers_globals_INTERNAL_VOLATILE.vi" "Video Frame Rate"(w1965) -> ()
          }
          n1254 = call <vilib>:"IMAQ Close.vi"("error in (no error)"=w1949, "IMAQ Session In"=w1948) -> ()  [unwired: 9 in, 1 out]
        }
        frame condition #1 {
          (unwired) FALSE ("background subtraction")
          # "This subdiagram acquires using the IMAQdx drivers.  This covers most FireWire and GigE cameras (at least the ones supporting the IIDC or GenICam standards)."
          n1255 = call <vilib>:"IMAQdx Open Camera.vi"("Session In"=T6 "dalsaGenie") -> ("error out"=w1975:errorcluster, "Session Out"=w1974:T6)  [unwired: 9 in]
          n1256 = call <vilib>:"IMAQdx Configure Grab.vi"("error in"=w1975, "Session In"=w1974) -> ("error out"=w1976:errorcluster, "Session Out"=w1977:T6)  [unwired: 8 in]
          n1257 = call "IMAQ Create"("Image Name"="Red Tweezers live image") -> ("New Image"=w1980:T8)  [unwired: 3 in, 2 out]
          n1258 = while {
            tunnel: w1977 -> [w1989]
            tunnel: w1976 -> [w1988]
            tunnel: w1980 -> [w1982]
            tunnel: [w1990] -> w1978
            tunnel: [w1984] -> w1979
            stop <- w1991 stop-if-true
            n1259 = local read "stop"() -> (w1991:bool)
            n1260 = call <vilib>:"IMAQdx Grab.vi"("error in"=w1988, "Image In"=w1982, "Session In"=w1989) -> ("error out"=w1984:errorcluster, "Image Out"=w1983:T8, "Session Out"=w1990:T6)  [unwired: 5 in, 1 out]
            n1261 = call "imageQ_camera_hook.vi"("Image"=w1983) -> ()  [unwired: 11 in]
            n1262 = feedback #13() -> (w1986:T26)  [unwired: 1 in]
            n1263 = call "Smoothed Frame Rate.vi"("Feedback In"=w1986) -> ("Feedback Out"=w1987:T26, "Frame Rate"=w1985:dbl)  [unwired: 1 in, 4 out]
            n1264 = feedback-in #13(w1987) -> ()
            n1265 = global write "red_tweezers_globals_INTERNAL_VOLATILE.vi" "Video Frame Rate"(w1985) -> ()
          }
          n1266 = call <vilib>:"IMAQdx Close Camera.vi"("error in"=w1979, "Session In"=w1978) -> ()  [unwired: 9 in, 1 out]
        }
        frame condition #2 {
          # "This subdiagram acquires using the IMAQdx drivers.  This covers most FireWire and GigE cameras (at least the ones supporting the IIDC or GenICam standards)."
          n1267 = call <vilib>:"IMAQdx Open Camera.vi"("Session In"="Camera") -> ("error out"=w2003:errorcluster, "Session Out"=w2002:T6)  [unwired: 9 in]
          n1268 = call <vilib>:"IMAQdx Configure Grab.vi"("error in"=w2003, "Session In"=w2002) -> ("error out"=w1999:errorcluster, "Session Out"=w2000:T6)  [unwired: 8 in]
          n1269 = call "IMAQ Create"("Image Name"="Red Tweezers live image") -> ("New Image"=w1997:T8)  [unwired: 3 in, 2 out]
          n1270 = call "IMAQdx_get_ROI.vi"("Session In"=w2000) -> ("ROI"=w1996:u32[], "Session Out"=w1998:T6)  [unwired: 8 in]
          n1271 = while {
            shift-right: [w2012] -> w1992
            shift-left: w1999 -> [w2013]
            shift-right: [w2009] -> w1993
            shift-left: w1998 -> [w2010]
            tunnel: w1997 -> [w2008]
            tunnel: w1996 -> [w2007]
            tunnel: w1995 -> [w2006]
            tunnel: [w2005] -> w1994
            stop <- w2019 stop-if-true
            n1272 = event shown="[0] Timeout" {
              selector: _ -> [_ _ _]
              dyn-events: _ -> [_ _ _]
              timeout: 0 -> [_ _ _]
              tunnel: w2013 -> [w2026 w2033 w2048]
              tunnel: [w2025 w2033 w2048] -> w2012
              tunnel: w2010 -> [w2024 w2034 w2049]
              tunnel: [w2023 w2034 w2049] -> w2009
              tunnel: w2008 -> [w2022 _ _]
              tunnel: w2007 -> [w2021 _ _]
              tunnel: w2006 -> [_ w2032 w2047]
              event Timeout {
                w2020 = 0  # timeout in ms
                # "Use a timeout of a few hundred ms if you want to acquire just fast enough to update the image- or a timeout of zero to run the camera at full speed."
                # "This VI sends the image to the loop above for display.\nIt's better to do this than to display here, because it separates the camera loop from the front panel a bit, and increases speed without sacrificing responsiveness of the UI.  Of course, using the event structure removes some of those benefits- but it is possible to write a high-performance camera loop with fast particle tracking, and still use this mechanism to display images without slowing down acquisition."
                # "If we're not dealing with other events, acquire from the camera."
                n1273 = event-data() -> ("Time"=w2031:u32)  [unwired: 1 in]
                n1274 = call <vilib>:"IMAQdx Grab.vi"("error in"=w2026, "Image In"=w2022, "Session In"=w2024) -> ("error out"=w2025:errorcluster, "Image Out"=w2028:T8, "Session Out"=w2023:T6)  [unwired: 5 in, 1 out]
                n1275 = call "IMAQ Clear Overlay"("Image"=w2028) -> ("Image Out"=w2027:T8)  [unwired: 9 in, 1 out]
                n1276 = Multiply(x=w2031, y=u32 1000) -> (x*y=w2029:u32)
                n1277 = call "imageQ_camera_hook.vi"("timeout in ms (0=don't wait if there are no requests)"=w2020, "Timestamp/us"=w2029, "ROI"=w2021, "Image"=w2027) -> ()  [unwired: 8 in]
              }
              event "Draw ROI", "Zoom": Value Change {
                # "This changes the current mouse mode on the image, allowing zooming/drawing of ROI (which can be useful if you want to window down a camera for particle tracking)."
                n1278 = event-data() -> ("CtlRef"=w2039:refnum<vi>)  [unwired: 1 in]
                n1279 = control-ref of="Draw ROI"() -> (w2040:refnum<vi>)
                n1280 = Equal?(x=w2040, y=w2039) -> (x = y?=w2038:bool)
                n1281 = case shown="True" w2038 {
                  tunnel: [w2043 w2046] -> w2037
                  tunnel: [TRUE ("stop") FALSE ("stop")] -> w2035
                  tunnel: [FALSE ("Update Indicators?") TRUE ("Update Indicators?")] -> w2036
                  frame False {
                    w2043 = u32 8 items=["Zoom Tool"=8, "Selection Tool"=0, "Pan Tool"=9, "Point Tool"=1, "Line Tool"=2, "Rectangle Tool"=3, "Rotated Rectangle Tool"=12, "Polyline Tool"=10, "Polygon Tool"=5, "Freehand Tool"=11, "Closed Freehand Tool"=6, "Ellipse Tool"=4, "Annulus Tool"=7] ("Current ROI Tool")
                  }
                  frame True {
                    w2046 = u32 3 items=["Zoom Tool"=8, "Selection Tool"=0, "Pan Tool"=9, "Point Tool"=1, "Line Tool"=2, "Rectangle Tool"=3, "Rotated Rectangle Tool"=12, "Polyline Tool"=10, "Polygon Tool"=5, "Freehand Tool"=11, "Closed Freehand Tool"=6, "Ellipse Tool"=4, "Annulus Tool"=7] ("Current ROI Tool")
                  }
                }
                n1282 = local write "Draw ROI"(w2036) -> ()
                n1283 = local write "Zoom"(w2035) -> ()
                n1284 = property on="Property Node" class="ImageControl"(reference=w2032, "Current ROI Tool"=w2037) -> ()  [unwired: 1 in, 2 out]
              }
              event "Zoom to Fit": Value Change {
                # "The various ROI tools are hidden, so the image control resizes nicely as the Red Tweezers window is resized.  The zoom to fit button/mouse mode buttons return some of this functionality."
                n1285 = event-data() -> ("NewVal"=w2050:bool)  [unwired: 1 in]
                n1286 = property on="Property Node" class="ImageControl"(reference=w2047, "Zoom to Fit Mode"=w2050) -> ()  [unwired: 1 in, 2 out]
              }
            }
            n1287 = feedback #14() -> (w2018:T26)  [unwired: 1 in]
            n1288 = call "Smoothed Frame Rate.vi"("Feedback In"=w2018, "Alpha"=0.05) -> ("Feedback Out"=w2017:T26, "Frame Rate"=w2014:dbl)  [unwired: 4 out]
            n1289 = feedback-in #14(w2017) -> ()
            n1290 = global write "red_tweezers_globals_INTERNAL_VOLATILE.vi" "Video Frame Rate"(w2014) -> ()
            n1291 = local read "stop"() -> (w2015:bool)
            n1292 = Unbundle By Name(w2012) -> ("status"=w2005:bool)
            n1293 = Or(x=w2005, y=w2015) -> (x .or. y?=w2019:bool)
          }
          n1294 = call <vilib>:"IMAQdx Close Camera.vi"("error in"=w1992, "Session In"=w1993) -> ()  [unwired: 9 in, 1 out]
        }
        frame condition #3 (active) {
          w2052 = 0 ("element")
          w2054 = 1920 ("dimension size")
          w2053 = 1080 ("dimension size")
          w2055 = T15 0 items=["Grayscale (U8)", "Grayscale (I16)", "Grayscale (SGL)", "Complex (CSG)", "RGB (U32)", "HSL (U32)", "RGB (U64)", "Grayscale (U16)"] ("Image Type")
          (unwired) FALSE ("background subtraction")
          # "This subdiagram generates a blank white image- useful if you don't have a camera"
          n1295 = Build Array(w2052, w2052, w2054, w2053) -> (w2051:i32[])
          n1296 = Initialize Array(u8 255 ("element"), w2053, w2054) -> (w2056:u8[][])
          n1297 = global write "red_tweezers_globals_INTERNAL.vi" "Global ROI"(w2051) -> ()
          n1298 = call "IMAQ Create"("Image Name"="red tweezers camera stub", "Image Type"=w2055) -> ("New Image"=w2057:T8)  [unwired: 2 in, 2 out]
          n1299 = call "IMAQ ArrayToImage"("Image Pixels (U8)"=w2056, "Image"=w2057) -> ("Image Out"=w2060:T8)  [unwired: 8 in, 1 out]
          n1300 = call "IMAQ Create"("Image Name"="Red Tweezers live image") -> ("New Image"=w2061:T8)  [unwired: 3 in, 2 out]
          n1301 = while {
            tunnel: w2060 -> [w2064]
            tunnel: w2061 -> [_]
            stop <- w2068 stop-if-true
            n1302 = local read "stop"() -> (w2068:bool)
            n1303 = Wait Until Next ms Multiple(millisecond multiple=u32 20) -> ()  [unwired: 1 out]
            n1304 = call "imageQ_camera_hook.vi"("Image"=w2064) -> ()  [unwired: 11 in]
            n1305 = feedback #15() -> (w2066:T26)  [unwired: 1 in]
            n1306 = call "Smoothed Frame Rate.vi"("Feedback In"=w2066) -> ("Feedback Out"=w2067:T26, "Frame Rate"=w2065:dbl)  [unwired: 1 in, 4 out]
            n1307 = feedback-in #15(w2067) -> ()
            n1308 = global write "red_tweezers_globals_INTERNAL_VOLATILE.vi" "Video Frame Rate"(w2065) -> ()
          }
        }
        frame condition #4 {
          # "Use this subdiagram if you have an external camera VI which writes to the image queue (using imageQ_camera_hook.vi)"
        }
        frame condition #5 {
          w2069 = path "C:/Users/Tweezer Cube/Desktop/red_tweezers_1_4_rc0/camera_for_rt136.llb/Particle Tracking.vi"  # Path to camera VI
          # "Use this subdiagram if you have an external camera VI which writes to the image queue (using imageQ_camera_hook.vi).  This is the slightly more sophisticated version, which checks that said external VI is running, and runs it if not."
          n1309 = Open VI Reference(vi path=w2069) -> (vi reference=w2070:refnum<vi>, error out=w2072:errorcluster)  [unwired: 5 in]
          n1310 = property class="VI"(reference=w2070) -> ("Path"=w2071:path)  [unwired: 1 in, 2 out]
          n1311 = global write "red_tweezers_globals_INTERNAL_VOLATILE.vi" "Current Camera VI"(w2071) -> ()
          n1312 = property class="VI"(reference=w2070, error in=w2072) -> (reference out=w2077:refnum<vi>, error out=w2076:errorcluster, "Exec.State"=w2074:T28)
          n1313 = Equal?(x=w2074, y=T28."Idle") -> (x = y?=w2078:bool)
          n1314 = case shown="True" w2078 {
            tunnel: w2077 -> [w2082 w2091]
            tunnel: w2076 -> [w2081 w2088]
            tunnel: [w2080 w2087] -> w2073
            tunnel: w2074 -> [w2084 _]
            frame False {
              n1315 = Close Reference(reference=w2082, error in (no error)=w2081) -> (error out=w2080:errorcluster)
              n1316 = Equal?(x=w2084, y=T28."Bad") -> (x = y?=w2083:bool)
              n1317 = case shown="False" w2083 {
                frame False {
                }
                frame True {
                  n1318 = One Button Dialog(message="The external camera VI is not running and cannot be started- it's probably broken or missing.  Check the static/dynamically loaded VI reference in the bottom loop on the block diagram.") -> ()  [unwired: 1 in, 1 out]
                }
              }
            }
            frame True {
              n1319 = invoke class="VI" method="Run VI"(reference=w2091, error in=w2088, "Wait until done"=FALSE ("Wait Until Done"), "Auto Dispose Ref"=TRUE ("Auto Dispose Reference")) -> (error out=w2087:errorcluster)  [unwired: 1 in, 4 out]
            }
          }
          n1320 = call <vilib>:"Simple Error Handler.vi"("error source (\" \")"="External camera VI (see the bottom loop in the block diagram)" ("error source (\" \")"), "error in (no error)"=w2073) -> ()  [unwired: 3 in, 5 out]
        }
      }
    }
  }
  n1321 = while {
    tunnel: w9 -> [w2109]
    shift-right: [w2108] -> w8
    shift-left: w10 -> [w2110]
    shift-right: [w2105] -> _
    shift-left: _ -> [w2098]
    shift-right: [w2104] -> _
    shift-left: _ -> [w2102]
    shift-right: [w2103] -> _
    shift-left: FALSE ("Saving") -> [w2099]
    stop <- w2107 stop-if-true
    w2096 = u32 50 ("millisecond multiple")
    # "Start/stop saving data, if necessary"
    n1322 = Divide(x=u32 1000, y=w2096) -> (x/y=w2094:dbl)
    n1323 = Wait Until Next ms Multiple(millisecond multiple=w2096) -> ()  [unwired: 1 out]
    n1324 = call "imageQ_dequeue.vi"("timeout in ms (-1)"=2000, "Return queue"=w2110, "Image Dst"=w2109) -> ("Timestamp/us"=w2100:u64, "Return queue out"=w2108:refnum<queue>, "Image Dst Out"=w2111:T8, "timed out?"=w2114:bool, "ROI"=w2093:u64[])  [unwired: 4 in]
    n1325 = Not(x=w2114) -> (.not. x?=w2112:bool)
    n1326 = case shown="True" w2112 {
      tunnel: w2111 -> [_ w2148]
      tunnel: w2102 -> [w2141 w2151]
      tunnel: w2099 -> [_ w2145]
      tunnel: [w2141 w2146] -> w2101
      tunnel: w2100 -> [_ w2149]
      tunnel: w2098 -> [w2142 w2150]
      tunnel: [w2142 w2147] -> w2097
      tunnel: w2093 -> [_ w2144]
      frame False {
      }
      frame True {
        n1327 = global read "red_tweezers_globals_INTERNAL.vi" "Image Overlay (extras from control loop)"() -> (w2159:T18[])
        n1328 = case shown="True" w2145 {
          tunnel: w2151 -> [w2160 w2162]
          tunnel: w2150 -> [w2161 w2168]
          tunnel: w2149 -> [_ w2167]
          tunnel: w2148 -> [_ w2166]
          tunnel: [w2161 w2165] -> w2147
          tunnel: [w2160 w2164] -> w2146
          frame False {
          }
          frame True {
            n1329 = call "save_data_save.vi"("Image"=w2166, "Timestamp"=w2167, "Avi Refnum"=w2162, "Data refnum"=w2168) -> ("error out"=w2163:errorcluster, "Avi Refnum (duplicate)"=w2164:T29, "Data refnum (duplicate)"=w2165:refnum<file>)  [unwired: 5 in]
            n1330 = case shown="Error" w2163 {
              selector: w2163 -> [_ w2170]
              frame No Error {
              }
              frame Error {
                n1331 = call <vilib>:"Clear Errors.vi"("error in (no error)"=w2170) -> ()  [unwired: 5 in, 2 out]
                n1332 = local write "Save Video"(FALSE ("Save")) -> ()
              }
            }
          }
        }
        n1333 = global write "red_tweezers_globals_INTERNAL.vi" "Global ROI"(w2144) -> ()
        n1334 = global read "red_tweezers_globals_INTERNAL_VOLATILE.vi" "Tracked Spot Positions (3D)"() -> (w2152:cluster{"x":dbl, "y":dbl, "Z":dbl}[])
        n1335 = global read "red_tweezers_globals.vi" "Selection/Group"() -> (w2158:T7[])
        n1336 = global read "red_tweezers_globals.vi" "Spots"() -> (w2157:T1[])
        n1337 = call "overlay_positions.vi"("Positions"=w2152, "Image"=w2148) -> ("Image 2"=w2154:T8)  [unwired: 9 in]
        n1338 = call "render_overlay_elements.vi"("Image Overlay (extras from control loop)"=w2159, "Image"=w2154) -> ("Image Out"=w2156:T8)  [unwired: 5 in]
        n1339 = call "grid_and_guides.vi"("Operation"=T12."Render on image", "Image"=w2156) -> ("Image Out"=w2143:T8)  [unwired: 9 in]
        n1340 = call "overlay_spots_on_image.vi"("Selection and Groups"=w2158, "Spots"=w2157, "image"=w2143) -> ("Image"=→"Image":T8)  [unwired: 3 in, 1 out]
      }
    }
    n1341 = global read "red_tweezers_globals_INTERNAL_VOLATILE.vi" "Video Frame Rate"() -> (→"Video Frame Rate":dbl)
    n1342 = case shown="True" "Save Video" {
      tunnel: [w2117 w2132] -> w2105
      tunnel: [w2116 w2126] -> w2104
      tunnel: [FALSE ("Saving") w2131] -> w2103
      tunnel: w2099 -> [w2120 w2130]
      tunnel: w2101 -> [w2118 w2129]
      tunnel: w2097 -> [w2119 w2128]
      tunnel: w2094 -> [_ w2127]
      frame False {
        n1343 = case shown="True" w2120 {
          tunnel: w2119 -> [w2122 w2125]
          tunnel: w2118 -> [w2121 w2124]
          tunnel: [w2122 _] -> w2117
          tunnel: [w2121 _] -> w2116
          frame False {
          }
          frame True {
            n1344 = local write "Save Video"(FALSE ("Save")) -> ()
            n1345 = call "save_data_stop.vi"("Avi Refnum"=w2124, "Data refnum"=w2125) -> ()  [unwired: 10 in]
          }
        }
      }
      frame True {
        n1346 = case shown="False" w2130 {
          selector: w2130 -> [_ w2140]
          tunnel: [w2137 w2138] -> w2132
          tunnel: [w2136 w2139] -> w2126
          tunnel: [w2133 w2140] -> w2131
          tunnel: w2129 -> [_ w2139]
          tunnel: w2128 -> [_ w2138]
          tunnel: w2127 -> [w2135 _]
          frame False {
            n1347 = call "save_data_start.vi"("Save Video"=TRUE, "Frames Per Second"=w2135) -> ("Saving"=w2133:bool, "Avi Refnum"=w2136:T29, "Data Refnum"=w2137:refnum<file>)  [unwired: 3 in]
            n1348 = local write "Save Video"(w2133) -> ()
          }
          frame True {
          }
        }
      }
    }
    n1349 = local read "stop"() -> (w2107:bool)
  }
  n1350 = Release Queue(queue=w8) -> ()  [unwired: 2 in, 3 out]
  n1351 = case shown="True" w3 {
    frame False {
    }
    frame True {
      n1352 = One Button Dialog(message="Warning: there was a camera error.  You may need to restart Red Tweezers.") -> ()  [unwired: 1 in, 1 out]
    }
  }
  n1353 = flat-sequence {
    tunnel: w18 -> [w2176]
    tunnel: w17 -> [_]
    frame #0 {
      # "This autosaves when we stop.  The sequence structures are necessary so that:\n1. loading settings doesn't stop the VI\n2. plugins are still open (and hence saved) when we save settings"
      n1354 = local read "Plugins"() -> (w2179:T3)
      n1355 = global read "red_tweezers_globals_INTERNAL_VOLATILE.vi" "Current Settings File"() -> (w2173:path)
      n1356 = global read "red_tweezers_globals_INTERNAL_VOLATILE.vi" "Save Settings On Exit"() -> (w2172:bool)
      n1357 = flat-sequence {
        tunnel: w2176 -> [w2182]
        tunnel: [w2182] -> w2175
        frame #0 {
          n1358 = local write "stop"(FALSE ("STOP")) -> ()
        }
      }
      n1359 = case shown="True" w2172 {
        tunnel: w2173 -> [_ w2187]
        tunnel: w2175 -> [w2184 w2185]
        tunnel: [w2184 w2185] -> w2174
        frame False {
        }
        frame True {
          n1360 = Path To String(path=w2187) -> (string=w2186:string)
          n1361 = call "settings_save_to_file.vi"("XML File Path"=w2187) -> ()  [unwired: 11 in]
          n1362 = call "settings_filename_to_registry.vi"("Last Used Settings File"=w2186) -> ()  [unwired: 11 in]
        }
      }
      n1363 = flat-sequence {
        tunnel: w2174 -> [w2180]
        tunnel: [w2180] -> _
        frame #0 {
          n1364 = local write "stop"(TRUE ("STOP")) -> ()
        }
      }
      n1365 = control-ref of="Plugin Pnl"() -> (w2177:refnum<vi>)
      n1366 = control-ref of="Plugin:"() -> (w2178:refnum<vi>)
      n1367 = call "plugins_unload.vi"("error in (no error)"=w2174, "Plugins"=w2179, "Sub Panel"=w2177, "Plugin Chooser"=w2178) -> ()  [unwired: 2 in, 2 out]
    }
  }
